vi "Periodic Tasks.vi"(8 "error in":errorcluster) -> ()   [LabVIEW 2023]
doc: "This VI runs in parallel to other tasks. It can contain as many user-defined periodic loops as you need. These can carry out PID or other sorts of timed response."
uses:
  <vilib>/Rock Robotics/WPI/DriverStation/WPI_DriverStationAllianceInfo.ctl
  <vilib>/Rock Robotics/WPI/DriverStation/WPI_DriverStationRobotMode2.ctl
  <vilib>/Rock Robotics/WPI/ThirdParty/JAS_Junk/TrajLib/TypeDef/TRANSLATION3D.ctl
  <vilib>/Rock Robotics/WPI/ThirdParty/JAS_Junk/TrajLib/TypeDef/POSE2D.ctl
  <vilib>/Rock Robotics/WPI/ThirdParty/JAS_Junk/TrajLib/TypeDef/TRANSLATION2D.ctl
  <vilib>/Rock Robotics/WPI/ThirdParty/JAS_Junk/TrajLib/TypeDef/ROTATION2D.ctl
  <vilib>/Rock Robotics/WPI/ThirdParty/JAS_Junk/TrajLib/TypeDef/X_Y_PAIR.ctl
  e9f6a02a-451a-49ef-b810-556ee57ecbaa.vi
  d07e73b9-761c-4664-be59-ebf116924375.vi
  <vilib>/Rock Robotics/WPI/ThirdParty/JAS_Junk/TrajLib/VI/BoolCmd_Recv_Internal.vi
  <vilib>/Rock Robotics/WPI/ThirdParty/JAS_Junk/TrajLib/VI/BoolCmd_Send_Internal.vi
  <vilib>/Rock Robotics/WPI/ThirdParty/JAS_Junk/TrajLib/VI/Util_GetTime_U32.vi
  <vilib>/Rock Robotics/WPI/ThirdParty/JAS_Junk/TrajLib/Translation2d_UnaryMinus.vi
  <vilib>/Rock Robotics/WPI/ThirdParty/JAS_Junk/TrajLib/Rotation2d_UnaryMinus.vi
  <vilib>/Rock Robotics/WPI/ThirdParty/JAS_Junk/TrajLib/Translation2d_RotateBy.vi
  <vilib>/Rock Robotics/WPI/ThirdParty/JAS_Junk/TrajLib/MathUtil_InputModulus.vi
  <vilib>/Rock Robotics/WPI/ThirdParty/JAS_Junk/TrajLib/Rotation2d_GetRadians.vi
  <vilib>/Rock Robotics/WPI/ThirdParty/JAS_Junk/TrajLib/MathUtil_Clamp.vi
  <vilib>/Rock Robotics/WPI/ThirdParty/JAS_Junk/TrajLib/VI/BoolCmd_ObtainQueue.vi
  <vilib>/Rock Robotics/WPI/ThirdParty/JAS_Junk/TrajLib/Rotation2d_CreateXY.vi
  <vilib>/Rock Robotics/WPI/Utilities/WPI_GetSetVariantRefNum.vi
  <vilib>/Rock Robotics/WPI/ThirdParty/JAS_Junk/TrajLib/VI/Util_GetTime_U64.vi
  <vilib>/Rock Robotics/Network Tables/NT Write Number.vi
  Swerve_Drive_System/SWERVE_DRIVE_GLOBALS.vi
  <vilib>/Rock Robotics/Network Tables/NT Read Numeric Array.vi
  <vilib>/Rock Robotics/Network Tables/NT Read String.vi
  Robot Global Data.vi
  <vilib>/Rock Robotics/Network Tables/NT Write String.vi
  <vilib>/Rock Robotics/Network Tables/NT Write Boolean.vi
  <vilib>/Rock Robotics/Network Tables/NT Write String Array.vi
  <vilib>/Rock Robotics/Network Tables/NT Write Numeric Array.vi
  <vilib>/addons/control/pid/pid.llb/PID Control Input Filter (DBL).vi
  <vilib>/Rock Robotics/Network Tables/NT Read String Array.vi
  <vilib>/Rock Robotics/Network Tables/NT Read Boolean.vi
  <vilib>/Rock Robotics/Network Tables/NT Read Number.vi
  <vilib>/gmath/interp.llb/Search Ordered Table.vi
  <vilib>/Rock Robotics/WPI/ThirdParty/Phoenix-LabVIEW/Motor Controller/Get/CTRE_Phoenix_MotorController_GetSelectedSensorData.vi
  <vilib>/Rock Robotics/WPI/ThirdParty/JAS_Junk/TrajLib/Trajectory_Library.lvlib
  <vilib>/Rock Robotics/WPI/ThirdParty/Phoenix-LabVIEW/Motor Controller/Controls/CTRE_Phoenix_MotorControl_ControlMode.ctl
  <vilib>/Rock Robotics/WPI/ThirdParty/JAS_Junk/TrajLib/Enum/DCMOTOR_TYPES_ENUM.ctl
  <vilib>/Rock Robotics/WPI/ThirdParty/REV Robotics/REVLib/Typedef/Spark MAX Control Type.ctl
  <vilib>/Rock Robotics/WPI/ThirdParty/Phoenix-LabVIEW/Motor Controller/Get/CTRE_Phoenix_MotorController_GetTemperature.vi
  <vilib>/Rock Robotics/WPI/ThirdParty/Phoenix-LabVIEW/CANdle/Controls/CTRE_Phoenix_CANdle_LEDColor.ctl
  <vilib>/addons/control/pid/NI_PID_pid.lvlib
  a548ba9f-81d9-431c-be79-d7e9cbcd1e66.vi
  <vilib>/Rock Robotics/WPI/ThirdParty/Phoenix-LabVIEW/Motor Controller/Controls/CTRE_Phoenix_MotorControl_NeutralMode.ctl
  <vilib>/Rock Robotics/Network Tables/NT Write Boolean Array.vi
  <vilib>/Rock Robotics/WPI/ThirdParty/Phoenix-LabVIEW/CANCoder/Get/CTRE_Phoenix_CANcoder_GetSensorData.vi
  <vilib>/Rock Robotics/Network Tables/NT Write Variant.vi
  <vilib>/Rock Robotics/Network Tables/NT Read Variant.vi
  <vilib>/Rock Robotics/WPI/ThirdParty/REV Robotics/REVLib/SubVI/Public/SPARK Get Device Status Applied Output.vi
  <vilib>/Rock Robotics/WPI/ThirdParty/REV Robotics/REVLib/SubVI/Public/SPARK Get Encoder Status Position.vi
  <vilib>/Rock Robotics/WPI/ThirdParty/REV Robotics/REVLib/SubVI/Public/SPARK Get Encoder Status Velocity.vi
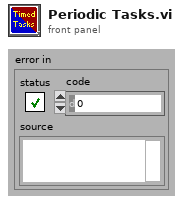
[diagram p1: front panel]
types:
  T1 = typedef "CTRE_Phoenix_CANdle_LEDColor.ctl" = cluster{"Red":u8, "Green":u8, "Blue":u8, "White":u8}
  T2 = typedef "WPI_DriverStationRobotMode2.ctl" = enum16{"Autonomous Disabled", "Autonomous Enabled", "Teleop Disabled", "Teleop Enabled", "Disconnected", "Finish", "Test Disabled", "Test Enabled", "Emergency Stopped"}
  T3 = typedef "CTRE_Phoenix_CANdle_DeviceRef.ctl" = cluster{"DeviceStatus":errorcluster, "Device Number":u8, "Handle":u64, "UsageFrame":u32, "Library Path":path}
  T4 = typedef "Trajectory_Library.lvlib/X_Y_PAIR.ctl" = cluster{"X":dbl, "Y":dbl}
  T5 = typedef "Trajectory_Library.lvlib/FUNCTION_GENERATOR.ctl" = cluster{"Table Xs":dbl[], "Table Ys":dbl[], "MinX":dbl, "MaxX":dbl, "ItemCount":i32}
  T6 = typedef "PathPlanner24.lvlib/PathPlannerEventMarker.ctl" = cluster{"WaypointRelativePos":dbl, "minimumTriggerDistance":dbl, "markerPos":T7, "lastRobotPos":T7, "Command":T8, "markerPos Exists":bool, "LastRobotPoseExists":bool, "Triggered":bool}
  T7 = typedef "Trajectory_Library.lvlib/TRANSLATION2D.ctl" = cluster{"X":dbl, "Y":dbl}
  T8 = typedef "PathPlanner24.lvlib/PathPlannerCommandUtil.ctl" = cluster{"waitTime":dbl, "name":string, "pathName":string, "commands":cluster{"type":T9, "waitTime":dbl, "name":string, "pathName":string}[], "type":T9}
  T9 = typedef "PathPlanner24.lvlib/PathPlanner_CommandUtilType_ENUM.ctl" = enum16{"Unknown", "Wait", "Named", "Path", "Sequential", "Parallel", "Race", "Deadline"}
  T10 = typedef "WPI_JoystickDevRef.ctl" = cluster{"Device":T11}
  T11 = typedef "WPI_JoystickDeviceEnum.ctl" = enum16{"USB 0", "USB 1", "USB 2", "USB 3", "USB 4", "USB 5"}
  T12 = typedef "Trajectory_Library.lvlib/SWERVE_DRIVE_KINEMATICS.ctl" = cluster{"NumModules":i32, "InverseKinematics":T13, "ForwardKinematics":T13, "Modules":T7[], "PrevCoR":T7, "SavedModuleStates":T14[]}
  T13 = typedef "NI_Matrix.lvlib/RealMatrix.ctl" = dbl[][]
  T14 = typedef "Trajectory_Library.lvlib/SWERVE_DRIVE_MODULE_STATE.ctl" = cluster{"Speed":dbl, "Angle":T15}
  T15 = typedef "Trajectory_Library.lvlib/ROTATION2D.ctl" = cluster{"VALUE":dbl, "COS":dbl, "SIN":dbl}
  T16 = typedef "Trajectory_Library.lvlib/SWERVE_DRIVE_ODOMETRY.ctl" = cluster{"POSE":T17, "GyroOffset":T15, "PreviousAngle":T15, "PrevModulePositions":T18[], "NumModules":i32}
  T17 = typedef "Trajectory_Library.lvlib/POSE2D.ctl" = cluster{"TRANSLATION":T7, "ROTATION":T15}
  T18 = typedef "Trajectory_Library.lvlib/SWERVE_DRIVE_MODULE_POSITION.ctl" = cluster{"Distance":dbl, "Angle":T15, "P":bool}
  T19 = typedef "Trajectory_Library.lvlib/SWERVE_DRIVE_POSE_EST2.ctl" = cluster{"M_Vision_K":T13, "m_nominal_dT":dbl, "m_PrevTime_Sec":dbl, "Pose_Buffer":T20, "Swerve_Drive_Kinematics":T12, "Swerve_Drive_Odom":T16, "M_Q":T13, "NumModules":i32}
  T20 = typedef "Trajectory_Library.lvlib/TIME_INTERPOLATABLE_VARIANT.ctl" = cluster{"TimeStamps":dbl[], "DataArray":variant[], "Min_TimeStamp":dbl, "Max_TimeStamp":dbl, "ItemCount":i32, "MaxBufferTime":dbl}
  T21 = typedef "Spark MAX Control Type.ctl" = enum16{"Percent VBus", "Voltage", "Velocity", "Position", "Smart Motion", "Current", "Smart Velocity", "MAXMotion Position", "MAXMotion Velocity"}
  T22 = typedef "Trajectory_Library.lvlib/DCMOTOR_TYPES_ENUM.ctl" = enum16{"CIM", "AndyMark 9015", "Andy Mark RS 775 125", "Bag", "BaneBots RS 550", "BaneBots RS 775", "Falcon 500", "Mini CIM", "NEO", "NEO 550", "Romi BuiltIn", "Vex 775 Pro", "Snow Blower AM 2235A", "Bosch Seat AM 3493", "Falcon 500 FOC", "Kraken X60", "Kraken X60 FOC", "NEO Vortex"}
  T23 = enum16{"DemandType_Neutral", "DemandType_AuxPID", "DemandType_ArbitraryFeedForward"}
  T24 = typedef "WPI_DriverStationAllianceInfo.ctl" = enum16{"Red", "Blue", "Invalid"}
  T25 = typedef "CTRE_Phoenix_MotorControl_NeutralMode.ctl" = enum8{"EEPROMSetting", "Override to Coast", "Override to Brake"}
  T26 = cluster{"proportional gain (Kp)":dbl, "integral time (Ki)":dbl, "derivative time (Kd)":dbl}
  T27 = typedef "WPI_MotorControlDeviceRef.ctl" = cluster{"DeviceStatus":errorcluster, "Type":T28, "PWM":cluster{"PWM Channel":T29, "DeadBand":T30}, "CAN":cluster{"Device Number":u8, "SetOutput VI Ref":variant, "GetOutput VI Ref":variant, "Enable VI Ref":variant, "Disable VI Ref":variant, "Data":variant}, "Invert":bool, "DIO PWM":cluster{"PWM \"Enable\" Channel":T29, "DIOChannel":T31, "PWM Rate":dbl}}
  T28 = typedef "WPI_MotorControlType.ctl" = enum16{"PWM", "CAN", "DIO PWM"}
  T29 = typedef "FPGA_DIOPWMChannel.ctl" = enum8{"PWM 0", "PWM 1", "PWM 2", "PWM 3", "PWM 4", "PWM 5", "PWM 6", "PWM 7", "PWM 8", "PWM 9", "PWM MXP 0", "PWM MXP 1", "PWM MXP 2", "PWM MXP 3", "PWM MXP 4", "PWM MXP 5", "PWM MXP 6", "PWM MXP 7", "PWM MXP 8", "PWM MXP 9", "Invalid"}
  T30 = typedef "WPI_PWMDeadband.ctl" = cluster{"Name":string, "maxPositivePwm":i32, "minPositivePwm":i32, "centerPwm":i32, "maxNegativePwm":i32, "minNegativePwm":i32, "angularRange":u16}
  T31 = typedef "FPGA_DIOChannel.ctl" = enum8{"DIO 0", "DIO 1", "DIO 2", "DIO 3", "DIO 4", "DIO 5", "DIO 6", "DIO 7", "DIO 8", "DIO 9", "DIO MXP 0", "DIO MXP 1", "DIO MXP 2", "DIO MXP 3", "DIO MXP 4", "DIO MXP 5", "DIO MXP 6", "DIO MXP 7", "DIO MXP 8", "DIO MXP 9", "DIO MXP 10", "DIO MXP 11", "DIO MXP 12", "DIO MXP 13", "DIO MXP 14", "DIO MXP 15", "SPI Port CS1", "SPI Port CS2", "SPI Port CS3", "SPI Port MISO", "SPI Port MOSI", "Invalid"}
  T32 = typedef "Trajectory_Library.lvlib/DCMOTOR.CTL" = cluster{"nominalVoltage_Volts":dbl, "StallTorque_NM":dbl, "StallCurrent_Amps":dbl, "FreeCurrent_Amps":dbl, "FreeSpeed_RadPerSec":dbl, "R_Ohms":dbl, "KvINV_RadPerSecPerVolt":dbl, "Kt_NMPerAmp":dbl, "L_H":dbl, "Jr_KgM2":dbl}
  T33 = typedef "Trajectory_Library.lvlib/SIMPLE_MOTOR_FF.ctl" = cluster{"Ks":dbl, "Kv":dbl, "Ka":dbl, "KnInv":dbl}
  T34 = typedef "CTRE_Phoenix_MotorControl_ControlMode.ctl" = u16
  T35 = typedef "CTRE_Phoenix_CANcoder_DeviceRef.ctl" = cluster{"DeviceStatus":errorcluster, "Device Number":u8, "Handle":u64, "UsageFrame":u32, "Library Path":path}
  T36 = typedef "WPI_SwitchDevRef.ctl" = cluster{"DevStatus":errorcluster, "DIO Channel":T31, "CntIndex":T37, "Normally Closed":bool}
  T37 = typedef "FPGA_CounterCtrSystemIndex.ctl" = enum8{"Ctr 0", "Ctr 1", "Ctr 2", "Ctr 3", "Ctr 4", "Ctr 5", "Ctr 6", "Ctr 7", "Invalid"}
  T38 = typedef "Trajectory_Library.lvlib/TRANSLATION3D.ctl" = cluster{"X":dbl, "Y":dbl, "Z":dbl}
  T39 = cluster{"CameraName":string, "TRANSLATION3D":T38, "Roll, Pitch, Yaw":cluster{"Roll  Degrees":dbl, "Pitch  Degrees":dbl, "Yaw  Degrees":dbl}}[]
  T40 = cluster{"Roll  Degrees":dbl, "Pitch  Degrees":dbl, "Yaw  Degrees":dbl}
  T41 = typedef "Trajectory_Library.lvlib/POSE3D.ctl" = cluster{"Translation3d":T38, "Rotation3d":T42}
  T42 = typedef "Trajectory_Library.lvlib/ROTATION3D.ctl" = cluster{"Q_quaternion":T43}
  T43 = typedef "Trajectory_Library.lvlib/QUATERNION.ctl" = cluster{"R":dbl, "V":dbl[]}
  T44 = cluster{"Future Proof Configs":bool, "MotorOutputInverted":u16, "MotorOutputNeutralMode":u16, "MotorOutputDutyCycleNeutralDeadband":dbl, "MotorOutputPeakForwardDutyCycle":dbl, "MotorOutputPeakReverseDutyCycle":dbl, "MotorOutputControlTimesyncFreqHz":dbl, "CurrentLimitsStatorCurrentLimit":dbl, "CurrentLimitsStatorCurrentLimitEnable":bool, "CurrentLimitsSupplyCurrentLimit":dbl, "CurrentLimitsSupplyCurrentLimitEnable":bool, "CurrentLimitsSupplyCurrentLowerLimit":dbl, "CurrentLimitsSupplyCurrentLowerTime":dbl, "VoltageSupplyVoltageTimeConstant":dbl, "VoltagePeakForwardVoltage":dbl, "VoltagePeakReverseVoltage":dbl, "TorqueCurrentPeakForwardTorqueCurrent":dbl, "TorqueCurrentPeakReverseTorqueCurrent":dbl, "TorqueCurrentTorqueNeutralDeadband":dbl, "FeedbackFeedbackRotorOffset":dbl, "FeedbackSensorToMechanismRatio":dbl, "FeedbackRotorToSensorRatio":dbl, "FeedbackFeedbackSensorSource":u16, "FeedbackFeedbackRemoteSensorID":i16, "FeedbackVelocityFilterTimeConstant":dbl, "DifferentialSensorsDifferentialSensorSource":u16, "DifferentialSensorsDifferentialTalonFXSensorID":i16, "DifferentialSensorsDifferentialRemoteSensorID":i16, "DifferentialConstantsPeakDifferentialDutyCycle":dbl, "DifferentialConstantsPeakDifferentialVoltage":dbl, "DifferentialConstantsPeakDifferentialTorqueCurrent":dbl, "OpenLoopRampsDutyCycleOpenLoopRampPeriod":dbl, "OpenLoopRampsVoltageOpenLoopRampPeriod":dbl, "OpenLoopRampsTorqueOpenLoopRampPeriod":dbl, "ClosedLoopRampsDutyCycleClosedLoopRampPeriod":dbl, "ClosedLoopRampsVoltageClosedLoopRampPeriod":dbl, "ClosedLoopRampsTorqueClosedLoopRampPeriod":dbl, "HardwareLimitSwitchForwardLimitType":u16, "HardwareLimitSwitchForwardLimitAutosetPositionEnable":bool, "HardwareLimitSwitchForwardLimitAutosetPositionValue":dbl, "HardwareLimitSwitchForwardLimitEnable":bool, "HardwareLimitSwitchForwardLimitSource":u16, "HardwareLimitSwitchForwardLimitRemoteSensorID":i16, "HardwareLimitSwitchReverseLimitType":u16, "HardwareLimitSwitchReverseLimitAutosetPositionEnable":bool, "HardwareLimitSwitchReverseLimitAutosetPositionValue":dbl, "HardwareLimitSwitchReverseLimitEnable":bool, "HardwareLimitSwitchReverseLimitSource":u16, "HardwareLimitSwitchReverseLimitRemoteSensorID":i16, "AudioBeepOnBoot":bool, "AudioBeepOnConfig":bool, "AudioAllowMusicDurDisable":bool, "SoftwareLimitSwitchForwardSoftLimitEnable":bool, "SoftwareLimitSwitchReverseSoftLimitEnable":bool, "SoftwareLimitSwitchForwardSoftLimitThreshold":dbl, "SoftwareLimitSwitchReverseSoftLimitThreshold":dbl, "MotionMagicMotionMagicCruiseVelocity":dbl, "MotionMagicMotionMagicAcceleration":dbl, "MotionMagicMotionMagicJerk":dbl, "MotionMagicMotionMagicExpo_kV":dbl, "MotionMagicMotionMagicExpo_kA":dbl, "CustomParamsCustomParam0":i16, "CustomParamsCustomParam1":i16, "ClosedLoopGeneralContinuousWrap":bool, "Slot0kP":dbl, "Slot0kI":dbl, "Slot0kD":dbl, "Slot0kS":dbl, "Slot0kV":dbl, "Slot0kA":dbl, "Slot0kG":dbl, "Slot0GravityType":u16, "Slot0StaticFeedforwardSign":u16, "Slot1kP":dbl, "Slot1kI":dbl, "Slot1kD":dbl, "Slot1kS":dbl, "Slot1kV":dbl, "Slot1kA":dbl, "Slot1kG":dbl, "Slot1GravityType":u16, "Slot1StaticFeedforwardSign":u16, "Slot2kP":dbl, "Slot2kI":dbl, "Slot2kD":dbl, "Slot2kS":dbl, "Slot2kV":dbl, "Slot2kA":dbl, "Slot2kG":dbl, "Slot2GravityType":u16, "Slot2StaticFeedforwardSign":u16}[]
  T45 = typedef "Trajectory_Library.lvlib/CHASSIS_SPEEDS.ctl" = cluster{"vX":dbl, "vY":dbl, "vOmega":dbl}
  T46 = typedef "Trajectory_Library.lvlib/TWIST2D.ctl" = cluster{"dX":dbl, "dY":dbl, "dTHETA":dbl}
  T47 = typedef "Trajectory_Library.lvlib/TRANSFORM2D.ctl" = cluster{"TRANSLATION":T7, "ROTATION":T15, "xF":bool}
  T48 = cluster{"Future Proof Configs":bool, "MotorOutputInverted":u16, "MotorOutputNeutralMode":u16, "MotorOutputDutyCycleNeutralDeadband":dbl, "MotorOutputPeakForwardDutyCycle":dbl, "MotorOutputPeakReverseDutyCycle":dbl, "MotorOutputControlTimesyncFreqHz":dbl, "CurrentLimitsStatorCurrentLimit":dbl, "CurrentLimitsStatorCurrentLimitEnable":bool, "CurrentLimitsSupplyCurrentLimit":dbl, "CurrentLimitsSupplyCurrentLimitEnable":bool, "CurrentLimitsSupplyCurrentLowerLimit":dbl, "CurrentLimitsSupplyCurrentLowerTime":dbl, "VoltageSupplyVoltageTimeConstant":dbl, "VoltagePeakForwardVoltage":dbl, "VoltagePeakReverseVoltage":dbl, "TorqueCurrentPeakForwardTorqueCurrent":dbl, "TorqueCurrentPeakReverseTorqueCurrent":dbl, "TorqueCurrentTorqueNeutralDeadband":dbl, "FeedbackFeedbackRotorOffset":dbl, "FeedbackSensorToMechanismRatio":dbl, "FeedbackRotorToSensorRatio":dbl, "FeedbackFeedbackSensorSource":u16, "FeedbackFeedbackRemoteSensorID":i16, "FeedbackVelocityFilterTimeConstant":dbl, "DifferentialSensorsDifferentialSensorSource":u16, "DifferentialSensorsDifferentialTalonFXSensorID":i16, "DifferentialSensorsDifferentialRemoteSensorID":i16, "DifferentialConstantsPeakDifferentialDutyCycle":dbl, "DifferentialConstantsPeakDifferentialVoltage":dbl, "DifferentialConstantsPeakDifferentialTorqueCurrent":dbl, "OpenLoopRampsDutyCycleOpenLoopRampPeriod":dbl, "OpenLoopRampsVoltageOpenLoopRampPeriod":dbl, "OpenLoopRampsTorqueOpenLoopRampPeriod":dbl, "ClosedLoopRampsDutyCycleClosedLoopRampPeriod":dbl, "ClosedLoopRampsVoltageClosedLoopRampPeriod":dbl, "ClosedLoopRampsTorqueClosedLoopRampPeriod":dbl, "HardwareLimitSwitchForwardLimitType":u16, "HardwareLimitSwitchForwardLimitAutosetPositionEnable":bool, "HardwareLimitSwitchForwardLimitAutosetPositionValue":dbl, "HardwareLimitSwitchForwardLimitEnable":bool, "HardwareLimitSwitchForwardLimitSource":u16, "HardwareLimitSwitchForwardLimitRemoteSensorID":i16, "HardwareLimitSwitchReverseLimitType":u16, "HardwareLimitSwitchReverseLimitAutosetPositionEnable":bool, "HardwareLimitSwitchReverseLimitAutosetPositionValue":dbl, "HardwareLimitSwitchReverseLimitEnable":bool, "HardwareLimitSwitchReverseLimitSource":u16, "HardwareLimitSwitchReverseLimitRemoteSensorID":i16, "AudioBeepOnBoot":bool, "AudioBeepOnConfig":bool, "AudioAllowMusicDurDisable":bool, "SoftwareLimitSwitchForwardSoftLimitEnable":bool, "SoftwareLimitSwitchReverseSoftLimitEnable":bool, "SoftwareLimitSwitchForwardSoftLimitThreshold":dbl, "SoftwareLimitSwitchReverseSoftLimitThreshold":dbl, "MotionMagicMotionMagicCruiseVelocity":dbl, "MotionMagicMotionMagicAcceleration":dbl, "MotionMagicMotionMagicJerk":dbl, "MotionMagicMotionMagicExpo_kV":dbl, "MotionMagicMotionMagicExpo_kA":dbl, "CustomParamsCustomParam0":i16, "CustomParamsCustomParam1":i16, "ClosedLoopGeneralContinuousWrap":bool, "Slot0kP":dbl, "Slot0kI":dbl, "Slot0kD":dbl, "Slot0kS":dbl, "Slot0kV":dbl, "Slot0kA":dbl, "Slot0kG":dbl, "Slot0GravityType":u16, "Slot0StaticFeedforwardSign":u16, "Slot1kP":dbl, "Slot1kI":dbl, "Slot1kD":dbl, "Slot1kS":dbl, "Slot1kV":dbl, "Slot1kA":dbl, "Slot1kG":dbl, "Slot1GravityType":u16, "Slot1StaticFeedforwardSign":u16, "Slot2kP":dbl, "Slot2kI":dbl, "Slot2kD":dbl, "Slot2kS":dbl, "Slot2kV":dbl, "Slot2kA":dbl, "Slot2kG":dbl, "Slot2GravityType":u16, "Slot2StaticFeedforwardSign":u16}
  T49 = typedef "DeviceReference.ctl" = cluster{"CANbus Name":string, "Device Encoding":u32, "Device Name":string}
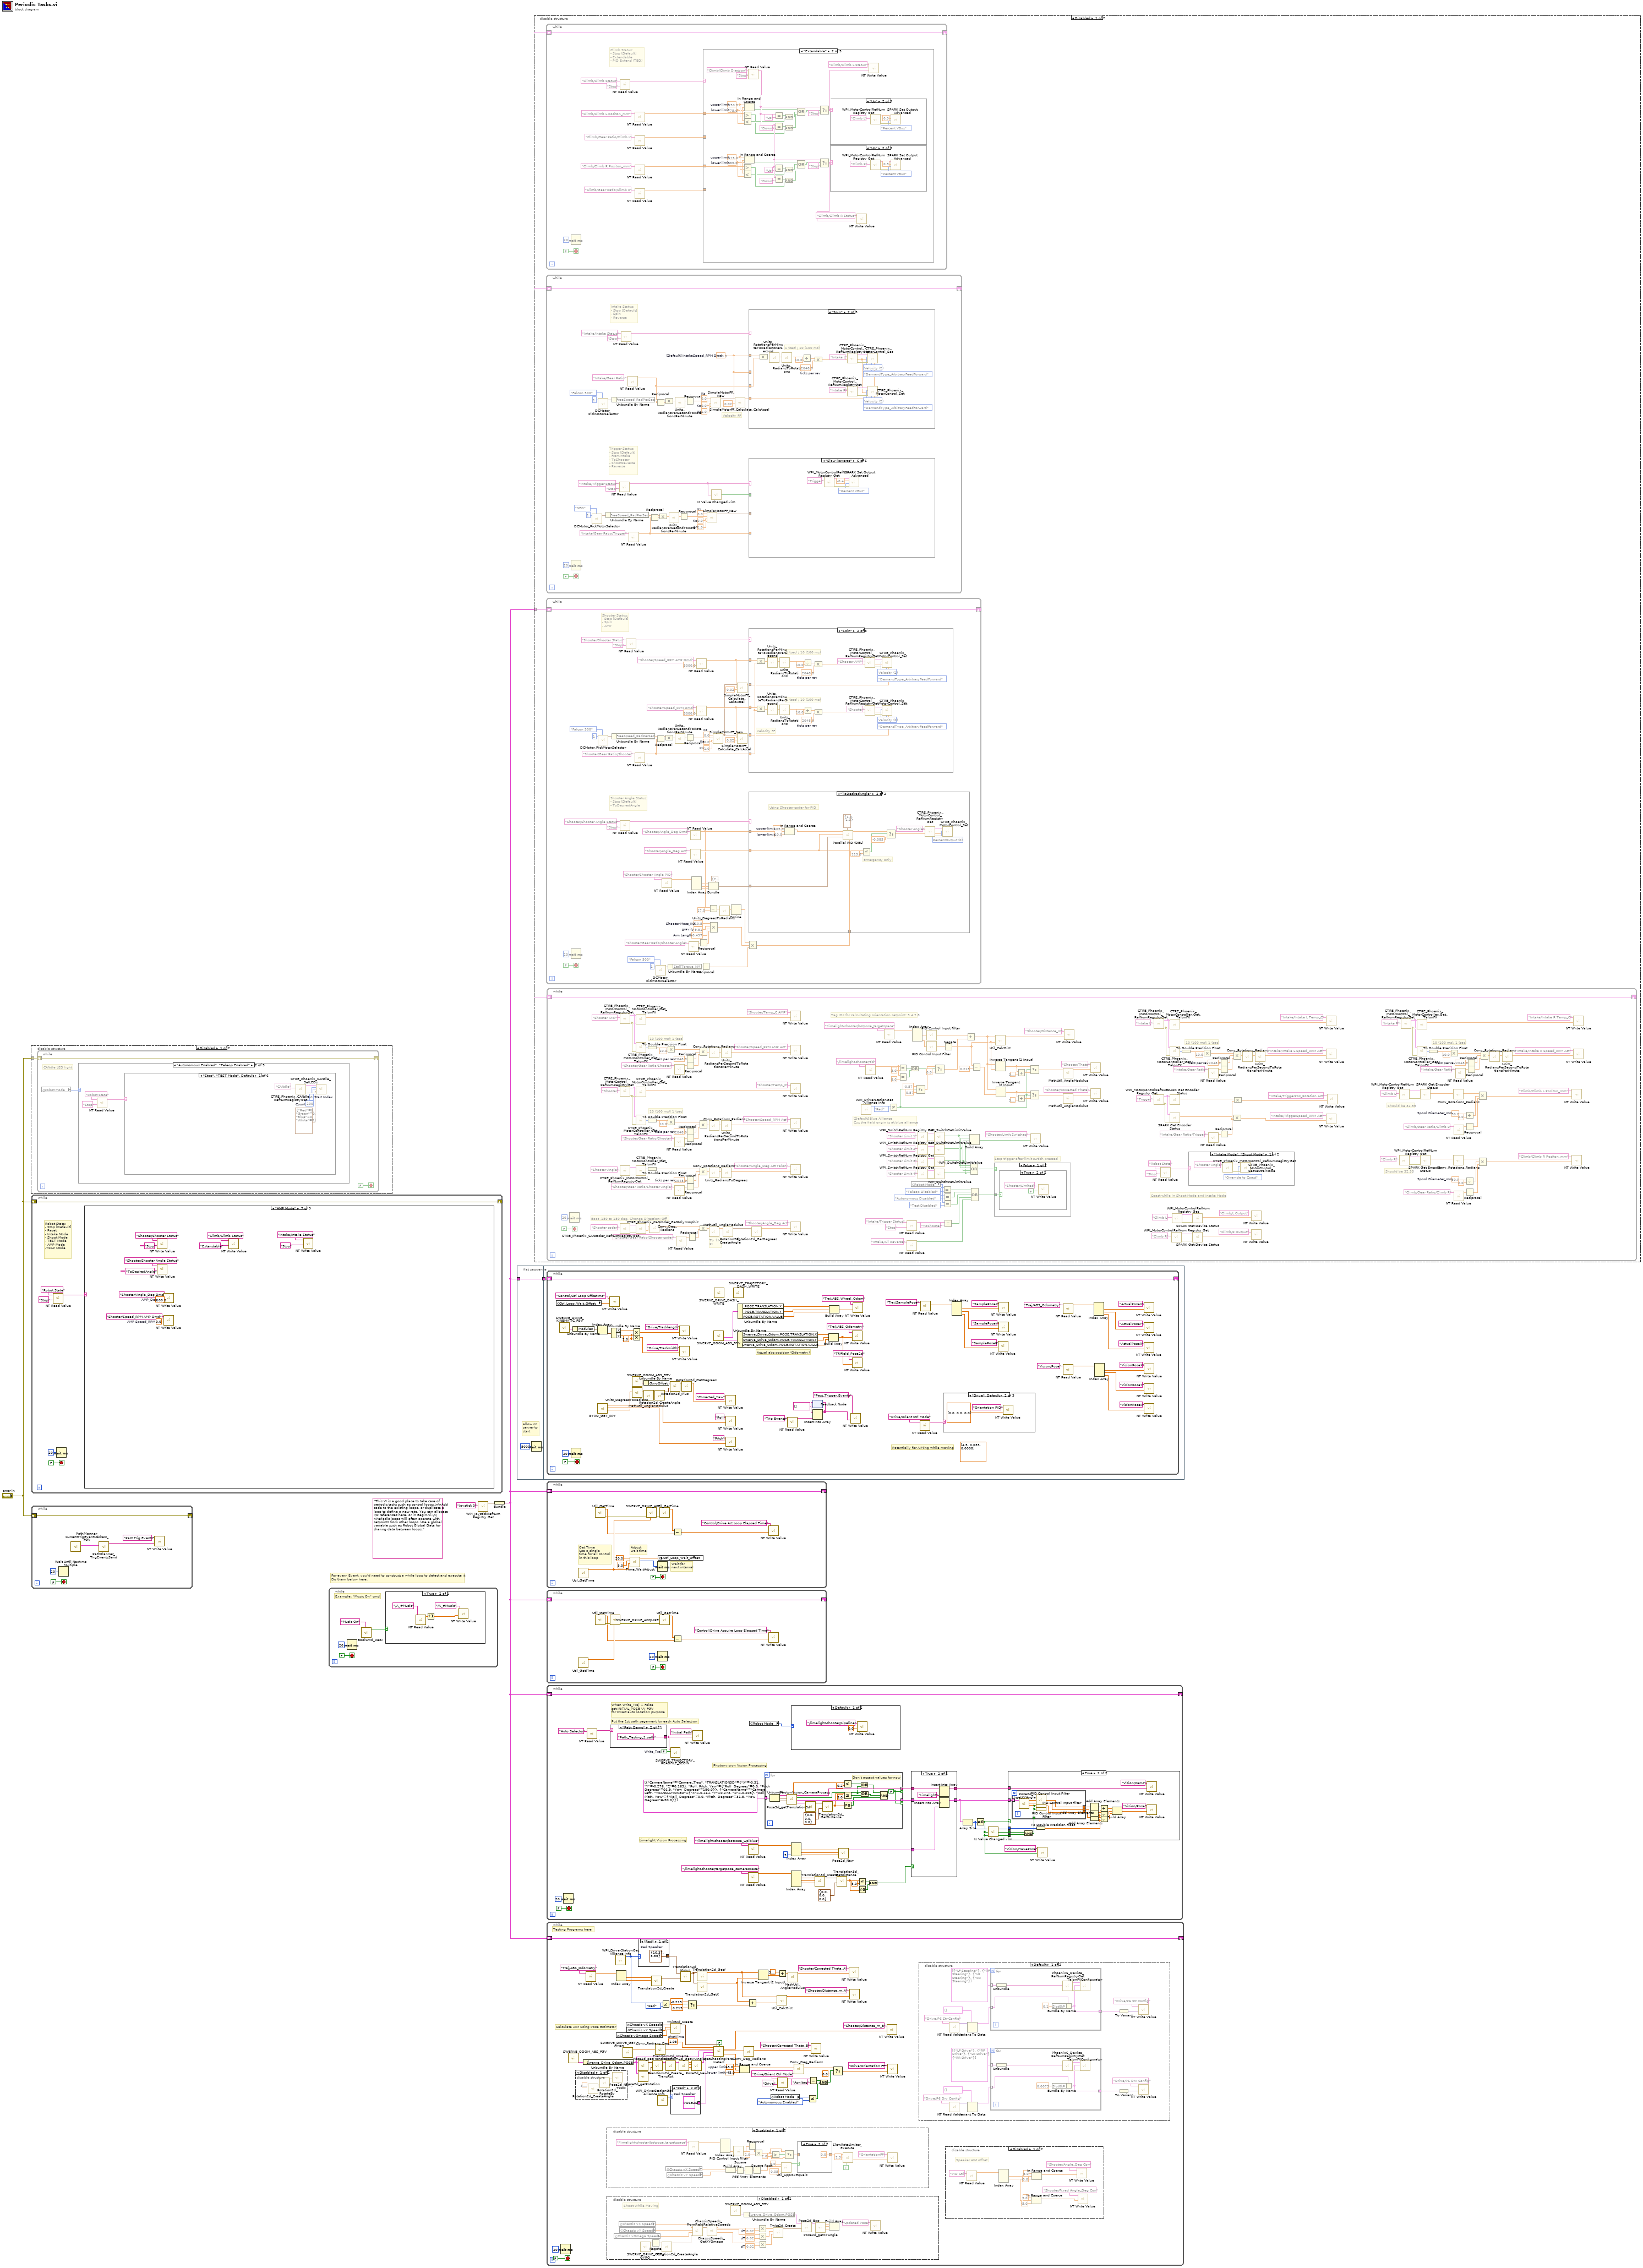
[diagram p0: block diagram]
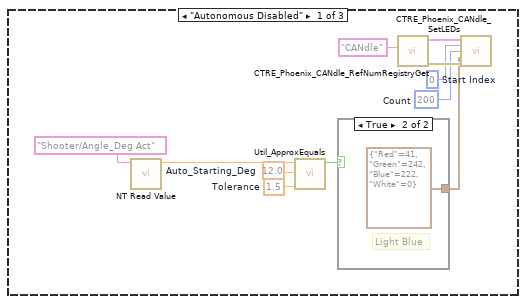
[diagram p2: hidden frame]
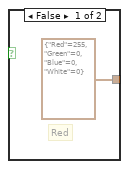
[diagram p3: hidden frame]
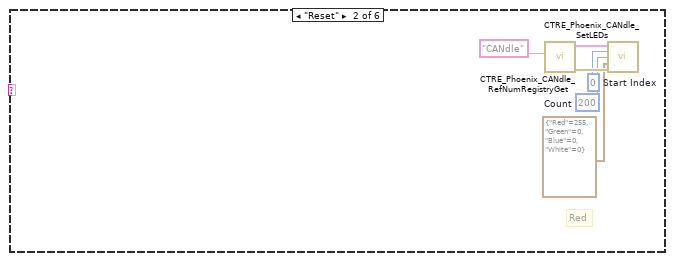
[diagram p4: hidden frame]
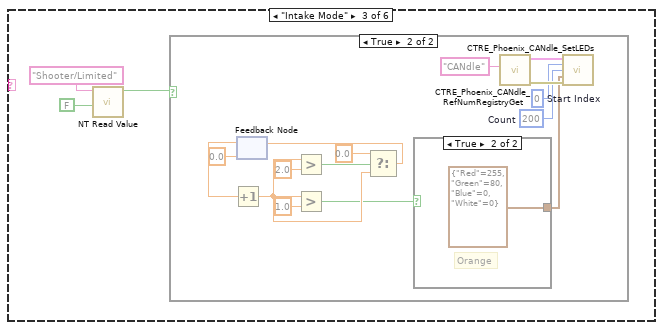
[diagram p5: hidden frame]
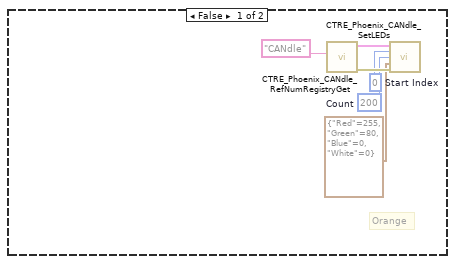
[diagram p6: hidden frame]
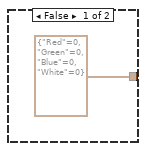
[diagram p7: hidden frame]
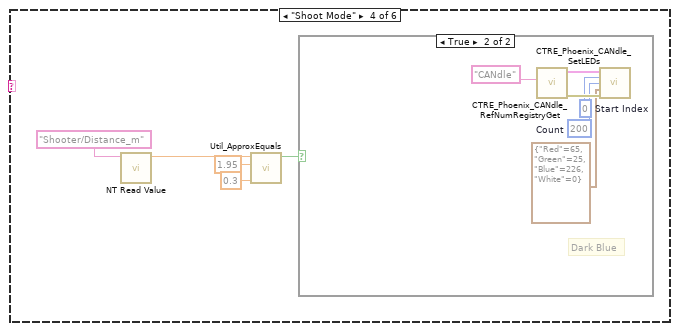
[diagram p8: hidden frame]
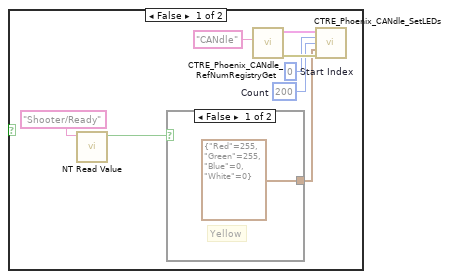
[diagram p9: hidden frame]
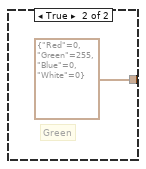
[diagram p10: hidden frame]
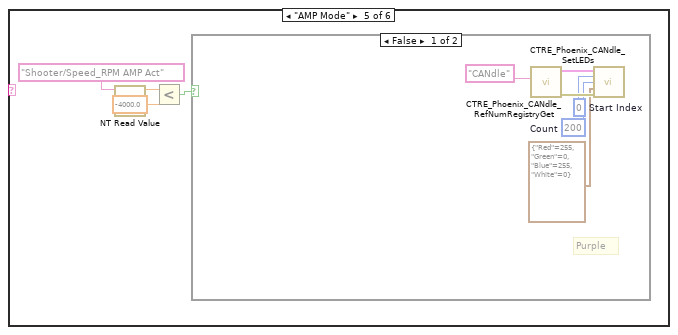
[diagram p11: hidden frame]
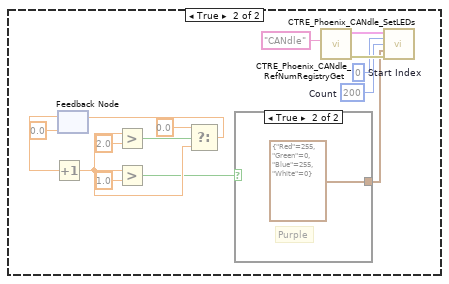
[diagram p12: hidden frame]
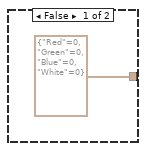
[diagram p13: hidden frame]
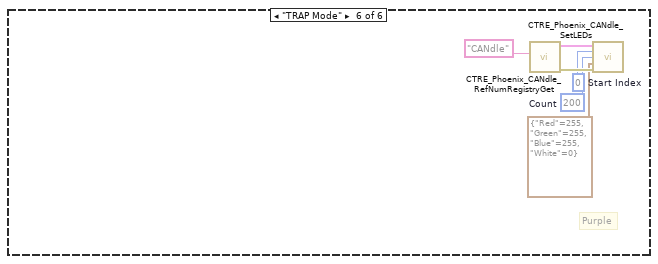
[diagram p14: hidden frame]
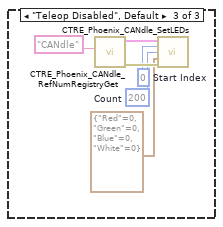
[diagram p15: hidden frame]
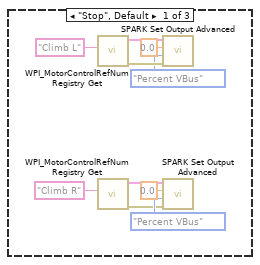
[diagram p18: hidden frame]
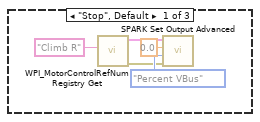
[diagram p19: hidden frame]
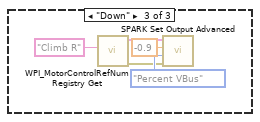
[diagram p20: hidden frame]
diagram:
  (unwired) "This VI is a good place to take care of periodic tasks such as control loops.\n\nAdd code to the existing loops, or duplicate a loop to define a new rate. You can allocate I/O references here, or in Begin.vi.\n\nPeriodic loops will often operate with setpoints from other loops. Use a global variable such as Robot Global Data for sharing data between loops."
  # "For every Event, you'd need to construct a while loop to detect and execute it\nDo them below here:"
  n1 = disable-structure shown="Disabled" {
    disable-tunnel: "error in" -> [w6 _]
    frame Disabled {
      n2 = while {
        shift-right: [w9] -> _
        shift-left: w6 -> [w9]
        stop <- FALSE stop-if-true
        # "CANdle LED light"
        n3 = global read "Robot Global Data.vi" "Robot Mode"() -> (w8:T2)
        n4 = case shown="\"Autonomous Enabled\", \"Teleop Enabled\"" w8 {
          frame "Autonomous Disabled" {
            w11 = 12.0  # Auto_Starting_Deg
            w13 = 1.5  # Tolerance
            w15 = 200  # Count
            w16 = 0  # Start Index
            n5 = call-poly <vilib>:"NT Read Value.vi"("name"="Shooter/Angle_Deg Act") -> ("value"=w12:dbl)  [unwired: 8 in, 2 out]
            n6 = call <vilib>:"Util_ApproxEquals.vi"("Tolerance"=w13, "Value 2"=w11, "Value 1"=w12) -> ("ApproxEquals"=w10:bool)  [unwired: 8 in]
            n7 = case shown="True" w10 {
              tunnel: [T1 {"Red"=255, "Green"=0, "Blue"=0, "White"=0} ("LED Color") T1 {"Red"=41, "Green"=242, "Blue"=222, "White"=0} ("LED Color")] -> w14
              frame False {
                # "Red"
              }
              frame True {
                # "Light Blue"
              }
            }
            n8 = call <vilib>:"CTRE_Phoenix_CANdle_RefNumRegistryGet.vi"("refnum name"="CANdle") -> ("error out"=w17:errorcluster, "CTRE_CANdle_DeviceRef"=w18:T3)  [unwired: 9 in]
            n9 = call <vilib>:"CTRE_Phoenix_CANdle_SetLEDs.vi"("CTRE_CANdle_DeviceRef"=w18, "Start Index"=w16, "Count"=w15, "LED Color"=w14, "error in"=w17) -> ()  [unwired: 9 in, 2 out]
          }
          frame "Autonomous Enabled", "Teleop Enabled" {
            n10 = call-poly <vilib>:"NT Read Value.vi"("default value"="Stop", "name"="Robot State") -> ("value"=w23:string)  [unwired: 7 in, 2 out]
            n11 = case shown="\"Stop\", \"TEST Mode\", Default" w23 {
              frame "Stop", "TEST Mode", Default {
                w27 = 200  # Count
                w28 = 0  # Start Index
                n12 = call <vilib>:"CTRE_Phoenix_CANdle_RefNumRegistryGet.vi"("refnum name"="CANdle") -> ("error out"=w29:errorcluster, "CTRE_CANdle_DeviceRef"=w30:T3)  [unwired: 9 in]
                n13 = call <vilib>:"CTRE_Phoenix_CANdle_SetLEDs.vi"("CTRE_CANdle_DeviceRef"=w30, "Start Index"=w28, "Count"=w27, "LED Color"=T1 {"Red"=0, "Green"=0, "Blue"=0, "White"=0}, "error in"=w29) -> ()  [unwired: 9 in, 2 out]
              }
              frame "Reset" {
                w33 = 200  # Count
                w34 = 0  # Start Index
                # "Red"
                n14 = call <vilib>:"CTRE_Phoenix_CANdle_RefNumRegistryGet.vi"("refnum name"="CANdle") -> ("error out"=w35:errorcluster, "CTRE_CANdle_DeviceRef"=w36:T3)  [unwired: 9 in]
                n15 = call <vilib>:"CTRE_Phoenix_CANdle_SetLEDs.vi"("CTRE_CANdle_DeviceRef"=w36, "Start Index"=w34, "Count"=w33, "LED Color"=T1 {"Red"=255, "Green"=0, "Blue"=0, "White"=0}, "error in"=w35) -> ()  [unwired: 9 in, 2 out]
              }
              frame "Intake Mode" {
                n16 = call-poly <vilib>:"NT Read Value.vi"("default value"=FALSE ("value"), "name"="Shooter/Limited") -> ("value"=w38:bool)  [unwired: 7 in, 2 out]
                n17 = case shown="True" w38 {
                  frame False {
                    w42 = 200  # Count
                    w43 = 0  # Start Index
                    # "Orange"
                    n18 = call <vilib>:"CTRE_Phoenix_CANdle_RefNumRegistryGet.vi"("refnum name"="CANdle") -> ("error out"=w44:errorcluster, "CTRE_CANdle_DeviceRef"=w45:T3)  [unwired: 9 in]
                    n19 = call <vilib>:"CTRE_Phoenix_CANdle_SetLEDs.vi"("CTRE_CANdle_DeviceRef"=w45, "Start Index"=w43, "Count"=w42, "LED Color"=T1 {"Red"=255, "Green"=80, "Blue"=0, "White"=0}, "error in"=w44) -> ()  [unwired: 9 in, 2 out]
                  }
                  frame True {
                    w57 = 200  # Count
                    w58 = 0  # Start Index
                    n20 = feedback #1(0.0) -> (w55:dbl)
                    n21 = Increment(x=w55) -> (x+1=w50:dbl)
                    n22 = Greater?(x=w50, y=2.0) -> (0:w48:bool)
                    n23 = Greater?(x=w50, y=1.0) -> (0:w47:bool)
                    n24 = Select(t=0.0, s=w48, f=w50) -> (s? t:f=w49:dbl)
                    n25 = feedback-in #1(w49) -> ()
                    n26 = case shown="True" w47 {
                      tunnel: [T1 {"Red"=0, "Green"=0, "Blue"=0, "White"=0} ("LED Color") T1 {"Red"=255, "Green"=80, "Blue"=0, "White"=0} ("LED Color")] -> w56
                      frame False {
                      }
                      frame True {
                        # "Orange"
                      }
                    }
                    n27 = call <vilib>:"CTRE_Phoenix_CANdle_RefNumRegistryGet.vi"("refnum name"="CANdle") -> ("error out"=w59:errorcluster, "CTRE_CANdle_DeviceRef"=w60:T3)  [unwired: 9 in]
                    n28 = call <vilib>:"CTRE_Phoenix_CANdle_SetLEDs.vi"("CTRE_CANdle_DeviceRef"=w60, "Start Index"=w58, "Count"=w57, "LED Color"=w56, "error in"=w59) -> ()  [unwired: 9 in, 2 out]
                  }
                }
              }
              frame "Shoot Mode" {
                n29 = call-poly <vilib>:"NT Read Value.vi"("name"="Shooter/Distance_m") -> ("value"=w67:dbl)  [unwired: 8 in, 2 out]
                n30 = call <vilib>:"Util_ApproxEquals.vi"("Tolerance"=0.3, "Value 2"=1.95, "Value 1"=w67) -> ("ApproxEquals"=w64:bool)  [unwired: 8 in]
                n31 = case shown="True" w64 {
                  frame False {
                    w72 = 200  # Count
                    w73 = 0  # Start Index
                    n32 = call-poly <vilib>:"NT Read Value.vi"("name"="Shooter/Ready") -> ("value"=w69:bool)  [unwired: 8 in, 2 out]
                    n33 = case shown="False" w69 {
                      tunnel: [T1 {"Red"=255, "Green"=255, "Blue"=0, "White"=0} ("LED Color") T1 {"Red"=0, "Green"=255, "Blue"=0, "White"=0} ("LED Color")] -> w71
                      frame False {
                        # "Yellow"
                      }
                      frame True {
                        # "Green"
                      }
                    }
                    n34 = call <vilib>:"CTRE_Phoenix_CANdle_RefNumRegistryGet.vi"("refnum name"="CANdle") -> ("error out"=w74:errorcluster, "CTRE_CANdle_DeviceRef"=w75:T3)  [unwired: 9 in]
                    n35 = call <vilib>:"CTRE_Phoenix_CANdle_SetLEDs.vi"("CTRE_CANdle_DeviceRef"=w75, "Start Index"=w73, "Count"=w72, "LED Color"=w71, "error in"=w74) -> ()  [unwired: 9 in, 2 out]
                  }
                  frame True {
                    w80 = 200  # Count
                    w81 = 0  # Start Index
                    # "Dark Blue"
                    n36 = call <vilib>:"CTRE_Phoenix_CANdle_RefNumRegistryGet.vi"("refnum name"="CANdle") -> ("error out"=w82:errorcluster, "CTRE_CANdle_DeviceRef"=w83:T3)  [unwired: 9 in]
                    n37 = call <vilib>:"CTRE_Phoenix_CANdle_SetLEDs.vi"("CTRE_CANdle_DeviceRef"=w83, "Start Index"=w81, "Count"=w80, "LED Color"=T1 {"Red"=65, "Green"=25, "Blue"=226, "White"=0}, "error in"=w82) -> ()  [unwired: 9 in, 2 out]
                  }
                }
              }
              frame "AMP Mode" {
                n38 = call-poly <vilib>:"NT Read Value.vi"("name"="Shooter/Speed_RPM AMP Act") -> ("value"=w86:dbl)  [unwired: 8 in, 2 out]
                n39 = Less?(x=w86, y=-4000.0) -> (x < y?=w87:bool)
                n40 = case shown="False" w87 {
                  frame False {
                    w90 = 200  # Count
                    w91 = 0  # Start Index
                    # "Purple"
                    n41 = call <vilib>:"CTRE_Phoenix_CANdle_RefNumRegistryGet.vi"("refnum name"="CANdle") -> ("error out"=w92:errorcluster, "CTRE_CANdle_DeviceRef"=w93:T3)  [unwired: 9 in]
                    n42 = call <vilib>:"CTRE_Phoenix_CANdle_SetLEDs.vi"("CTRE_CANdle_DeviceRef"=w93, "Start Index"=w91, "Count"=w90, "LED Color"=T1 {"Red"=255, "Green"=0, "Blue"=255, "White"=0}, "error in"=w92) -> ()  [unwired: 9 in, 2 out]
                  }
                  frame True {
                    w105 = 200  # Count
                    w106 = 0  # Start Index
                    n43 = feedback #2(0.0) -> (w103:dbl)
                    n44 = Increment(x=w103) -> (x+1=w98:dbl)
                    n45 = Greater?(x=w98, y=2.0) -> (0:w96:bool)
                    n46 = Greater?(x=w98, y=1.0) -> (0:w95:bool)
                    n47 = Select(t=0.0, s=w96, f=w98) -> (s? t:f=w97:dbl)
                    n48 = feedback-in #2(w97) -> ()
                    n49 = case shown="True" w95 {
                      tunnel: [T1 {"Red"=0, "Green"=0, "Blue"=0, "White"=0} ("LED Color") T1 {"Red"=255, "Green"=0, "Blue"=255, "White"=0} ("LED Color")] -> w104
                      frame False {
                      }
                      frame True {
                        # "Purple"
                      }
                    }
                    n50 = call <vilib>:"CTRE_Phoenix_CANdle_RefNumRegistryGet.vi"("refnum name"="CANdle") -> ("error out"=w107:errorcluster, "CTRE_CANdle_DeviceRef"=w108:T3)  [unwired: 9 in]
                    n51 = call <vilib>:"CTRE_Phoenix_CANdle_SetLEDs.vi"("CTRE_CANdle_DeviceRef"=w108, "Start Index"=w106, "Count"=w105, "LED Color"=w104, "error in"=w107) -> ()  [unwired: 9 in, 2 out]
                  }
                }
              }
              frame "TRAP Mode" {
                w113 = 200  # Count
                w114 = 0  # Start Index
                # "Purple"
                n52 = call <vilib>:"CTRE_Phoenix_CANdle_RefNumRegistryGet.vi"("refnum name"="CANdle") -> ("error out"=w115:errorcluster, "CTRE_CANdle_DeviceRef"=w116:T3)  [unwired: 9 in]
                n53 = call <vilib>:"CTRE_Phoenix_CANdle_SetLEDs.vi"("CTRE_CANdle_DeviceRef"=w116, "Start Index"=w114, "Count"=w113, "LED Color"=T1 {"Red"=255, "Green"=255, "Blue"=255, "White"=0}, "error in"=w115) -> ()  [unwired: 9 in, 2 out]
              }
            }
          }
          frame "Teleop Disabled", Default {
            w119 = 200  # Count
            w120 = 0  # Start Index
            n54 = call <vilib>:"CTRE_Phoenix_CANdle_RefNumRegistryGet.vi"("refnum name"="CANdle") -> ("error out"=w121:errorcluster, "CTRE_CANdle_DeviceRef"=w122:T3)  [unwired: 9 in]
            n55 = call <vilib>:"CTRE_Phoenix_CANdle_SetLEDs.vi"("CTRE_CANdle_DeviceRef"=w122, "Start Index"=w120, "Count"=w119, "LED Color"=T1 {"Red"=0, "Green"=0, "Blue"=0, "White"=0}, "error in"=w121) -> ()  [unwired: 9 in, 2 out]
          }
        }
      }
    }
    frame Enabled {
    }
  }
  n56 = while {
    shift-right: [w128] -> _
    shift-left: "error in" -> [w128]
    stop <- FALSE stop-if-true
    # "Robot State:\n- Stop [Default]\n- Reset\n- Intake Mode\n- Shoot Mode\n- TEST Mode\n- AMP Mode\n-TRAP Mode"
    n57 = call-poly <vilib>:"NT Read Value.vi"("default value"="Stop", "name"="Robot State") -> ("value"=w124:string)  [unwired: 7 in, 2 out]
    n58 = Wait (ms)(milliseconds to wait=u32 20) -> ()  [unwired: 1 out]
    n59 = case shown="\"AMP Mode\"" w124 {
      frame "Stop", Default {
        n60 = call-poly <vilib>:"NT Write Value.vi"("value"="Stop" ("default value"), "name"="Shooter/Shooter Status") -> ()  [unwired: 9 in, 1 out]
        n61 = call-poly <vilib>:"NT Write Value.vi"("value"="Stop" ("default value"), "name"="Shooter/Shooter Angle Status") -> ()  [unwired: 9 in, 1 out]
        n62 = call-poly <vilib>:"NT Write Value.vi"("value"="Stop" ("default value"), "name"="Climb/Climb Status") -> ()  [unwired: 9 in, 1 out]
        n63 = call-poly <vilib>:"NT Write Value.vi"("value"="Stop" ("default value"), "name"="Intake/Intake Status") -> ()  [unwired: 9 in, 1 out]
        n64 = call-poly <vilib>:"NT Write Value.vi"("value"="Stop" ("default value"), "name"="Intake/Trigger Status") -> ()  [unwired: 9 in, 1 out]
      }
      frame "Reset" {
        w142 = 12.0  # Reset_Deg
        n65 = global read "Robot Global Data.vi" "Robot Mode"() -> (w140:T2)
        n66 = case shown="\"Autonomous Disabled\", Default" w140 {
          frame "Autonomous Disabled", Default {
            n67 = call-poly <vilib>:"NT Write Value.vi"("value"="Stop" ("default value"), "name"="Shooter/Shooter Status") -> ()  [unwired: 9 in, 1 out]
          }
          frame "Autonomous Enabled" {
            n68 = call-poly <vilib>:"NT Write Value.vi"("value"="Spin" ("default value"), "name"="Shooter/Shooter Status") -> ()  [unwired: 9 in, 1 out]
          }
        }
        n69 = call-poly <vilib>:"NT Write Value.vi"("value"="ToDesiredAngle" ("default value"), "name"="Shooter/Shooter Angle Status") -> ()  [unwired: 9 in, 1 out]
        n70 = call-poly <vilib>:"NT Write Value.vi"("value"=w142, "name"="Shooter/Angle_Deg Dmd") -> ()  [unwired: 9 in, 1 out]
        n71 = call-poly <vilib>:"NT Write Value.vi"("value"="Extendable" ("default value"), "name"="Climb/Climb Status") -> ()  [unwired: 9 in, 1 out]
        n72 = call-poly <vilib>:"NT Write Value.vi"("value"="Stop" ("default value"), "name"="Intake/Intake Status") -> ()  [unwired: 9 in, 1 out]
        n73 = call-poly <vilib>:"NT Write Value.vi"("value"="Stop" ("default value"), "name"="Intake/Trigger Status") -> ()  [unwired: 9 in, 1 out]
      }
      frame "Intake Mode" {
        w155 = 17.0  # Intake_Deg
        n74 = call-poly <vilib>:"NT Write Value.vi"("value"="Extendable" ("default value"), "name"="Climb/Climb Status") -> ()  [unwired: 9 in, 1 out]
        n75 = call-poly <vilib>:"NT Write Value.vi"("value"="ToDesiredAngle" ("default value"), "name"="Shooter/Shooter Angle Status") -> ()  [unwired: 9 in, 1 out]
        n76 = call-poly <vilib>:"NT Read Value.vi"("name"="Intake/All Reverse") -> ("value"=w158:bool)  [unwired: 8 in, 2 out]
        n77 = global read "Robot Global Data.vi" "Robot Mode"() -> (w156:T2)
        n78 = case shown="False" w158 {
          frame False {
            n79 = call-poly <vilib>:"NT Read Value.vi"("default value"=FALSE ("value"), "name"="Shooter/Limited") -> ("value"=w176:bool)  [unwired: 7 in, 2 out]
            n80 = Select(t="Stop" ("default value"), s=w176, f="FromIntake" ("default value")) -> (s? t:f=w179:string)
            n81 = call-poly <vilib>:"NT Write Value.vi"("value"="Spin" ("default value"), "name"="Intake/Intake Status") -> ()  [unwired: 9 in, 1 out]
            n82 = call-poly <vilib>:"NT Write Value.vi"("value"=w179, "name"="Intake/Trigger Status") -> ()  [unwired: 9 in, 1 out]
          }
          frame True {
            n83 = call-poly <vilib>:"NT Write Value.vi"("value"="Reverse" ("default value"), "name"="Intake/Intake Status") -> ()  [unwired: 9 in, 1 out]
            n84 = call-poly <vilib>:"NT Write Value.vi"("value"="Reverse" ("default value"), "name"="Intake/Trigger Status") -> ()  [unwired: 9 in, 1 out]
          }
        }
        n85 = case shown="\"Autonomous Disabled\", Default" w156 {
          frame "Autonomous Disabled", Default {
            w164 = 3500.0  # Pre-accelerate RPM
            n86 = call-poly <vilib>:"NT Write Value.vi"("value"="Spin" ("default value"), "name"="Shooter/Shooter Status") -> ()  [unwired: 9 in, 1 out]
            n87 = call-poly <vilib>:"NT Write Value.vi"("value"=w164, "name"="Shooter/Speed_RPM AMP Dmd") -> ()  [unwired: 9 in, 1 out]
            n88 = call-poly <vilib>:"NT Write Value.vi"("value"=w164, "name"="Shooter/Speed_RPM Dmd") -> ()  [unwired: 9 in, 1 out]
          }
          frame "Autonomous Enabled" {
            w169 = 3500.0  # Pre-accelerate RPM
            n89 = call-poly <vilib>:"NT Write Value.vi"("value"="Spin" ("default value"), "name"="Shooter/Shooter Status") -> ()  [unwired: 9 in, 1 out]
            n90 = call-poly <vilib>:"NT Write Value.vi"("value"=w169, "name"="Shooter/Speed_RPM AMP Dmd") -> ()  [unwired: 9 in, 1 out]
            n91 = call-poly <vilib>:"NT Write Value.vi"("value"=w169, "name"="Shooter/Speed_RPM Dmd") -> ()  [unwired: 9 in, 1 out]
          }
        }
        n92 = call-poly <vilib>:"NT Write Value.vi"("value"=w155, "name"="Shooter/Angle_Deg Dmd") -> ()  [unwired: 9 in, 1 out]
      }
      frame "Shoot Mode" {
        w198 = 300.0  # Tolerance
        w223 = 2.75  # Tolerance
        w226 = 2.0  # Tolerance
        # "Overwrite Shooter Angle in Auto B2"
        # "stop shooter angle when firing note"
        n93 = global read "Robot Global Data.vi" "Robot Mode"() -> (w213:T2)
        n94 = call-poly <vilib>:"NT Read Value.vi"("name"="Drive/Orient Ctrl Mode") -> ("value"=w206:string)  [unwired: 8 in, 2 out]
        n95 = call-poly <vilib>:"NT Read Value.vi"("default value"=FALSE, "name"="Shooter/Fixed Angle") -> ("value"=w196:bool)  [unwired: 7 in, 2 out]
        n96 = call-poly <vilib>:"NT Read Value.vi"("default value"=FALSE ("value"), "name"="Shooter/Overwrite Angle") -> ("value"=w191:bool)  [unwired: 7 in, 2 out]
        n97 = global read "Robot Global Data.vi" "Robot Mode"() -> (w188:T2)
        n98 = Equal?(x=w213, y=WPI_DriverStationRobotMode2."Autonomous Enabled") -> (x = y?=w204:bool)
        n99 = Not Equal?(x=w206, y="Apriltag" ("default value")) -> (x != y?=w202:bool)
        n100 = call-poly <vilib>:"NT Write Value.vi"("value"="Spin" ("default value"), "name"="Shooter/Shooter Status") -> ()  [unwired: 9 in, 1 out]
        n101 = call-poly <vilib>:"NT Write Value.vi"("value"="ToDesiredAngle" ("default value"), "name"="Shooter/Shooter Angle Status") -> ()  [unwired: 9 in, 1 out]
        n102 = Not(x=w204) -> (.not. x?=w193:bool)
        n103 = Or(x=w202, y=w196) -> (x .or. y?=w203:bool)
        n104 = Or(x=w193, y=w191) -> (x .or. y?=w192:bool)
        n105 = Compound Arithmetic op=AND(w203, w192) -> (w190:bool)
        n106 = call-poly <vilib>:"NT Write Value.vi"("value"="Extendable" ("default value"), "name"="Climb/Climb Status") -> ()  [unwired: 9 in, 1 out]
        n107 = global read "Robot Global Data.vi" "Robot Mode"() -> (w215:T2)
        n108 = Not(x=w190) -> (.not. x?=w189:bool)
        n109 = call-poly <vilib>:"NT Read Value.vi"("default value"="Stop", "name"="Intake/Trigger Status") -> ("value"=w231:string)  [unwired: 7 in, 2 out]
        n110 = call-poly <vilib>:"NT Read Value.vi"("name"="Shooter/Angle_Deg Act") -> ("value"=w210:dbl)  [unwired: 8 in, 2 out]
        n111 = call-poly <vilib>:"NT Read Value.vi"("name"="Shooter/Angle_Deg Dmd") -> ("value"=w227:dbl)  [unwired: 8 in, 2 out]
        n112 = call-poly <vilib>:"NT Read Value.vi"("name"="Shooter/Speed_RPM AMP Dmd") -> ("value"=w199:dbl)  [unwired: 8 in, 2 out]
        n113 = call-poly <vilib>:"NT Read Value.vi"("name"="Shooter/Speed_RPM AMP Act") -> ("value"=w201:dbl)  [unwired: 8 in, 2 out]
        n114 = call-poly <vilib>:"NT Read Value.vi"("name"="Shooter/Corrected Theta_A") -> ("value"=w221:dbl)  [unwired: 8 in, 2 out]
        n115 = case shown="\"Autonomous Enabled\"" w215 {
          frame Default {
            n116 = call-poly <vilib>:"NT Write Value.vi"("value"="Stop" ("default value"), "name"="Intake/Intake Status") -> ()  [unwired: 9 in, 1 out]
          }
          frame "Autonomous Enabled" {
            # "For Autonomous, spin intake until note is into trigger"
            n117 = call-poly <vilib>:"NT Read Value.vi"("name"="Shooter/Limited") -> ("value"=w287:bool)  [unwired: 8 in, 2 out]
            n118 = Select(t="Stop" ("default value"), s=w287, f="Spin" ("default value")) -> (s? t:f=w290:string)
            n119 = call-poly <vilib>:"NT Write Value.vi"("value"=w290, "name"="Intake/Intake Status") -> ()  [unwired: 9 in, 1 out]
          }
        }
        n120 = Not Equal?(x=w231, y="ToShooter") -> (x != y?=w214:bool)
        n121 = Or(x=w204, y=w214) -> (x .or. y?=w187:bool)
        n122 = case shown="True" w190 {
          tunnel: [w253 w269] -> w211
          tunnel: w210 -> [w252 _]
          tunnel: w187 -> [w251 _]
          tunnel: w196 -> [_ w268]
          tunnel: w191 -> [_ w276]
          tunnel: w188 -> [w241 _]
          frame False {
            w258 = 5000.0  # Long Dist RPM
            w249 = 3500.0  # Short Dist RPM
            # "1.735"
            # "When in different distance, pick between two RPMs and regression equations"
            # "Shooter Angle AIM enabled"
            n123 = case shown="Default" w241 {
              tunnel: [w262 w265] -> w247
              frame "Autonomous Disabled", "Autonomous Enabled" {
                n124 = call-poly <vilib>:"NT Read Value.vi"("name"="Shooter/Distance_m") -> ("value"=w262:dbl)  [unwired: 8 in, 2 out]
              }
              frame Default {
                n125 = call-poly <vilib>:"NT Read Value.vi"("name"="Shooter/Distance_m_A") -> ("value"=w265:dbl)  [unwired: 8 in, 2 out]
              }
            }
            n126 = Greater?(x=w247, y=1.95) -> (0:w243:bool)
            n127 = Select(t=w258, s=w243, f=w249) -> (s? t:f=w250:dbl)
            n128 = Select(t=T4[] [{"X"=3.032472, "Y"=32.6}, {"X"=3.48178, "Y"=29.78}, {"X"=4.03953, "Y"=25.46}, {"X"=4.51023, "Y"=24.546}, {"X"=4.964, "Y"=22.922}, {"X"=5.5, "Y"=22.75}, {"X"=6.0, "Y"=20.5}, {"X"=2.730961, "Y"=33.428516}, {"X"=2.527363, "Y"=35.068359}, {"X"=2.30303, "Y"=36.386719}, {"X"=2.038037, "Y"=40.78125}, {"X"=3.132137, "Y"=31.025391}] ("X, Y Pairs"), s=w243, f=T4[] [{"X"=1.323346, "Y"=51.397656}, {"X"=1.517911, "Y"=48.867188}, {"X"=2.019133, "Y"=42.714844}] ("X, Y Pairs")) -> (s? t:f=w242:T4[])
            n129 = call <vilib>:"FunctionGenerator_New.vi"("X Y Pairs"=w242) -> ("FUNCTION_GENERATOR"=w248:T5)  [unwired: 10 in]
            n130 = call <vilib>:"FunctionGenerator_Calculate.vi"("Input Value"=w247, "FUNCTION_GENERATOR"=w248) -> ("Output Value"=w246:dbl)  [unwired: 9 in]
            n131 = call-poly <vilib>:"NT Read Value.vi"("default value"=0.0, "name"="Shooter/Angle_Deg Corr") -> ("value"=w256:dbl)  [unwired: 7 in, 2 out]
            n132 = call-poly <vilib>:"NT Write Value.vi"("value"=w250, "name"="Shooter/Speed_RPM AMP Dmd") -> ()  [unwired: 9 in, 1 out]
            n133 = call-poly <vilib>:"NT Write Value.vi"("value"=w250, "name"="Shooter/Speed_RPM Dmd") -> ()  [unwired: 9 in, 1 out]
            n134 = Add(x=w256, y=w246) -> (x+y=w254:dbl)
            n135 = Select(t=w254, s=w251, f=w252) -> (s? t:f=w253:dbl)
          }
          frame True {
            w280 = 12.5  # Reset_Deg
            w281 = 51.5  # Subwoofer_Deg
            # "Disable shooter angle AIM while in teleop if robot not auto-aiming or in fixed angle mode"
            n136 = call-poly <vilib>:"NT Read Value.vi"("name"="Shooter/Overwrite RPM") -> ("value"=w266:bool)  [unwired: 8 in, 2 out]
            n137 = case shown="False" w266 {
              tunnel: [w282 w283] -> w277
              frame False {
                w282 = 3250.0  # Fixed Deg RPM
              }
              frame True {
                n138 = call-poly <vilib>:"NT Read Value.vi"("name"="Shooter/RPM Dmd") -> ("value"=w283:dbl)  [unwired: 8 in, 2 out]
              }
            }
            n139 = Select(t=w281, s=w268, f=w280) -> (s? t:f=w275:dbl)
            n140 = call-poly <vilib>:"NT Read Value.vi"("name"="Shooter/Fixed Angle_Deg Corr") -> ("value"=w270:dbl)  [unwired: 8 in, 2 out]
            n141 = call-poly <vilib>:"NT Read Value.vi"("name"="Shooter/Angle_Deg Dmd") -> ("value"=w273:dbl)  [unwired: 8 in, 2 out]
            n142 = Select(t=w273, s=w276, f=w275) -> (s? t:f=w272:dbl)
            n143 = Add(x=w270, y=w272) -> (x+y=w269:dbl)
            n144 = call-poly <vilib>:"NT Write Value.vi"("value"=w277, "name"="Shooter/Speed_RPM AMP Dmd") -> ()  [unwired: 9 in, 1 out]
            n145 = call-poly <vilib>:"NT Write Value.vi"("value"=w277, "name"="Shooter/Speed_RPM Dmd") -> ()  [unwired: 9 in, 1 out]
          }
        }
        n146 = call "SWERVE_DRIVE_GET_GYRO.vi"() -> ("Gyro Heading Radians"=w220:dbl)  [unwired: 11 in]
        n147 = call <vilib>:"Units_DegreesToRadians.vi"("Degrees"=w223) -> ("Radians"=w224:dbl)  [unwired: 10 in]
        n148 = call <vilib>:"Util_ApproxEquals.vi"("Tolerance"=w226, "Value 2"=w227, "Value 1"=w210) -> ("ApproxEquals"=w219:bool)  [unwired: 8 in]
        n149 = call <vilib>:"Util_ApproxEquals.vi"("Tolerance"=w224, "Value 2"=w221, "Value 1"=w220) -> ("ApproxEquals"=w218:bool)  [unwired: 8 in]
        n150 = call <vilib>:"Util_ApproxEquals.vi"("Tolerance"=w198, "Value 2"=w201, "Value 1"=w199) -> ("ApproxEquals"=w197:bool)  [unwired: 8 in]
        n151 = Compound Arithmetic op=AND(w219, w197, w218, w189) -> (w216:bool)
        n152 = call-poly <vilib>:"NT Write Value.vi"("value"=w216, "name"="Shooter/Ready") -> ()  [unwired: 9 in, 1 out]
        n153 = call-poly <vilib>:"NT Write Value.vi"("value"=w211, "name"="Shooter/Angle_Deg Dmd") -> ()  [unwired: 9 in, 1 out]
      }
      frame "Reverse Mode" {
        w298 = -1900.0  # Trap RPM
        (unwired) "Shooter/Speed_RPM Dmd" ("name")
        (unwired) "Shooter/Speed_RPM AMP Dmd" ("name")
        n154 = call-poly <vilib>:"NT Read Value.vi"("name"="PID Ctrl") -> ("value"=w294:dbl[])  [unwired: 8 in, 2 out]
        n155 = Index Array(array=w294) -> (element=w293:dbl)  [unwired: 1 in]
        n156 = call-poly <vilib>:"NT Write Value.vi"("value"="Spin" ("default value"), "name"="Shooter/Shooter Status") -> ()  [unwired: 9 in, 1 out]
        n157 = call-poly <vilib>:"NT Write Value.vi"("value"="ToDesiredAngle" ("default value"), "name"="Shooter/Shooter Angle Status") -> ()  [unwired: 9 in, 1 out]
        n158 = call-poly <vilib>:"NT Write Value.vi"("value"=w298) -> ()  [unwired: 10 in, 1 out]
        n159 = call-poly <vilib>:"NT Write Value.vi"("value"=w298) -> ()  [unwired: 10 in, 1 out]
        n160 = call-poly <vilib>:"NT Write Value.vi"("value"=w293, "name"="Shooter/Angle_Deg Dmd") -> ()  [unwired: 9 in, 1 out]
        n161 = call-poly <vilib>:"NT Write Value.vi"("value"="Stop" ("default value"), "name"="Climb/Climb Status") -> ()  [unwired: 9 in, 1 out]
        n162 = call-poly <vilib>:"NT Write Value.vi"("value"="Slow Reverse", "name"="Intake/Trigger Status") -> ()  [unwired: 9 in, 1 out]
        n163 = call-poly <vilib>:"NT Write Value.vi"("value"="Stop" ("default value"), "name"="Intake/Intake Status") -> ()  [unwired: 9 in, 1 out]
      }
      frame "TEST Mode" {
        w308 = 5000.0  # Test Mode RPM
        w313 = TRUE  # AIM Calibration
        n164 = call-poly <vilib>:"NT Write Value.vi"("value"="Spin" ("default value"), "name"="Shooter/Shooter Status") -> ()  [unwired: 9 in, 1 out]
        n165 = call-poly <vilib>:"NT Write Value.vi"("value"="ToDesiredAngle" ("default value"), "name"="Shooter/Shooter Angle Status") -> ()  [unwired: 9 in, 1 out]
        n166 = case shown="True" w313 {
          frame False {
          }
          frame True {
            # "Angle to Shoot"
            # "Distance to Target"
            n167 = call-poly <vilib>:"NT Read Value.vi"("name"="Shooter/Data Reset") -> ("value"=w337:bool)  [unwired: 8 in, 2 out]
            n168 = call-poly <vilib>:"NT Read Value.vi"("name"="Shooter/Data Accept") -> ("value"=w326:bool)  [unwired: 8 in, 2 out]
            n169 = call-poly <vilib>:"NT Read Value.vi"("name"="Shooter/Distance_m") -> ("value"=w322:dbl)  [unwired: 8 in, 2 out]
            n170 = call-poly <vilib>:"NT Read Value.vi"("name"="Shooter/Angle_Deg Dmd") -> ("value"=w330:dbl)  [unwired: 8 in, 2 out]
            n171 = call "Is Value Changed.vim"("value"=w326) -> ("changed or first call?"=w336:bool)
            n172 = And(x=w326, y=w336) -> (x .and. y?=w335:bool)
            n173 = feedback #3(0.0) -> (w329:dbl)
            n174 = Select(t=w330, s=w335, f=w329) -> (s? t:f=w333:dbl)
            n175 = feedback-in #3(w333) -> ()
            n176 = call <vilib>:"Util_ApproxEquals.vi"("Tolerance"=1.0, "Value 2"=w329, "Value 1"=w330) -> ("ApproxEquals"=w324:bool)  [unwired: 8 in]
            n177 = Not(x=w324) -> (.not. x?=w327:bool)
            n178 = And(x=w326, y=w327) -> (x .and. y?=w325:bool)
            n179 = Build Array(w322, w330) -> (w332:dbl[])
            n180 = Build Array(w332) -> (w331:dbl[][])
            n181 = call "AIM_DataCollectAsCSV.vi"("Data Reset?"=w337, "WRITE"=w325, "in X, Y Data"=w331, "Data File Name"="AIM_Data_far.csv") -> ()  [unwired: 4 in, 4 out]
          }
        }
        n182 = call-poly <vilib>:"NT Write Value.vi"("value"="Extendable" ("default value"), "name"="Climb/Climb Status") -> ()  [unwired: 9 in, 1 out]
        n183 = call-poly <vilib>:"NT Read Value.vi"("name"="PID Ctrl") -> ("value"=w309:dbl[])  [unwired: 8 in, 2 out]
        n184 = Index Array(array=w309) -> ()  [unwired: 3 in, 3 out]
        n185 = call-poly <vilib>:"NT Write Value.vi"("value"="Spin" ("default value"), "name"="Intake/Intake Status") -> ()  [unwired: 9 in, 1 out]
        n186 = call-poly <vilib>:"NT Write Value.vi"("value"=w308, "name"="Shooter/Speed_RPM AMP Dmd") -> ()  [unwired: 9 in, 1 out]
        n187 = call-poly <vilib>:"NT Write Value.vi"("value"=w308, "name"="Shooter/Speed_RPM Dmd") -> ()  [unwired: 9 in, 1 out]
      }
      frame "AMP Mode" {
        w342 = 100.0  # AMP_Deg
        w344 = 0.0  # AMP Speed_RPM
        n188 = call-poly <vilib>:"NT Write Value.vi"("value"="Stop" ("default value"), "name"="Shooter/Shooter Status") -> ()  [unwired: 9 in, 1 out]
        n189 = call-poly <vilib>:"NT Write Value.vi"("value"="ToDesiredAngle" ("default value"), "name"="Shooter/Shooter Angle Status") -> ()  [unwired: 9 in, 1 out]
        n190 = call-poly <vilib>:"NT Write Value.vi"("value"=w342, "name"="Shooter/Angle_Deg Dmd") -> ()  [unwired: 9 in, 1 out]
        n191 = call-poly <vilib>:"NT Write Value.vi"("value"=w344, "name"="Shooter/Speed_RPM AMP Dmd") -> ()  [unwired: 9 in, 1 out]
        n192 = call-poly <vilib>:"NT Write Value.vi"("value"="Extendable" ("default value"), "name"="Climb/Climb Status") -> ()  [unwired: 9 in, 1 out]
        n193 = call-poly <vilib>:"NT Write Value.vi"("value"="Stop" ("default value"), "name"="Intake/Intake Status") -> ()  [unwired: 9 in, 1 out]
      }
      frame "TRAP Mode" {
        w354 = 1900.0  # Trap RPM
        w355 = 59.0  # AMP_Deg
        n194 = call-poly <vilib>:"NT Write Value.vi"("value"="Spin" ("default value"), "name"="Shooter/Shooter Status") -> ()  [unwired: 9 in, 1 out]
        n195 = call-poly <vilib>:"NT Write Value.vi"("value"="ToDesiredAngle" ("default value"), "name"="Shooter/Shooter Angle Status") -> ()  [unwired: 9 in, 1 out]
        n196 = call-poly <vilib>:"NT Write Value.vi"("value"=w354, "name"="Shooter/Speed_RPM AMP Dmd") -> ()  [unwired: 9 in, 1 out]
        n197 = call-poly <vilib>:"NT Write Value.vi"("value"=w354, "name"="Shooter/Speed_RPM Dmd") -> ()  [unwired: 9 in, 1 out]
        n198 = call-poly <vilib>:"NT Write Value.vi"("value"=w355, "name"="Shooter/Angle_Deg Dmd") -> ()  [unwired: 9 in, 1 out]
        n199 = call-poly <vilib>:"NT Write Value.vi"("value"="Extendable" ("default value"), "name"="Climb/Climb Status") -> ()  [unwired: 9 in, 1 out]
        n200 = call-poly <vilib>:"NT Write Value.vi"("value"="Stop" ("default value"), "name"="Intake/Intake Status") -> ()  [unwired: 9 in, 1 out]
      }
      frame "Calibrate Mode" {
        n201 = call-poly <vilib>:"NT Write Value.vi"("value"="Stop" ("default value"), "name"="Shooter/Shooter Status") -> ()  [unwired: 9 in, 1 out]
        n202 = call-poly <vilib>:"NT Write Value.vi"("value"="Calibrate" ("default value"), "name"="Shooter/Shooter Angle Status") -> ()  [unwired: 9 in, 1 out]
        n203 = call-poly <vilib>:"NT Write Value.vi"("value"="Stop" ("default value"), "name"="Climb/Climb Status") -> ()  [unwired: 9 in, 1 out]
        n204 = call-poly <vilib>:"NT Write Value.vi"("value"="Stop" ("default value"), "name"="Intake/Intake Status") -> ()  [unwired: 9 in, 1 out]
        n205 = call-poly <vilib>:"NT Write Value.vi"("value"="Stop" ("default value"), "name"="Intake/Trigger Status") -> ()  [unwired: 9 in, 1 out]
      }
    }
  }
  n206 = while {
    shift-right: [w381] -> _
    shift-left: "error in" -> [w381]
    stop <- FALSE stop-if-true
    n207 = Wait Until Next ms Multiple(millisecond multiple=u32 20) -> ()  [unwired: 1 out]
    n208 = call "PathPlanner_CurrentTrigEventMarkers_FGV.vi"() -> ("out EventMarkers"=w378:T6[])  [unwired: 11 in]
    n209 = call "PathPlanner_TrigEventsSend.vi"("Current Trig Events"=w378) -> ("Past Trig Events"=w379:string[])  [unwired: 9 in, 1 out]
    n210 = call-poly <vilib>:"NT Write Value.vi"("value"=w379, "name"="Past Trig Events") -> ()  [unwired: 9 in, 1 out]
  }
  n211 = while {
    stop <- FALSE stop-if-true
    # "Example: \"Music On\" cmd"
    n212 = Wait (ms)(milliseconds to wait=u32 20 ("millisecond multiple")) -> ()  [unwired: 1 out]
    n213 = call <vilib>:"BoolCmd_Recv.vi"("Command Name"="Music On") -> ("New Request"=w383:bool)  [unwired: 9 in, 1 out]
    n214 = case shown="True" w383 {
      frame False {
      }
      frame True {
        n215 = call-poly <vilib>:"NT Read Value.vi"("name"="/A_#Music") -> ("value"=w388:dbl)  [unwired: 8 in, 2 out]
        n216 = Increment(x=w388) -> (x+1=w387:dbl)
        n217 = call-poly <vilib>:"NT Write Value.vi"("value"=w387, "name"="/A_#Music") -> ()  [unwired: 9 in, 1 out]
      }
    }
  }
  n218 = call <vilib>:"WPI_JoystickRefNum Registry Get.vi"("refnum name"="Joystick 0") -> ("JoystickDevRef"=w4:T10)  [unwired: 1 in, 9 out]
  n219 = Bundle("JoystickDevRef"=w4) -> (w1:cluster{"JoystickDevRef":T10})  [unwired: 1 out]
  n220 = flat-sequence {
    tunnel: w1 -> [w392]
    tunnel: [w392] -> w3
    tunnel: w3 -> [w393]
    frame #0 {
      # "allow nt\nserver to \nstart"
      n221 = Wait (ms)(milliseconds to wait=u32 5000) -> ()  [unwired: 1 out]
    }
    frame #1 {
      n222 = while {
        shift-right: [w465] -> _
        shift-left: w393 -> [w465]
        stop <- FALSE stop-if-true
        (unwired) dbl[] [4.5, 0.035, 0.0008] ("value")
        w451 = 2.0 ("y")
        # "Potentially for AIMing while moving"
        # "Actual abs position (Odometry)"
        n223 = global read "Robot Global Data.vi" "Ctrl_Loop_Wait_Offset"() -> (w462:dbl)
        n224 = call "SWERVE_DRIVE_KINEMATIC_FGV.vi"() -> ("out SWERVE_DRIVE_KINEMATICS"=w448:T12)  [unwired: 11 in]
        n225 = Wait (ms)(milliseconds to wait=u32 20) -> ()  [unwired: 1 out]
        n226 = Unbundle By Name(w448) -> ("Modules"=w447:T7[])
        n227 = Index Array(array=w447) -> (element=w446:T7)  [unwired: 1 in]
        n228 = call "GYRO_GET_RPY.vi"() -> ("Yaw_Deg"=w394:dbl, "Pitch_Deg"=w395:dbl, "Roll_Deg"=w396:dbl)  [unwired: 9 in]
        n229 = call-poly <vilib>:"NT Write Value.vi"("value"=w462, "name"="Control/Ctrl Loop Offset ms" ("Name")) -> ()  [unwired: 9 in, 1 out]
        n230 = Unbundle By Name(w446) -> ("X"=w453:dbl, "Y"=w452:dbl)
        n231 = Multiply(x=w453, y=w451) -> (x*y=w449:dbl)
        n232 = Multiply(x=w452, y=w451) -> (x*y=w450:dbl)
        n233 = call "SWERVE_ODOM_ABS_FGV.vi"() -> ("out SWERVE_DRIVE_ODOMETRY"=w417:T16)  [unwired: 10 in, 1 out]
        n234 = call <vilib>:"Units_DegreesToRadians.vi"("Degrees"=w394) -> ("Radians"=w421:dbl)  [unwired: 10 in]
        n235 = Unbundle By Name(w417) -> ("GyroOffset"=w422:T15)
        n236 = call <vilib>:"MathUtil_AngleModulus.vi"("InputAngle"=w421) -> ("ModulsAngle"=w420:dbl)  [unwired: 10 in]
        n237 = call <vilib>:"Rotation2d_CreateAngle.vi"("Angle"=w420) -> ("ROTATION"=w419:T15)  [unwired: 10 in]
        n238 = call <vilib>:"Rotation2d_Plus.vi"("other ROTATION"=w419, "in ROTATION"=w422) -> ("out ROTATION"=w418:T15)  [unwired: 9 in]
        n239 = call-poly <vilib>:"NT Write Value.vi"("value"=w449, "name"="Drive/Tracklength" ("Name")) -> ()  [unwired: 9 in, 1 out]
        n240 = call-poly <vilib>:"NT Write Value.vi"("value"=w450, "name"="Drive/Trackwidth" ("Name")) -> ()  [unwired: 9 in, 1 out]
        n241 = call <vilib>:"Rotation2d_GetDegrees.vi"("in ROTATION"=w418) -> ("AngleDegrees"=w416:dbl)  [unwired: 10 in]
        n242 = call "SWERVE_ODOM_ABS_FGV.vi"() -> ("out SWERVE_DRIVE_POSE_EST2"=w429:T19, "out SWERVE_DRIVE_ODOMETRY"=w414:T16)  [unwired: 10 in]
        n243 = call "SWERVE_DRIVE_DASH_WRITE.vi"() -> ()  [unwired: 12 in]
        n244 = call-poly <vilib>:"NT Write Value.vi"("value"=w416, "name"="Corrected_Yaw" ("Name")) -> ()  [unwired: 9 in, 1 out]
        n245 = call-poly <vilib>:"NT Write Value.vi"("value"=w396, "name"="Roll" ("Name")) -> ()  [unwired: 9 in, 1 out]
        n246 = call-poly <vilib>:"NT Write Value.vi"("value"=w395, "name"="Pitch" ("Name")) -> ()  [unwired: 9 in, 1 out]
        n247 = call "SWERVE_TRAJECTORY_DASH_WRITE.vi"() -> ()  [unwired: 12 in]
        n248 = Unbundle By Name(w429) -> ("Swerve_Drive_Odom.POSE.TRANSLATION.X"=w459:dbl, "Swerve_Drive_Odom.POSE.TRANSLATION.Y"=w460:dbl, "Swerve_Drive_Odom.POSE.ROTATION.VALUE"=w461:dbl)
        n249 = Unbundle By Name(w414) -> ("POSE.TRANSLATION.X"=w411:dbl, "POSE.TRANSLATION.Y"=w410:dbl, "POSE.ROTATION.VALUE"=w409:dbl)
        n250 = call-poly <vilib>:"NT Read Value.vi"("name"="Trig Events") -> ("value"=w427:string[])  [unwired: 8 in, 2 out]
        n251 = feedback #4(string[] []) -> (w426:string[])
        n252 = Insert Into Array(array=w426, new element=w427) -> (w424:string[])  [unwired: 1 in]
        n253 = feedback-in #4(w424) -> ()
        n254 = Build Array(w459, w460, w461) -> (w397:dbl[])
        n255 = Build Array(w411, w410, w409) -> (w412:dbl[])
        n256 = call-poly <vilib>:"NT Write Value.vi"("value"=w424, "name"="Past_Trigger_Events") -> ()  [unwired: 9 in, 1 out]
        n257 = call-poly <vilib>:"NT Write Value.vi"("value"=w397, "name"="Traj/ABS_Odometry" ("Name")) -> ()  [unwired: 9 in, 1 out]
        n258 = call-poly <vilib>:"NT Write Value.vi"("value"=w397, "name"="TF/Field_Pose2d" ("Name")) -> ()  [unwired: 9 in, 1 out]
        n259 = call-poly <vilib>:"NT Write Value.vi"("value"=w412, "name"="Traj/ABS_Wheel_Odom" ("Name")) -> ()  [unwired: 9 in, 1 out]
        n260 = call-poly <vilib>:"NT Read Value.vi"("name"="Drive/Orient Ctrl Mode") -> ("value"=w407:string)  [unwired: 8 in, 2 out]
        n261 = call-poly <vilib>:"NT Read Value.vi"("name"="Traj/SamplePose" ("Name")) -> ("value"=w443:dbl[])  [unwired: 8 in, 2 out]
        n262 = case shown="\"Drive\", Default" w407 {
          frame "Note" {
            n263 = call-poly <vilib>:"NT Write Value.vi"("value"=dbl[] [2.5, 0.003, 0.06], "name"="Orientation PID") -> ()  [unwired: 9 in, 1 out]
          }
          frame "Drive", Default {
            n264 = call-poly <vilib>:"NT Write Value.vi"("value"=dbl[] [0.0, 0.0, 0.0], "name"="Orientation PID") -> ()  [unwired: 9 in, 1 out]
          }
          frame "Apriltag" {
            n265 = call-poly <vilib>:"NT Write Value.vi"("value"=dbl[] [2.5, 0.0075, 0.0], "name"="Orientation PID") -> ()  [unwired: 9 in, 1 out]
          }
        }
        n266 = Index Array(array=w443) -> (element #1=w439:dbl, element #2=w436:dbl, element #3=w432:dbl)  [unwired: 3 in]
        n267 = call-poly <vilib>:"NT Write Value.vi"("value"=w432, "name"="SamplePoseR" ("Name")) -> ()  [unwired: 9 in, 1 out]
        n268 = call-poly <vilib>:"NT Write Value.vi"("value"=w439, "name"="SamplePoseX" ("Name")) -> ()  [unwired: 9 in, 1 out]
        n269 = call-poly <vilib>:"NT Write Value.vi"("value"=w436, "name"="SamplePoseY" ("Name")) -> ()  [unwired: 9 in, 1 out]
        n270 = call-poly <vilib>:"NT Read Value.vi"("name"="Traj/ABS_Odometry" ("Name")) -> ("value"=w442:dbl[])  [unwired: 8 in, 2 out]
        n271 = call-poly <vilib>:"NT Read Value.vi"("name"="Vision/Pose" ("Name")) -> ("value"=w400:dbl[])  [unwired: 8 in, 2 out]
        n272 = Index Array(array=w442) -> (element #1=w438:dbl, element #2=w434:dbl, element #3=w430:dbl)  [unwired: 3 in]
        n273 = Index Array(array=w400) -> (element #1=w402:dbl, element #2=w404:dbl, element #3=w406:dbl)  [unwired: 3 in]
        n274 = call-poly <vilib>:"NT Write Value.vi"("value"=w438, "name"="ActualPoseX" ("Name")) -> ()  [unwired: 9 in, 1 out]
        n275 = call-poly <vilib>:"NT Write Value.vi"("value"=w434, "name"="ActualPoseY" ("Name")) -> ()  [unwired: 9 in, 1 out]
        n276 = call-poly <vilib>:"NT Write Value.vi"("value"=w430, "name"="ActualPoseR" ("Name")) -> ()  [unwired: 9 in, 1 out]
        n277 = call-poly <vilib>:"NT Write Value.vi"("value"=w402, "name"="VisionPoseX" ("Name")) -> ()  [unwired: 9 in, 1 out]
        n278 = call-poly <vilib>:"NT Write Value.vi"("value"=w404, "name"="VisionPoseY" ("Name")) -> ()  [unwired: 9 in, 1 out]
        n279 = call-poly <vilib>:"NT Write Value.vi"("value"=w406, "name"="VisionPoseR" ("Name")) -> ()  [unwired: 9 in, 1 out]
      }
    }
  }
  n280 = disable-structure shown="Disabled" {
    disable-tunnel: w1 -> [w473 _]
    frame Disabled {
      n281 = while {
        shift-right: [w485] -> _
        shift-left: w473 -> [w485]
        stop <- FALSE stop-if-true
        # "Climb Status:\n- Stop [Default]\n- Extendable\n- PID Extend (TBD)"
        n282 = Wait (ms)(milliseconds to wait=u32 20) -> ()  [unwired: 1 out]
        n283 = call-poly <vilib>:"NT Read Value.vi"("default value"="Stop", "name"="Climb/Climb Status") -> ("value"=w483:string)  [unwired: 7 in, 2 out]
        n284 = call-poly <vilib>:"NT Read Value.vi"("name"="Climb/Climb L Positon_mm") -> ("value"=w475:dbl)  [unwired: 8 in, 2 out]
        n285 = call-poly <vilib>:"NT Read Value.vi"("name"="Climb/Gear Ratio/Climb L") -> ("value"=w481:dbl)  [unwired: 8 in, 2 out]
        n286 = call-poly <vilib>:"NT Read Value.vi"("name"="Climb/Climb R Positon_mm") -> ("value"=w476:dbl)  [unwired: 8 in, 2 out]
        n287 = call-poly <vilib>:"NT Read Value.vi"("name"="Climb/Gear Ratio/Climb R") -> ("value"=w479:dbl)  [unwired: 8 in, 2 out]
        n288 = case shown="\"Extendable\"" w483 {
          tunnel: w481 -> [_ _ _]
          tunnel: w479 -> [_ _ _]
          tunnel: w475 -> [_ w530 w580]
          tunnel: w476 -> [_ w529 w564]
          frame "Stop", Default {
            n289 = call <vilib>:"WPI_MotorControlRefNum Registry Get.vi"("refnum name"="Climb L") -> ("error out"=w497:errorcluster, "MotorControlDevRef"=w496:T27)  [unwired: 9 in]
            n290 = call <vilib>:"WPI_MotorControlRefNum Registry Get.vi"("refnum name"="Climb R") -> ("error out"=w488:errorcluster, "MotorControlDevRef"=w489:T27)  [unwired: 9 in]
            n291 = call <vilib>:"SPARK Set Output Advanced.vi"("error in (no error)"=w497, "Control Mode"=Spark_MAX_Control_Type."Percent VBus", "Setpoint"=0.0 ("t"), "MotorControlDevRef"=w496) -> ()  [unwired: 6 in, 2 out]
            n292 = call <vilib>:"SPARK Set Output Advanced.vi"("error in (no error)"=w488, "Control Mode"=Spark_MAX_Control_Type."Percent VBus", "Setpoint"=0.0 ("t"), "MotorControlDevRef"=w489) -> ()  [unwired: 6 in, 2 out]
          }
          frame "Extendable" {
            w512 = 175.0  # upper limit
            w513 = -85.0  # lower limit
            w517 = 150.0  # upper limit
            w516 = -75.0  # lower limit
            n293 = Greater?(x=w530, y=w517) -> (0:w521:bool)
            n294 = Less?(x=w530, y=w516) -> (x < y?=w524:bool)
            n295 = Greater?(x=w529, y=w512) -> (0:w508:bool)
            n296 = Less?(x=w529, y=w513) -> (x < y?=w505:bool)
            n297 = In Range and Coerce(upper limit=w517, x=w530, lower limit=w516) -> (In Range?=w515:bool)  [unwired: 1 out]
            n298 = In Range and Coerce(upper limit=w512, x=w529, lower limit=w513) -> (In Range?=w514:bool)  [unwired: 1 out]
            n299 = call-poly <vilib>:"NT Read Value.vi"("default value"="Stop", "name"="Climb/Climb Diection") -> ("value"=w528:string)  [unwired: 7 in, 2 out]
            n300 = Equal?(x=w528, y="Up") -> (x = y?=w523:bool)
            n301 = Equal?(x=w528, y="Down") -> (x = y?=w520:bool)
            n302 = Equal?(x=w528, y="Up") -> (x = y?=w506:bool)
            n303 = Equal?(x=w528, y="Down") -> (x = y?=w509:bool)
            n304 = And(x=w523, y=w524) -> (x .and. y?=w525:bool)
            n305 = And(x=w520, y=w521) -> (x .and. y?=w526:bool)
            n306 = And(x=w506, y=w505) -> (x .and. y?=w504:bool)
            n307 = And(x=w509, y=w508) -> (x .and. y?=w503:bool)
            n308 = Compound Arithmetic op=OR(w515, w525, w526) -> (w527:bool)
            n309 = Compound Arithmetic op=OR(w514, w504, w503) -> (w502:bool)
            n310 = Select(t=w528, s=w527, f="Stop" ("t")) -> (s? t:f=w500:string)
            n311 = Select(t=w528, s=w502, f="Stop" ("t")) -> (s? t:f=w498:string)
            n312 = case shown="\"Up\"" w500 {
              frame "Stop", Default {
                n313 = call <vilib>:"WPI_MotorControlRefNum Registry Get.vi"("refnum name"="Climb L") -> ("error out"=w552:errorcluster, "MotorControlDevRef"=w551:T27)  [unwired: 9 in]
                n314 = call <vilib>:"SPARK Set Output Advanced.vi"("error in (no error)"=w552, "Control Mode"=Spark_MAX_Control_Type."Percent VBus", "Setpoint"=0.0 ("t"), "MotorControlDevRef"=w551) -> ()  [unwired: 6 in, 2 out]
              }
              frame "Up" {
                n315 = call <vilib>:"WPI_MotorControlRefNum Registry Get.vi"("refnum name"="Climb L") -> ("error out"=w557:errorcluster, "MotorControlDevRef"=w556:T27)  [unwired: 9 in]
                n316 = call <vilib>:"SPARK Set Output Advanced.vi"("error in (no error)"=w557, "Control Mode"=Spark_MAX_Control_Type."Percent VBus", "Setpoint"=0.9 ("t"), "MotorControlDevRef"=w556) -> ()  [unwired: 6 in, 2 out]
              }
              frame "Down" {
                n317 = call <vilib>:"WPI_MotorControlRefNum Registry Get.vi"("refnum name"="Climb L") -> ("error out"=w562:errorcluster, "MotorControlDevRef"=w561:T27)  [unwired: 9 in]
                n318 = call <vilib>:"SPARK Set Output Advanced.vi"("error in (no error)"=w562, "Control Mode"=Spark_MAX_Control_Type."Percent VBus", "Setpoint"=-0.9 ("t"), "MotorControlDevRef"=w561) -> ()  [unwired: 6 in, 2 out]
              }
            }
            n319 = case shown="\"Up\"" w498 {
              frame "Stop", Default {
                n320 = call <vilib>:"WPI_MotorControlRefNum Registry Get.vi"("refnum name"="Climb R") -> ("error out"=w533:errorcluster, "MotorControlDevRef"=w534:T27)  [unwired: 9 in]
                n321 = call <vilib>:"SPARK Set Output Advanced.vi"("error in (no error)"=w533, "Control Mode"=Spark_MAX_Control_Type."Percent VBus", "Setpoint"=0.0 ("t"), "MotorControlDevRef"=w534) -> ()  [unwired: 6 in, 2 out]
              }
              frame "Up" {
                n322 = call <vilib>:"WPI_MotorControlRefNum Registry Get.vi"("refnum name"="Climb R") -> ("error out"=w538:errorcluster, "MotorControlDevRef"=w539:T27)  [unwired: 9 in]
                n323 = call <vilib>:"SPARK Set Output Advanced.vi"("error in (no error)"=w538, "Control Mode"=Spark_MAX_Control_Type."Percent VBus", "Setpoint"=0.9 ("t"), "MotorControlDevRef"=w539) -> ()  [unwired: 6 in, 2 out]
              }
              frame "Down" {
                n324 = call <vilib>:"WPI_MotorControlRefNum Registry Get.vi"("refnum name"="Climb R") -> ("error out"=w543:errorcluster, "MotorControlDevRef"=w544:T27)  [unwired: 9 in]
                n325 = call <vilib>:"SPARK Set Output Advanced.vi"("error in (no error)"=w543, "Control Mode"=Spark_MAX_Control_Type."Percent VBus", "Setpoint"=-0.9 ("t"), "MotorControlDevRef"=w544) -> ()  [unwired: 6 in, 2 out]
              }
            }
            n326 = call-poly <vilib>:"NT Write Value.vi"("value"=w498, "name"="Climb/Climb R Status") -> ()  [unwired: 9 in, 1 out]
            n327 = call-poly <vilib>:"NT Write Value.vi"("value"=w500, "name"="Climb/Climb L Status") -> ()  [unwired: 9 in, 1 out]
          }
          frame "PID Extend" {
            w576 = 450.0  # upper limit
            w577 = 0.0  # lower limit
            w582 = 450.0  # upper limit
            w581 = 0.0  # lower limit
            n328 = Greater?(x=w580, y=w582) -> (0:w587:bool)
            n329 = Less?(x=w580, y=w581) -> (x < y?=w590:bool)
            n330 = Greater?(x=w564, y=w576) -> (0:w572:bool)
            n331 = Less?(x=w564, y=w577) -> (x < y?=w569:bool)
            n332 = In Range and Coerce(upper limit=w582, x=w580, lower limit=w581) -> (In Range?=w579:bool)  [unwired: 1 out]
            n333 = In Range and Coerce(upper limit=w576, x=w564, lower limit=w577) -> (In Range?=w578:bool)  [unwired: 1 out]
            n334 = call-poly <vilib>:"NT Read Value.vi"("default value"="Stop", "name"="Climb/Climb Diection") -> ("value"=w563:string)  [unwired: 7 in, 2 out]
            n335 = Equal?(x=w563, y="Up") -> (x = y?=w589:bool)
            n336 = Equal?(x=w563, y="Down") -> (x = y?=w586:bool)
            n337 = Equal?(x=w563, y="Up") -> (x = y?=w570:bool)
            n338 = Equal?(x=w563, y="Down") -> (x = y?=w573:bool)
            n339 = And(x=w589, y=w590) -> (x .and. y?=w591:bool)
            n340 = And(x=w586, y=w587) -> (x .and. y?=w592:bool)
            n341 = And(x=w570, y=w569) -> (x .and. y?=w568:bool)
            n342 = And(x=w573, y=w572) -> (x .and. y?=w567:bool)
            n343 = Compound Arithmetic op=OR(w579, w591, w592) -> (w593:bool)
            n344 = Compound Arithmetic op=OR(w578, w568, w567) -> (w566:bool)
            n345 = Select(t=w563, s=w593, f="Stop" ("t")) -> (s? t:f=w583:string)
            n346 = Select(t=w563, s=w566, f="Stop" ("t")) -> (s? t:f=w565:string)
            n347 = case shown="\"Stop\", Default" w583 {
              frame "Stop", Default {
                n348 = call <vilib>:"WPI_MotorControlRefNum Registry Get.vi"("refnum name"="Climb L") -> ("error out"=w615:errorcluster, "MotorControlDevRef"=w614:T27)  [unwired: 9 in]
                n349 = call <vilib>:"SPARK Set Output Advanced.vi"("error in (no error)"=w615, "Control Mode"=Spark_MAX_Control_Type."Percent VBus", "Setpoint"=0.0 ("t"), "MotorControlDevRef"=w614) -> ()  [unwired: 6 in, 2 out]
              }
              frame "Up" {
                n350 = call <vilib>:"WPI_MotorControlRefNum Registry Get.vi"("refnum name"="Climb L") -> ("error out"=w620:errorcluster, "MotorControlDevRef"=w619:T27)  [unwired: 9 in]
                n351 = call <vilib>:"SPARK Set Output Advanced.vi"("error in (no error)"=w620, "Control Mode"=Spark_MAX_Control_Type."Percent VBus", "Setpoint"=0.6 ("t"), "MotorControlDevRef"=w619) -> ()  [unwired: 6 in, 2 out]
              }
              frame "Down" {
                n352 = call <vilib>:"WPI_MotorControlRefNum Registry Get.vi"("refnum name"="Climb L") -> ("error out"=w625:errorcluster, "MotorControlDevRef"=w624:T27)  [unwired: 9 in]
                n353 = call <vilib>:"SPARK Set Output Advanced.vi"("error in (no error)"=w625, "Control Mode"=Spark_MAX_Control_Type."Percent VBus", "Setpoint"=-0.6 ("t"), "MotorControlDevRef"=w624) -> ()  [unwired: 6 in, 2 out]
              }
            }
            n354 = case shown="\"Stop\", Default" w565 {
              frame "Stop", Default {
                n355 = call <vilib>:"WPI_MotorControlRefNum Registry Get.vi"("refnum name"="Climb R") -> ("error out"=w596:errorcluster, "MotorControlDevRef"=w597:T27)  [unwired: 9 in]
                n356 = call <vilib>:"SPARK Set Output Advanced.vi"("error in (no error)"=w596, "Control Mode"=Spark_MAX_Control_Type."Percent VBus", "Setpoint"=0.0 ("t"), "MotorControlDevRef"=w597) -> ()  [unwired: 6 in, 2 out]
              }
              frame "Up" {
                n357 = call <vilib>:"WPI_MotorControlRefNum Registry Get.vi"("refnum name"="Climb R") -> ("error out"=w601:errorcluster, "MotorControlDevRef"=w602:T27)  [unwired: 9 in]
                n358 = call <vilib>:"SPARK Set Output Advanced.vi"("error in (no error)"=w601, "Control Mode"=Spark_MAX_Control_Type."Percent VBus", "Setpoint"=0.6 ("t"), "MotorControlDevRef"=w602) -> ()  [unwired: 6 in, 2 out]
              }
              frame "Down" {
                n359 = call <vilib>:"WPI_MotorControlRefNum Registry Get.vi"("refnum name"="Climb R") -> ("error out"=w606:errorcluster, "MotorControlDevRef"=w607:T27)  [unwired: 9 in]
                n360 = call <vilib>:"SPARK Set Output Advanced.vi"("error in (no error)"=w606, "Control Mode"=Spark_MAX_Control_Type."Percent VBus", "Setpoint"=-0.6 ("t"), "MotorControlDevRef"=w607) -> ()  [unwired: 6 in, 2 out]
              }
            }
          }
        }
      }
      n361 = while {
        shift-right: [w664] -> _
        shift-left: w473 -> [w664]
        stop <- FALSE stop-if-true
        w640 = 1.0  # Kn
        w642 = 0.0  # Ks
        w641 = 0.0  # Ka
        w632 = 650.0  # [Default] IntakeSpeed_RPM Dmd
        w659 = 1.0  # Kn
        w657 = 0.0  # Ks
        w658 = 0.0  # Ka
        # "Velocity FF"
        # "Trigger Status:\n- Stop [Default]\n- FromIntake\n- ToShooter\n- ShootReverse\n- Reverse"
        # "Intake Status:\n- Stop [Default]\n- Spin\n- Reverse"
        n362 = Wait (ms)(milliseconds to wait=u32 20) -> ()  [unwired: 1 out]
        n363 = call <vilib>:"DCMotor_PickMotorSelector.vi"("DCMOTOR_TYPES"=DCMOTOR_TYPES_ENUM."NEO" ("Motor Type"), "Num Motors"=1) -> ("DCMOTOR"=w631:T32)  [unwired: 9 in]
        n364 = call <vilib>:"DCMotor_PickMotorSelector.vi"("DCMOTOR_TYPES"=DCMOTOR_TYPES_ENUM."Falcon 500" ("Motor Type"), "Num Motors"=1) -> ("DCMOTOR"=w628:T32)  [unwired: 9 in]
        n365 = Unbundle By Name(w631) -> ("FreeSpeed_RadPerSec"=w645:dbl)
        n366 = Unbundle By Name(w628) -> ("FreeSpeed_RadPerSec"=w652:dbl)
        n367 = call-poly <vilib>:"NT Read Value.vi"("default value"="Stop", "name"="Intake/Trigger Status") -> ("value"=w635:string)  [unwired: 7 in, 2 out]
        n368 = call-poly <vilib>:"NT Read Value.vi"("default value"="Stop", "name"="Intake/Intake Status") -> ("value"=w662:string)  [unwired: 7 in, 2 out]
        n369 = call-poly <vilib>:"NT Read Value.vi"("name"="Intake/Gear Ratio") -> ("value"=w650:dbl)  [unwired: 8 in, 2 out]
        n370 = call-poly <vilib>:"NT Read Value.vi"("name"="Intake/Gear Ratio/Trigger") -> ("value"=w636:dbl)  [unwired: 8 in, 2 out]
        n371 = Reciprocal(x=w636) -> (1/x=w643:dbl)
        n372 = Reciprocal(x=w650) -> (1/x=w654:dbl)
        n373 = Compound Arithmetic op=MULTIPLY(w645, w643) -> (w646:dbl)
        n374 = Compound Arithmetic op=MULTIPLY(w652, w654) -> (w651:dbl)
        n375 = call <vilib>:"Units_RadiansPerSecondToRotationsPerMinute.vi"("RadiansPerSecond"=w646) -> ("RotationsPerMinute"=w639:dbl)  [unwired: 10 in]
        n376 = call <vilib>:"Units_RadiansPerSecondToRotationsPerMinute.vi"("RadiansPerSecond"=w651) -> ("RotationsPerMinute"=w660:dbl)  [unwired: 10 in]
        n377 = Reciprocal(x=w639) -> (1/x=w638:dbl)
        n378 = Reciprocal(x=w660) -> (1/x=w661:dbl)
        n379 = call <vilib>:"SimpleMotorFF_New.vi"("Kn"=w640, "Ka"=w641, "Kv"=w638, "Ks"=w642) -> ("SIMPLE_MOTOR_FF"=w637:T33)  [unwired: 7 in]
        n380 = call <vilib>:"SimpleMotorFF_New.vi"("Kn"=w659, "Ka"=w658, "Kv"=w661, "Ks"=w657) -> ("SIMPLE_MOTOR_FF"=w655:T33)  [unwired: 7 in]
        n381 = call "Is Value Changed.vim"("value"=w635) -> ("changed or first call?"=w634:bool)
        n382 = call <vilib>:"SimpleMotorFF_Calculate_CalcAccel.vi"("dT_Sec"=0.02, "VelSp"=w632, "SIMPLE_MOTOR_FF"=w655) -> ("FeedForward"=w633:dbl)  [unwired: 8 in]
        n383 = case shown="\"Spin\"" w662 {
          tunnel: w632 -> [_ w768 _]
          tunnel: w650 -> [_ w750 _]
          tunnel: w633 -> [_ w751 _]
          tunnel: w632 -> [_ _ _]
          frame "Stop", Default {
            w741 = T34 0 items=["PercentOutput"=0, "Position"=1, "Velocity"=2, "Current"=3, "Follower"=5, "MotionProfile"=6, "MotionMagic"=7, "MotionProfileArc"=10, "Disabled"=15] ("Control Mode")
            w746 = T34 0 items=["PercentOutput"=0, "Position"=1, "Velocity"=2, "Current"=3, "Follower"=5, "MotionProfile"=6, "MotionMagic"=7, "MotionProfileArc"=10, "Disabled"=15] ("Control Mode")
            n384 = call <vilib>:"CTRE_Phoenix_MotorControl_RefNumRegistryGet.vi"("refnum name"="Intake L") -> ("error out"=w748:errorcluster, "PhoenixMotorControlDevRef"=w747:T27)  [unwired: 9 in]
            n385 = call <vilib>:"CTRE_Phoenix_MotorControl_RefNumRegistryGet.vi"("refnum name"="Intake R") -> ("error out"=w743:errorcluster, "PhoenixMotorControlDevRef"=w742:T27)  [unwired: 9 in]
            n386 = call <vilib>:"CTRE_Phoenix_MotorControl_Set.vi"("error in (no error)"=w748, "Output"=0.0, "Control Mode"=w746, "PhoenixMotorControlDevRef"=w747) -> ()  [unwired: 6 in, 2 out]
            n387 = call <vilib>:"CTRE_Phoenix_MotorControl_Set.vi"("error in (no error)"=w743, "Output"=0.0, "Control Mode"=w741, "PhoenixMotorControlDevRef"=w742) -> ()  [unwired: 6 in, 2 out]
          }
          frame "Spin" {
            w754 = T34 2 items=["PercentOutput"=0, "Position"=1, "Velocity"=2, "Current"=3, "Follower"=5, "MotionProfile"=6, "MotionMagic"=7, "MotionProfileArc"=10, "Disabled"=15] ("Control Mode")
            w759 = 2048.0  # ticks per rev
            w765 = T34 2 items=["PercentOutput"=0, "Position"=1, "Velocity"=2, "Current"=3, "Follower"=5, "MotionProfile"=6, "MotionMagic"=7, "MotionProfileArc"=10, "Disabled"=15] ("Control Mode")
            # "1 (sec) / 10 (100 ms)"
            n388 = Compound Arithmetic op=MULTIPLY(w768, w750) -> (w758:dbl)
            n389 = call <vilib>:"Units_RotationsPerMinuteToRadiansPerSecond.vi"("RotationsPerMinute"=w758) -> ("RadiansPerSecond"=w760:dbl)  [unwired: 10 in]
            n390 = call <vilib>:"Units_RadiansToRotations.vi"("Radians"=w760) -> ("Rotations"=w757:dbl)  [unwired: 10 in]
            n391 = Divide(x=w757, y=10.0) -> (x/y=w761:dbl)
            n392 = Compound Arithmetic op=MULTIPLY(w761, w759) -> (w749:dbl)
            n393 = call <vilib>:"CTRE_Phoenix_MotorControl_RefNumRegistryGet.vi"("refnum name"="Intake L") -> ("error out"=w767:errorcluster, "PhoenixMotorControlDevRef"=w766:T27)  [unwired: 9 in]
            n394 = call <vilib>:"CTRE_Phoenix_MotorControl_RefNumRegistryGet.vi"("refnum name"="Intake R") -> ("error out"=w756:errorcluster, "PhoenixMotorControlDevRef"=w755:T27)  [unwired: 9 in]
            n395 = call <vilib>:"CTRE_Phoenix_MotorControl_Set.vi"("Demand1"=w751, "DemandType"=T23."DemandType_ArbitraryFeedForward", "error in (no error)"=w767, "Output"=w749, "Control Mode"=w765, "PhoenixMotorControlDevRef"=w766) -> ()  [unwired: 4 in, 2 out]
            n396 = call <vilib>:"CTRE_Phoenix_MotorControl_Set.vi"("Demand1"=w751, "DemandType"=T23."DemandType_ArbitraryFeedForward", "error in (no error)"=w756, "Output"=w749, "Control Mode"=w754, "PhoenixMotorControlDevRef"=w755) -> ()  [unwired: 4 in, 2 out]
          }
          frame "Reverse" {
            w771 = T34 0 items=["PercentOutput"=0, "Position"=1, "Velocity"=2, "Current"=3, "Follower"=5, "MotionProfile"=6, "MotionMagic"=7, "MotionProfileArc"=10, "Disabled"=15] ("Control Mode")
            w776 = T34 0 items=["PercentOutput"=0, "Position"=1, "Velocity"=2, "Current"=3, "Follower"=5, "MotionProfile"=6, "MotionMagic"=7, "MotionProfileArc"=10, "Disabled"=15] ("Control Mode")
            n397 = call <vilib>:"CTRE_Phoenix_MotorControl_RefNumRegistryGet.vi"("refnum name"="Intake L") -> ("error out"=w778:errorcluster, "PhoenixMotorControlDevRef"=w777:T27)  [unwired: 9 in]
            n398 = call <vilib>:"CTRE_Phoenix_MotorControl_RefNumRegistryGet.vi"("refnum name"="Intake R") -> ("error out"=w773:errorcluster, "PhoenixMotorControlDevRef"=w772:T27)  [unwired: 9 in]
            n399 = call <vilib>:"CTRE_Phoenix_MotorControl_Set.vi"("error in (no error)"=w778, "Output"=-1.0, "Control Mode"=w776, "PhoenixMotorControlDevRef"=w777) -> ()  [unwired: 6 in, 2 out]
            n400 = call <vilib>:"CTRE_Phoenix_MotorControl_Set.vi"("error in (no error)"=w773, "Output"=-1.0, "Control Mode"=w771, "PhoenixMotorControlDevRef"=w772) -> ()  [unwired: 6 in, 2 out]
          }
        }
        n401 = case shown="\"Slow Reverse\"" w635 {
          tunnel: w637 -> [_ w673 w692 _ _ _]
          tunnel: w636 -> [_ w672 w691 _ _ _]
          tunnel: w634 -> [_ _ _ w719 _ _]
          frame "Stop", Default {
            n402 = call <vilib>:"WPI_MotorControlRefNum Registry Get.vi"("refnum name"="Trigger") -> ("error out"=w671:errorcluster, "MotorControlDevRef"=w670:T27)  [unwired: 9 in]
            n403 = call <vilib>:"SPARK Set Output Advanced.vi"("error in (no error)"=w671, "Control Mode"=Spark_MAX_Control_Type."Percent VBus", "Setpoint"=0.0 ("t"), "MotorControlDevRef"=w670) -> ()  [unwired: 6 in, 2 out]
          }
          frame "FromIntake" {
            n404 = disable-structure shown="Enabled" {
              disable-tunnel: w673 -> [w680 _]
              disable-tunnel: w672 -> [w676 _]
              frame Disabled {
                w679 = 12.0  # Nominal Voltage
                w674 = 80.0  # TriggerSpeed_RPM Dmd
                n405 = call <vilib>:"SimpleMotorFF_Calculate_CalcAccel.vi"("dT_Sec"=0.02, "VelSp"=w674, "SIMPLE_MOTOR_FF"=w680) -> ("FeedForward"=w678:dbl)  [unwired: 8 in]
                n406 = Compound Arithmetic op=MULTIPLY(w674, w676) -> (w675:dbl)
                n407 = call <vilib>:"WPI_MotorControlRefNum Registry Get.vi"("refnum name"="Trigger") -> ("error out"=w685:errorcluster, "MotorControlDevRef"=w684:T27)  [unwired: 9 in]
                n408 = Multiply(x=w678, y=w679) -> (x*y=w677:dbl)
                n409 = call <vilib>:"SPARK Set Output Advanced.vi"("Arbitrary Feed Forward (0)"=w677, "error in (no error)"=w685, "Control Mode"=Spark_MAX_Control_Type."Velocity", "Setpoint"=w675, "MotorControlDevRef"=w684) -> ()  [unwired: 5 in, 2 out]
              }
              frame Enabled {
                n410 = call <vilib>:"WPI_MotorControlRefNum Registry Get.vi"("refnum name"="Trigger") -> ("error out"=w690:errorcluster, "MotorControlDevRef"=w689:T27)  [unwired: 9 in]
                n411 = call <vilib>:"SPARK Set Output Advanced.vi"("error in (no error)"=w690, "Control Mode"=Spark_MAX_Control_Type."Percent VBus", "Setpoint"=0.4, "MotorControlDevRef"=w689) -> ()  [unwired: 6 in, 2 out]
              }
            }
          }
          frame "ToShooter" {
            n412 = disable-structure shown="Enabled" {
              disable-tunnel: w692 -> [w699 _]
              disable-tunnel: w691 -> [w695 _]
              frame Disabled {
                w698 = 12.0  # Nominal Voltage
                w693 = 400.0  # TriggerSpeed_RPM Dmd
                n413 = call <vilib>:"SimpleMotorFF_Calculate_CalcAccel.vi"("dT_Sec"=0.02, "VelSp"=w693, "SIMPLE_MOTOR_FF"=w699) -> ("FeedForward"=w697:dbl)  [unwired: 8 in]
                n414 = Compound Arithmetic op=MULTIPLY(w693, w695) -> (w694:dbl)
                n415 = call <vilib>:"WPI_MotorControlRefNum Registry Get.vi"("refnum name"="Trigger") -> ("error out"=w704:errorcluster, "MotorControlDevRef"=w703:T27)  [unwired: 9 in]
                n416 = Multiply(x=w697, y=w698) -> (x*y=w696:dbl)
                n417 = call <vilib>:"SPARK Set Output Advanced.vi"("Arbitrary Feed Forward (0)"=w696, "error in (no error)"=w704, "Control Mode"=Spark_MAX_Control_Type."Velocity", "Setpoint"=w694, "MotorControlDevRef"=w703) -> ()  [unwired: 5 in, 2 out]
              }
              frame Enabled {
                n418 = call <vilib>:"WPI_MotorControlRefNum Registry Get.vi"("refnum name"="Trigger") -> ("error out"=w709:errorcluster, "MotorControlDevRef"=w708:T27)  [unwired: 9 in]
                n419 = call <vilib>:"SPARK Set Output Advanced.vi"("error in (no error)"=w709, "Control Mode"=Spark_MAX_Control_Type."Percent VBus", "Setpoint"=0.7 ("t"), "MotorControlDevRef"=w708) -> ()  [unwired: 6 in, 2 out]
              }
            }
          }
          frame "ShootReverse" {
            # "Backup plan, if limit switch stopper malfunction"
            # "End this when trigger turns approx 120 deg"
            n420 = feedback #5(0.0 ("Sensor Position")) -> (w718:dbl)
            n421 = call-poly <vilib>:"NT Read Value.vi"("name"="Intake/TriggerPos_Rotation Act") -> ("value"=w710:dbl)  [unwired: 8 in, 2 out]
            n422 = case shown="False" w719 {
              tunnel: [w727 w728] -> w716
              tunnel: w718 -> [w727 _]
              tunnel: w710 -> [_ w728]
              frame False {
              }
              frame True {
              }
            }
            n423 = feedback-in #5(w716) -> ()
            n424 = Subtract(x=w716, y=w710) -> (x-y=w715:dbl)
            n425 = Absolute Value(x=w715) -> (abs(x)=w714:dbl)
            n426 = Greater?(x=w714, y=0.3) -> (0:w712:bool)
            n427 = call <vilib>:"WPI_MotorControlRefNum Registry Get.vi"("refnum name"="Trigger") -> ("error out"=w724:errorcluster, "MotorControlDevRef"=w723:T27)  [unwired: 9 in]
            n428 = case shown="True" w712 {
              frame False {
              }
              frame True {
                n429 = call-poly <vilib>:"NT Write Value.vi"("value"="Stop", "name"="Intake/Trigger Status") -> ()  [unwired: 9 in, 1 out]
              }
            }
            n430 = call <vilib>:"SPARK Set Output Advanced.vi"("error in (no error)"=w724, "Control Mode"=Spark_MAX_Control_Type."Percent VBus", "Setpoint"=-0.4 ("t"), "MotorControlDevRef"=w723) -> ()  [unwired: 6 in, 2 out]
          }
          frame "Reverse" {
            n431 = call <vilib>:"WPI_MotorControlRefNum Registry Get.vi"("refnum name"="Trigger") -> ("error out"=w733:errorcluster, "MotorControlDevRef"=w732:T27)  [unwired: 9 in]
            n432 = call <vilib>:"SPARK Set Output Advanced.vi"("error in (no error)"=w733, "Control Mode"=Spark_MAX_Control_Type."Percent VBus", "Setpoint"=-1.0 ("t"), "MotorControlDevRef"=w732) -> ()  [unwired: 6 in, 2 out]
          }
          frame "Slow Reverse" {
            n433 = call <vilib>:"WPI_MotorControlRefNum Registry Get.vi"("refnum name"="Trigger") -> ("error out"=w738:errorcluster, "MotorControlDevRef"=w737:T27)  [unwired: 9 in]
            n434 = call <vilib>:"SPARK Set Output Advanced.vi"("error in (no error)"=w738, "Control Mode"=Spark_MAX_Control_Type."Percent VBus", "Setpoint"=-0.4 ("t"), "MotorControlDevRef"=w737) -> ()  [unwired: 6 in, 2 out]
          }
        }
      }
      n435 = while {
        shift-right: [w1076] -> _
        shift-left: w473 -> [w1076]
        stop <- FALSE stop-if-true
        w1028 = 0.497  # Arm Length
        w1046 = 9.81  # gravity
        w1042 = 10.5  # Shooter Mass_KG
        w1071 = 1.0  # Kn
        w1069 = 0.0  # Ks
        w1070 = 0.0  # Ka
        # "Shooter Angle Status:\n- Stop [Default]\n- ToDesiredAngle"
        # "Shooter Status:\n- Stop [Default]\n- Spin\n- AMP"
        n436 = Wait (ms)(milliseconds to wait=u32 20) -> ()  [unwired: 1 out]
        n437 = call <vilib>:"DCMotor_PickMotorSelector.vi"("DCMOTOR_TYPES"=DCMOTOR_TYPES_ENUM."Falcon 500" ("Motor Type"), "Num Motors"=1) -> ("DCMOTOR"=w1020:T32)  [unwired: 9 in]
        n438 = Unbundle By Name(w1020) -> ("FreeSpeed_RadPerSec"=w1062:dbl)
        n439 = call-poly <vilib>:"NT Read Value.vi"("default value"="Stop", "name"="Shooter/Shooter Angle Status") -> ("value"=w1058:string)  [unwired: 7 in, 2 out]
        n440 = call-poly <vilib>:"NT Read Value.vi"("default value"="Stop", "name"="Shooter/Shooter Status") -> ("value"=w1074:string)  [unwired: 7 in, 2 out]
        n441 = call-poly <vilib>:"NT Read Value.vi"("name"="Shooter/Gear Ratio/Shooter") -> ("value"=w1060:dbl)  [unwired: 8 in, 2 out]
        n442 = Reciprocal(x=w1060) -> (1/x=w1064:dbl)
        n443 = call <vilib>:"DCMotor_PickMotorSelector.vi"("DCMOTOR_TYPES"=DCMOTOR_TYPES_ENUM."Falcon 500" ("Motor Type"), "Num Motors"=1) -> ("DCMOTOR"=w1022:T32)  [unwired: 9 in]
        n444 = call-poly <vilib>:"NT Read Value.vi"("name"="Shooter/Shooter Angle PID") -> ("value"=w1049:dbl[])  [unwired: 8 in, 2 out]
        n445 = Compound Arithmetic op=MULTIPLY(w1062, w1064) -> (w1061:dbl)
        n446 = Unbundle By Name(w1022) -> ("StallTorque_NM"=w1045:dbl)
        n447 = call <vilib>:"Units_RadiansPerSecondToRotationsPerMinute.vi"("RadiansPerSecond"=w1061) -> ("RotationsPerMinute"=w1072:dbl)  [unwired: 10 in]
        n448 = Reciprocal(x=w1072) -> (1/x=w1073:dbl)
        n449 = call-poly <vilib>:"NT Read Value.vi"("name"="Shooter/Gear Ratio/Shooter Angle") -> ("value"=w1044:dbl)  [unwired: 8 in, 2 out]
        n450 = call-poly <vilib>:"NT Read Value.vi"("name"="Shooter/Angle_Deg Dmd") -> ("value"=w1036:dbl)  [unwired: 8 in, 2 out]
        n451 = call-poly <vilib>:"NT Read Value.vi"("name"="Shooter/Angle_Deg Act") -> ("value"=w1048:dbl)  [unwired: 8 in, 2 out]
        n452 = Index Array(array=w1049) -> (element #1=w1029:dbl, element #2=w1033:dbl, element #3=w1030:dbl)  [unwired: 3 in]
        n453 = call-poly <vilib>:"NT Read Value.vi"("default value"=5000.0, "name"="Shooter/Speed_RPM AMP Dmd") -> ("value"=w1025:dbl)  [unwired: 7 in, 2 out]
        n454 = call-poly <vilib>:"NT Read Value.vi"("default value"=5000.0, "name"="Shooter/Speed_RPM Dmd") -> ("value"=w1066:dbl)  [unwired: 7 in, 2 out]
        n455 = Reciprocal(x=w1044) -> (1/x=w1043:dbl)
        n456 = Reciprocal(x=w1045) -> (1/x=w1039:dbl)
        n457 = Bundle(cluster=T26 {"proportional gain (Kp)"=2.25, "integral time (Ki)"=0.0, "derivative time (Kd)"=0.0} ("PID gains"), "proportional gain (Kp)"=w1029, "integral time (Ki)"=w1033, "derivative time (Kd)"=w1030) -> (w1050:T26)
        n458 = Subtract(x=w1036, y=17.0) -> (x-y=w1034:dbl)
        n459 = Compound Arithmetic op=MULTIPLY(w1042, w1046, w1028, w1043) -> (w1038:dbl)
        n460 = call <vilib>:"SimpleMotorFF_New.vi"("Kn"=w1071, "Ka"=w1070, "Kv"=w1073, "Ks"=w1069) -> ("SIMPLE_MOTOR_FF"=w1026:T33)  [unwired: 7 in]
        n461 = call <vilib>:"Units_DegreesToRadians.vi"("Degrees"=w1034) -> ("Radians"=w1041:dbl)  [unwired: 10 in]
        n462 = Cosine(x=w1041) -> (cos(x)=w1040:dbl)
        n463 = call <vilib>:"SimpleMotorFF_Calculate_CalcAccel.vi"("dT_Sec"=0.02, "VelSp"=w1025, "SIMPLE_MOTOR_FF"=w1026) -> ("FeedForward"=w1024:dbl)  [unwired: 8 in]
        n464 = call <vilib>:"SimpleMotorFF_Calculate_CalcAccel.vi"("dT_Sec"=0.02, "VelSp"=w1066, "SIMPLE_MOTOR_FF"=w1026) -> ("FeedForward"=w1065:dbl)  [unwired: 8 in]
        n465 = case shown="\"Spin\"" w1074 {
          tunnel: w1066 -> [_ w1139 _]
          tunnel: w1065 -> [_ w1111 _]
          tunnel: w1060 -> [_ w1137 w1158]
          tunnel: w1025 -> [_ w1138 w1159]
          tunnel: w1024 -> [_ w1112 w1141]
          frame "Stop", Default {
            w1103 = T34 0 items=["PercentOutput"=0, "Position"=1, "Velocity"=2, "Current"=3, "Follower"=5, "MotionProfile"=6, "MotionMagic"=7, "MotionProfileArc"=10, "Disabled"=15] ("Control Mode")
            w1108 = T34 0 items=["PercentOutput"=0, "Position"=1, "Velocity"=2, "Current"=3, "Follower"=5, "MotionProfile"=6, "MotionMagic"=7, "MotionProfileArc"=10, "Disabled"=15] ("Control Mode")
            n466 = call <vilib>:"CTRE_Phoenix_MotorControl_RefNumRegistryGet.vi"("refnum name"="Shooter") -> ("error out"=w1105:errorcluster, "PhoenixMotorControlDevRef"=w1104:T27)  [unwired: 9 in]
            n467 = call <vilib>:"CTRE_Phoenix_MotorControl_RefNumRegistryGet.vi"("refnum name"="Shooter AMP") -> ("error out"=w1110:errorcluster, "PhoenixMotorControlDevRef"=w1109:T27)  [unwired: 9 in]
            n468 = call <vilib>:"CTRE_Phoenix_MotorControl_Set.vi"("error in (no error)"=w1105, "Output"=0.0, "Control Mode"=w1103, "PhoenixMotorControlDevRef"=w1104) -> ()  [unwired: 6 in, 2 out]
            n469 = call <vilib>:"CTRE_Phoenix_MotorControl_Set.vi"("error in (no error)"=w1110, "Output"=0.0, "Control Mode"=w1108, "PhoenixMotorControlDevRef"=w1109) -> ()  [unwired: 6 in, 2 out]
          }
          frame "Spin" {
            w1121 = 2048.0  # ticks per rev
            w1115 = T34 2 items=["PercentOutput"=0, "Position"=1, "Velocity"=2, "Current"=3, "Follower"=5, "MotionProfile"=6, "MotionMagic"=7, "MotionProfileArc"=10, "Disabled"=15] ("Control Mode")
            w1128 = 2048.0  # ticks per rev
            w1134 = T34 2 items=["PercentOutput"=0, "Position"=1, "Velocity"=2, "Current"=3, "Follower"=5, "MotionProfile"=6, "MotionMagic"=7, "MotionProfileArc"=10, "Disabled"=15] ("Control Mode")
            # "1 (sec) / 10 (100 ms)"
            # "Velocity FF"
            # "1 (sec) / 10 (100 ms)"
            n470 = Compound Arithmetic op=MULTIPLY(w1138, w1137) -> (w1122:dbl)
            n471 = Compound Arithmetic op=MULTIPLY(w1139, w1137) -> (w1127:dbl)
            n472 = call <vilib>:"Units_RotationsPerMinuteToRadiansPerSecond.vi"("RotationsPerMinute"=w1122) -> ("RadiansPerSecond"=w1120:dbl)  [unwired: 10 in]
            n473 = call <vilib>:"Units_RotationsPerMinuteToRadiansPerSecond.vi"("RotationsPerMinute"=w1127) -> ("RadiansPerSecond"=w1129:dbl)  [unwired: 10 in]
            n474 = call <vilib>:"Units_RadiansToRotations.vi"("Radians"=w1120) -> ("Rotations"=w1123:dbl)  [unwired: 10 in]
            n475 = call <vilib>:"Units_RadiansToRotations.vi"("Radians"=w1129) -> ("Rotations"=w1126:dbl)  [unwired: 10 in]
            n476 = Divide(x=w1123, y=10.0) -> (x/y=w1119:dbl)
            n477 = Divide(x=w1126, y=10.0) -> (x/y=w1130:dbl)
            n478 = Compound Arithmetic op=MULTIPLY(w1119, w1121) -> (w1124:dbl)
            n479 = Compound Arithmetic op=MULTIPLY(w1130, w1128) -> (w1125:dbl)
            n480 = call <vilib>:"CTRE_Phoenix_MotorControl_RefNumRegistryGet.vi"("refnum name"="Shooter AMP") -> ("error out"=w1113:errorcluster, "PhoenixMotorControlDevRef"=w1114:T27)  [unwired: 9 in]
            n481 = call <vilib>:"CTRE_Phoenix_MotorControl_RefNumRegistryGet.vi"("refnum name"="Shooter") -> ("error out"=w1136:errorcluster, "PhoenixMotorControlDevRef"=w1135:T27)  [unwired: 9 in]
            n482 = call <vilib>:"CTRE_Phoenix_MotorControl_Set.vi"("Demand1"=w1112, "DemandType"=T23."DemandType_ArbitraryFeedForward", "error in (no error)"=w1113, "Output"=w1124, "Control Mode"=w1115, "PhoenixMotorControlDevRef"=w1114) -> ()  [unwired: 4 in, 2 out]
            n483 = call <vilib>:"CTRE_Phoenix_MotorControl_Set.vi"("Demand1"=w1111, "DemandType"=T23."DemandType_ArbitraryFeedForward", "error in (no error)"=w1136, "Output"=w1125, "Control Mode"=w1134, "PhoenixMotorControlDevRef"=w1135) -> ()  [unwired: 4 in, 2 out]
          }
          frame "AMP" {
            w1150 = 2048.0  # ticks per rev
            w1144 = T34 2 items=["PercentOutput"=0, "Position"=1, "Velocity"=2, "Current"=3, "Follower"=5, "MotionProfile"=6, "MotionMagic"=7, "MotionProfileArc"=10, "Disabled"=15] ("Control Mode")
            w1155 = T34 0 items=["PercentOutput"=0, "Position"=1, "Velocity"=2, "Current"=3, "Follower"=5, "MotionProfile"=6, "MotionMagic"=7, "MotionProfileArc"=10, "Disabled"=15] ("Control Mode")
            # "1 (sec) / 10 (100 ms)"
            n484 = Compound Arithmetic op=MULTIPLY(w1159, w1158) -> (w1151:dbl)
            n485 = call <vilib>:"Units_RotationsPerMinuteToRadiansPerSecond.vi"("RotationsPerMinute"=w1151) -> ("RadiansPerSecond"=w1149:dbl)  [unwired: 10 in]
            n486 = call <vilib>:"Units_RadiansToRotations.vi"("Radians"=w1149) -> ("Rotations"=w1152:dbl)  [unwired: 10 in]
            n487 = Divide(x=w1152, y=10.0) -> (x/y=w1148:dbl)
            n488 = Compound Arithmetic op=MULTIPLY(w1148, w1150) -> (w1153:dbl)
            n489 = call <vilib>:"CTRE_Phoenix_MotorControl_RefNumRegistryGet.vi"("refnum name"="Shooter AMP") -> ("error out"=w1142:errorcluster, "PhoenixMotorControlDevRef"=w1143:T27)  [unwired: 9 in]
            n490 = call <vilib>:"CTRE_Phoenix_MotorControl_RefNumRegistryGet.vi"("refnum name"="Shooter") -> ("error out"=w1157:errorcluster, "PhoenixMotorControlDevRef"=w1156:T27)  [unwired: 9 in]
            n491 = call <vilib>:"CTRE_Phoenix_MotorControl_Set.vi"("Demand1"=w1141, "DemandType"=T23."DemandType_ArbitraryFeedForward", "error in (no error)"=w1142, "Output"=w1153, "Control Mode"=w1144, "PhoenixMotorControlDevRef"=w1143) -> ()  [unwired: 4 in, 2 out]
            n492 = call <vilib>:"CTRE_Phoenix_MotorControl_Set.vi"("error in (no error)"=w1157, "Output"=0.0, "Control Mode"=w1155, "PhoenixMotorControlDevRef"=w1156) -> ()  [unwired: 6 in, 2 out]
          }
        }
        n493 = Compound Arithmetic op=MULTIPLY(w1040, w1038, w1039) -> (w1037:dbl)
        n494 = case shown="\"ToDesiredAngle\"" w1058 {
          tunnel: w1036 -> [_ w1100]
          tunnel: w1048 -> [_ w1090]
          tunnel: w1050 -> [_ w1099]
          tunnel: w1037 -> [_ w1098]
          frame "Stop", Default {
            w1081 = T34 0 items=["PercentOutput"=0, "Position"=1, "Velocity"=2, "Current"=3, "Follower"=5, "MotionProfile"=6, "MotionMagic"=7, "MotionProfileArc"=10, "Disabled"=15] ("Control Mode")
            n495 = call <vilib>:"CTRE_Phoenix_MotorControl_RefNumRegistryGet.vi"("refnum name"="Shooter Angle") -> ("error out"=w1083:errorcluster, "PhoenixMotorControlDevRef"=w1082:T27)  [unwired: 9 in]
            n496 = call <vilib>:"CTRE_Phoenix_MotorControl_Set.vi"("error in (no error)"=w1083, "Output"=0.0, "Control Mode"=w1081, "PhoenixMotorControlDevRef"=w1082) -> ()  [unwired: 6 in, 2 out]
          }
          frame "ToDesiredAngle" {
            w1092 = 10.0  # lower limit
            w1093 = 105.0  # upper limit
            w1095 = T34 0 items=["PercentOutput"=0, "Position"=1, "Velocity"=2, "Current"=3, "Follower"=5, "MotionProfile"=6, "MotionMagic"=7, "MotionProfileArc"=10, "Disabled"=15] ("Control Mode")
            # "Emergency only"
            # "Using Shooter coder for PID"
            n497 = In Range and Coerce(upper limit=w1093, x=w1100, lower limit=w1092) -> (coerced(x)=w1091:dbl)  [unwired: 1 out]
            n498 = call <vilib>:"Parallel PID (DBL).vi"("FeedFwd Value"=w1098, "output range"=cluster{"high":dbl, "low":dbl} {"high"=1.0, "low"=-1.0}, "PID gains"=w1099, "process variable"=w1090, "setpoint"=w1091) -> ("output"=w1087:dbl)  [unwired: 3 in, 3 out]
            n499 = Less Or Equal?(x=w1090, y=115.0) -> (x <= y?=w1088:bool)
            n500 = Select(t=w1087, s=w1088, f=-0.085) -> (s? t:f=w1085:dbl)
            n501 = call <vilib>:"CTRE_Phoenix_MotorControl_RefNumRegistryGet.vi"("refnum name"="Shooter Angle") -> ("error out"=w1097:errorcluster, "PhoenixMotorControlDevRef"=w1096:T27)  [unwired: 9 in]
            n502 = call <vilib>:"CTRE_Phoenix_MotorControl_Set.vi"("error in (no error)"=w1097, "Output"=w1085, "Control Mode"=w1095, "PhoenixMotorControlDevRef"=w1096) -> ()  [unwired: 6 in, 2 out]
          }
        }
      }
      n503 = while {
        shift-right: [w1002] -> _
        shift-left: w473 -> [w1002]
        stop <- FALSE stop-if-true
        w845 = 2048.0  # ticks per rev
        w907 = 2048.0  # ticks per rev
        w921 = 30.0  # Spool Diameter_mm
        w925 = 30.0  # Spool Diameter_mm
        w972 = 2048.0  # ticks per rev
        w987 = 2048.0  # ticks per rev
        w979 = 2048.0  # ticks per rev
        # "Tag IDs for calcultating orientation setpoint: 3,4,7,8"
        # "[Default] Blue Alliance\nCuz the field origin is at blue alliance"
        # "Should be 32.55"
        # "Should be 32.55"
        # "Coast while in Shoot Mode and Intake Mode"
        # "Stop trigger after limit swtich pressed"
        # "10 (100 ms)/ 1 (sec)"
        # "10 (100 ms)/ 1 (sec)"
        # "Boot -180 to 180 deg, Change Direction: Off"
        # "To +/-\nPI"
        # "10 (100 ms)/ 1 (sec)"
        # "10 (100 ms)/ 1 (sec)"
        n504 = Wait (ms)(milliseconds to wait=u32 20) -> ()  [unwired: 1 out]
        n505 = call <vilib>:"CTRE_Phoenix_MotorControl_RefNumRegistryGet.vi"("refnum name"="Shooter AMP") -> ("error out"=w975:errorcluster, "PhoenixMotorControlDevRef"=w976:T27)  [unwired: 9 in]
        n506 = call <vilib>:"CTRE_Phoenix_MotorControl_RefNumRegistryGet.vi"("refnum name"="Shooter") -> ("error out"=w910:errorcluster, "PhoenixMotorControlDevRef"=w909:T27)  [unwired: 9 in]
        n507 = call <vilib>:"CTRE_Phoenix_MotorControl_RefNumRegistryGet.vi"("refnum name"="Shooter Angle") -> ("error out"=w985:errorcluster, "PhoenixMotorControlDevRef"=w984:T27)  [unwired: 9 in]
        n508 = call <vilib>:"CTRE_Phoenix_CANcoder_RefNumRegistryGet.vi"("refnum name"="Shooter coder") -> ("error out"=w962:errorcluster, "CTRE_CANcoder_DeviceRef"=w961:T35)  [unwired: 9 in]
        n509 = call-poly <vilib>:"CTRE_Phoenix_MotorController_Get_TalonFX.vi"("PhoenixMotorControlDevRef"=w976, "error in"=w975) -> ("Temperature (C)"=w980:dbl)  [unwired: 11 in, 2 out]
        n510 = call-poly <vilib>:"CTRE_Phoenix_MotorController_Get_TalonFX.vi"("PhoenixMotorControlDevRef"=w976, "error in"=w975) -> ("Velocity (Raw Sensor Units per 100 ms)"=w998:i32)  [unwired: 10 in, 3 out]
        n511 = call-poly <vilib>:"CTRE_Phoenix_MotorController_Get_TalonFX.vi"("PhoenixMotorControlDevRef"=w909, "error in"=w910) -> ("Temperature (C)"=w906:dbl)  [unwired: 11 in, 2 out]
        n512 = call-poly <vilib>:"CTRE_Phoenix_MotorController_Get_TalonFX.vi"("PhoenixMotorControlDevRef"=w909, "error in"=w910) -> ("Velocity (Raw Sensor Units per 100 ms)"=w898:i32)  [unwired: 10 in, 3 out]
        n513 = call-poly <vilib>:"CTRE_Phoenix_MotorController_Get_TalonFX.vi"("PhoenixMotorControlDevRef"=w984, "error in"=w985) -> ("Position (Raw Sensor Units)"=w990:i32)  [unwired: 10 in, 3 out]
        n514 = call-poly <vilib>:"CTRE_Phoenix_CANcoder_GetPolymorphic.vi"("CTRE_CANcoder_DeviceRef"=w961, "error in"=w962) -> ("Absolute Position"=w866:dbl)  [unwired: 9 in, 4 out]
        n515 = To Double Precision Float(number=w998) -> (double precision float=w997:dbl)
        n516 = To Double Precision Float(number=w898) -> (double precision float=w899:dbl)
        n517 = To Double Precision Float(number=w990) -> (double precision float=w983:dbl)
        n518 = call <vilib>:"Conv_Deg_Radians.vi"("Degress"=w866) -> ("Radians"=w943:dbl)  [unwired: 10 in]
        n519 = Multiply(x=w997, y=10.0) -> (x*y=w995:dbl)
        n520 = Multiply(x=w899, y=10.0) -> (x*y=w901:dbl)
        n521 = call-poly <vilib>:"NT Read Value.vi"("name"="Shooter/Gear Ratio/Shooter") -> ("value"=w950:dbl)  [unwired: 8 in, 2 out]
        n522 = call-poly <vilib>:"NT Read Value.vi"("name"="Shooter/Gear Ratio/Shooter") -> ("value"=w912:dbl)  [unwired: 8 in, 2 out]
        n523 = call-poly <vilib>:"NT Read Value.vi"("name"="Shooter/Gear Ratio/Shooter Angle") -> ("value"=w952:dbl)  [unwired: 8 in, 2 out]
        n524 = call-poly <vilib>:"NT Read Value.vi"("name"="Shooter/Gear Ratio/Shooter coder") -> ("value"=w954:dbl)  [unwired: 8 in, 2 out]
        n525 = Reciprocal(x=w979) -> (1/x=w1000:dbl)
        n526 = Reciprocal(x=w950) -> (1/x=w978:dbl)
        n527 = Reciprocal(x=w907) -> (1/x=w896:dbl)
        n528 = Reciprocal(x=w912) -> (1/x=w908:dbl)
        n529 = Reciprocal(x=w987) -> (1/x=w988:dbl)
        n530 = Reciprocal(x=w952) -> (1/x=w977:dbl)
        n531 = Reciprocal(x=w954) -> (1/x=w959:dbl)
        n532 = Compound Arithmetic op=MULTIPLY(w995, w1000, w978) -> (w994:dbl)
        n533 = Compound Arithmetic op=MULTIPLY(w901, w896, w908) -> (w902:dbl)
        n534 = Compound Arithmetic op=MULTIPLY(w983, w988, w977) -> (w991:dbl)
        n535 = Compound Arithmetic op=MULTIPLY(w943, w959) -> (w958:dbl)
        n536 = call <vilib>:"Conv_Rotations_Radians.vi"("Rotations"=w994) -> ("Radians"=w993:dbl)  [unwired: 10 in]
        n537 = call <vilib>:"Conv_Rotations_Radians.vi"("Rotations"=w902) -> ("Radians"=w903:dbl)  [unwired: 10 in]
        n538 = call <vilib>:"Conv_Rotations_Radians.vi"("Rotations"=w991) -> ("Radians"=w982:dbl)  [unwired: 10 in]
        n539 = call <vilib>:"MathUtil_AngleModulus.vi"("InputAngle"=w958) -> ("ModulsAngle"=w957:dbl)  [unwired: 10 in]
        n540 = call <vilib>:"Units_RadiansPerSecondToRotationsPerMinute.vi"("RadiansPerSecond"=w993) -> ("RotationsPerMinute"=w992:dbl)  [unwired: 10 in]
        n541 = call <vilib>:"Units_RadiansPerSecondToRotationsPerMinute.vi"("RadiansPerSecond"=w903) -> ("RotationsPerMinute"=w904:dbl)  [unwired: 10 in]
        n542 = call <vilib>:"Units_RadiansToDegrees.vi"("Radians"=w982) -> ("Degrees"=w916:dbl)  [unwired: 10 in]
        n543 = call <vilib>:"Rotation2d_CreateAngle.vi"("Angle"=w957) -> ("ROTATION"=w894:T15)  [unwired: 10 in]
        n544 = call <vilib>:"Rotation2d_GetDegrees.vi"("in ROTATION"=w894) -> ("AngleDegrees"=w956:dbl)  [unwired: 10 in]
        n545 = call-poly <vilib>:"NT Write Value.vi"("value"=w980, "name"="Shooter/Temp_C AMP") -> ()  [unwired: 9 in, 1 out]
        n546 = call-poly <vilib>:"NT Write Value.vi"("value"=w992, "name"="Shooter/Speed_RPM AMP Act") -> ()  [unwired: 9 in, 1 out]
        n547 = call-poly <vilib>:"NT Write Value.vi"("value"=w906, "name"="Shooter/Temp_C") -> ()  [unwired: 9 in, 1 out]
        n548 = call-poly <vilib>:"NT Write Value.vi"("value"=w904, "name"="Shooter/Speed_RPM Act") -> ()  [unwired: 9 in, 1 out]
        n549 = call-poly <vilib>:"NT Write Value.vi"("value"=w916, "name"="Shooter/Angle_Deg Act Talon") -> ()  [unwired: 9 in, 1 out]
        n550 = call-poly <vilib>:"NT Write Value.vi"("value"=w956, "name"="Shooter/Angle_Deg Act") -> ()  [unwired: 9 in, 1 out]
        n551 = call <vilib>:"WPI_DriverStationGet Alliance Info.vi"() -> ("Alliance"=w827:T24)  [unwired: 6 in, 5 out]
        n552 = call-poly <vilib>:"NT Read Value.vi"("name"="/limelight-shooter/tid") -> ("value"=w809:dbl)  [unwired: 8 in, 2 out]
        n553 = call-poly <vilib>:"NT Read Value.vi"("name"="/limelight-shooter/botpose_targetspace") -> ("value"=w836:dbl[])  [unwired: 8 in, 2 out]
        n554 = Not Equal?(x=w827, y=WPI_DriverStationAllianceInfo."Red") -> (x != y?=w805:bool)
        n555 = Equal?(x=w809, y=3.0) -> (x = y?=w811:bool)
        n556 = Equal?(x=w809, y=8.0) -> (x = y?=w808:bool)
        n557 = call-poly <vilib>:"NT Read Value.vi"("default value"="Stop", "name"="Intake/Trigger Status") -> ("value"=w863:string)  [unwired: 7 in, 2 out]
        n558 = call-poly <vilib>:"NT Read Value.vi"("name"="Intake/All Reverse") -> ("value"=w841:bool)  [unwired: 8 in, 2 out]
        n559 = Or(x=w811, y=w808) -> (x .or. y?=w807:bool)
        n560 = global read "Robot Global Data.vi" "Robot Mode"() -> (w882:T2)
        n561 = Index Array(array=w836) -> (element #1=w830:dbl, element #3=w829:dbl)  [unwired: 3 in, 1 out]
        n562 = Select(t=-0.57, s=w805, f=0.57) -> (s? t:f=w802:dbl)
        n563 = call <vilib>:"WPI_SwitchRefNum Registry Get.vi"("refnum name"="Shooter Limit 1") -> ("error out"=w914:errorcluster, "SwitchDevRef"=w915:T36)  [unwired: 9 in]
        n564 = call <vilib>:"WPI_SwitchRefNum Registry Get.vi"("refnum name"="Shooter Limit 2") -> ("error out"=w892:errorcluster, "SwitchDevRef"=w891:T36)  [unwired: 9 in]
        n565 = call <vilib>:"WPI_SwitchRefNum Registry Get.vi"("refnum name"="Shooter Limit 3") -> ("error out"=w889:errorcluster, "SwitchDevRef"=w890:T36)  [unwired: 9 in]
        n566 = call <vilib>:"WPI_SwitchRefNum Registry Get.vi"("refnum name"="Shooter Limit 4") -> ("error out"=w886:errorcluster, "SwitchDevRef"=w885:T36)  [unwired: 9 in]
        n567 = call-poly <vilib>:"PID Control Input Filter.vi"("input"=w830) -> ("output"=w818:dbl)  [unwired: 4 in]
        n568 = call-poly <vilib>:"PID Control Input Filter.vi"("input"=w829) -> ("output"=w814:dbl)  [unwired: 4 in]
        n569 = call <vilib>:"WPI_SwitchGetLimitValue.vi"("error in (no error)"=w914, "SwitchDevRef"=w915) -> ("Switch Pressed"=w871:bool)  [unwired: 7 in, 2 out]
        n570 = call <vilib>:"WPI_SwitchGetLimitValue.vi"("error in (no error)"=w892, "SwitchDevRef"=w891) -> ("Switch Pressed"=w870:bool)  [unwired: 7 in, 2 out]
        n571 = call <vilib>:"WPI_SwitchGetLimitValue.vi"("error in (no error)"=w889, "SwitchDevRef"=w890) -> ("Switch Pressed"=w869:bool)  [unwired: 7 in, 2 out]
        n572 = call <vilib>:"WPI_SwitchGetLimitValue.vi"("error in (no error)"=w886, "SwitchDevRef"=w885) -> ("Switch Pressed"=w868:bool)  [unwired: 7 in, 2 out]
        n573 = Select(t=w802, s=w807, f=0.0) -> (s? t:f=w817:dbl)
        n574 = Equal?(x=w882, y=WPI_DriverStationRobotMode2."Teleop Disabled") -> (x = y?=w878:bool)
        n575 = Equal?(x=w882, y=WPI_DriverStationRobotMode2."Autonomous Disabled") -> (x = y?=w877:bool)
        n576 = Equal?(x=w882, y=WPI_DriverStationRobotMode2."Test Disabled") -> (x = y?=w876:bool)
        n577 = Equal?(x=w863, y="ToShooter") -> (x = y?=w861:bool)
        n578 = Negate(x=w814) -> (-x=w799:dbl)
        n579 = Add(x=w818, y=w817) -> (x+y=w815:dbl)
        n580 = Build Array(w871, w870, w869, w868) -> (w867:bool[])
        n581 = Compound Arithmetic op=OR(w871, w870, w869, w868) -> (w883:bool)
        n582 = Compound Arithmetic op=OR(w878, w877, w876, w861, w841) -> (w875:bool)
        n583 = Subtract(x=w799, y=0.215) -> (x-y=w801:dbl)
        n584 = case shown="False" w883 {
          tunnel: w875 -> [w1013 _]
          frame False {
            n585 = case shown="True" w1013 {
              frame False {
              }
              frame True {
                n586 = call-poly <vilib>:"NT Write Value.vi"("value"=FALSE, "name"="Shooter/Limited") -> ()  [unwired: 9 in, 1 out]
              }
            }
          }
          frame True {
            n587 = call-poly <vilib>:"NT Write Value.vi"("value"=TRUE, "name"="Shooter/Limited") -> ()  [unwired: 9 in, 1 out]
          }
        }
        n588 = call <vilib>:"Util_CalcDist.vi"("Y"=w799, "X"=w815) -> ("DIST"=w816:dbl)  [unwired: 9 in]
        n589 = Inverse Tangent (2 Input)(1:w799, 2:w815) -> (0:w825:dbl)
        n590 = Inverse Tangent (2 Input)(1:w801, 2:w815) -> (0:w821:dbl)
        n591 = Add(x=w825, y=3.141592653589793) -> (x+y=w826:dbl)
        n592 = Add(x=w821, y=3.141592653589793) -> (x+y=w823:dbl)
        n593 = Select(t=w825, s=w805, f=w826) -> (s? t:f=w824:dbl)
        n594 = Select(t=w821, s=w805, f=w823) -> (s? t:f=w820:dbl)
        n595 = call-poly <vilib>:"NT Write Value.vi"("value"=w867, "name"="Shooter/Limit Switches") -> ()  [unwired: 9 in, 1 out]
        n596 = call <vilib>:"MathUtil_AngleModulus.vi"("InputAngle"=w824) -> ("ModulsAngle"=w835:dbl)  [unwired: 10 in]
        n597 = call <vilib>:"MathUtil_AngleModulus.vi"("InputAngle"=w820) -> ("ModulsAngle"=w831:dbl)  [unwired: 10 in]
        n598 = call-poly <vilib>:"NT Write Value.vi"("value"=w816, "name"="Shooter/Distance_m") -> ()  [unwired: 9 in, 1 out]
        n599 = call-poly <vilib>:"NT Write Value.vi"("value"=w835, "name"="Shooter/Theta") -> ()  [unwired: 9 in, 1 out]
        n600 = call-poly <vilib>:"NT Write Value.vi"("value"=w831, "name"="Shooter/Corrected Theta") -> ()  [unwired: 9 in, 1 out]
        n601 = call <vilib>:"CTRE_Phoenix_MotorControl_RefNumRegistryGet.vi"("refnum name"="Intake L") -> ("error out"=w946:errorcluster, "PhoenixMotorControlDevRef"=w947:T27)  [unwired: 9 in]
        n602 = call <vilib>:"WPI_MotorControlRefNum Registry Get.vi"("refnum name"="Trigger") -> ("error out"=w785:errorcluster, "MotorControlDevRef"=w786:T27)  [unwired: 9 in]
        n603 = call-poly <vilib>:"NT Read Value.vi"("default value"="Stop", "name"="Robot State") -> ("value"=w838:string)  [unwired: 7 in, 2 out]
        n604 = call-poly <vilib>:"CTRE_Phoenix_MotorController_Get_TalonFX.vi"("PhoenixMotorControlDevRef"=w947, "error in"=w946) -> ("Temperature (C)"=w949:dbl)  [unwired: 11 in, 2 out]
        n605 = call-poly <vilib>:"CTRE_Phoenix_MotorController_Get_TalonFX.vi"("PhoenixMotorControlDevRef"=w947, "error in"=w946) -> ("Velocity (Raw Sensor Units per 100 ms)"=w968:i32)  [unwired: 10 in, 3 out]
        n606 = call-poly <vilib>:"SPARK Get Encoder Status.vi"("error in (no error)"=w785, "MotorControlDevRef in"=w786) -> ("Sensor Position"=w788:dbl)  [unwired: 6 in, 3 out]
        n607 = call-poly <vilib>:"SPARK Get Encoder Status.vi"("error in (no error)"=w785, "MotorControlDevRef in"=w786) -> ("Sensor Velocity"=w787:dbl)  [unwired: 6 in, 3 out]
        n608 = call <vilib>:"WPI_MotorControlRefNum Registry Get.vi"("refnum name"="Climb R") -> ("error out"=w789:errorcluster, "MotorControlDevRef"=w790:T27)  [unwired: 9 in]
        n609 = call <vilib>:"WPI_MotorControlRefNum Registry Get.vi"("refnum name"="Climb L") -> ("error out"=w793:errorcluster, "MotorControlDevRef"=w794:T27)  [unwired: 9 in]
        n610 = To Double Precision Float(number=w968) -> (double precision float=w964:dbl)
        n611 = case shown="\"Intake Mode\", \"Shoot Mode\"" w838 {
          frame "Intake Mode", "Shoot Mode" {
            n612 = call <vilib>:"CTRE_Phoenix_MotorControl_RefNumRegistryGet.vi"("refnum name"="Shooter Angle") -> ("error out"=w1008:errorcluster, "PhoenixMotorControlDevRef"=w1007:T27)  [unwired: 9 in]
            n613 = call <vilib>:"CTRE_Phoenix_MotorControl_SetNeutralMode.vi"("error in (no error)"=w1008, "Motor Control Neutral Mode"=CTRE_Phoenix_MotorControl_NeutralMode."Override to Coast", "PhoenixMotorControlDevRef"=w1007) -> ()  [unwired: 7 in, 2 out]
          }
          frame "Stop", Default {
            n614 = call <vilib>:"CTRE_Phoenix_MotorControl_RefNumRegistryGet.vi"("refnum name"="Shooter Angle") -> ("error out"=w1012:errorcluster, "PhoenixMotorControlDevRef"=w1011:T27)  [unwired: 9 in]
            n615 = call <vilib>:"CTRE_Phoenix_MotorControl_SetNeutralMode.vi"("error in (no error)"=w1012, "Motor Control Neutral Mode"=CTRE_Phoenix_MotorControl_NeutralMode."Override to Brake", "PhoenixMotorControlDevRef"=w1011) -> ()  [unwired: 7 in, 2 out]
          }
        }
        n616 = call-poly <vilib>:"SPARK Get Device Status.vi"("error in (no error)"=w793, "MotorControlDevRef in"=w794) -> ("Applied Output"=w792:dbl)  [unwired: 6 in, 3 out]
        n617 = call-poly <vilib>:"SPARK Get Device Status.vi"("error in (no error)"=w789, "MotorControlDevRef in"=w790) -> ("Applied Output"=w791:dbl)  [unwired: 6 in, 3 out]
        n618 = Multiply(x=w964, y=10.0) -> (x*y=w963:dbl)
        n619 = call-poly <vilib>:"NT Read Value.vi"("name"="Intake/Gear Ratio") -> ("value"=w944:dbl)  [unwired: 8 in, 2 out]
        n620 = call-poly <vilib>:"NT Read Value.vi"("name"="Intake/Gear Ratio/Trigger") -> ("value"=w941:dbl)  [unwired: 8 in, 2 out]
        n621 = Reciprocal(x=w972) -> (1/x=w973:dbl)
        n622 = Reciprocal(x=w944) -> (1/x=w971:dbl)
        n623 = Reciprocal(x=w941) -> (1/x=w873:dbl)
        n624 = Compound Arithmetic op=MULTIPLY(w963, w973, w971) -> (w974:dbl)
        n625 = Compound Arithmetic op=MULTIPLY(w787, w873) -> (w938:dbl)
        n626 = Compound Arithmetic op=MULTIPLY(w788, w873) -> (w872:dbl)
        n627 = call <vilib>:"Conv_Rotations_Radians.vi"("Rotations"=w974) -> ("Radians"=w967:dbl)  [unwired: 10 in]
        n628 = call-poly <vilib>:"NT Write Value.vi"("value"=w792, "name"="Climb/L Output") -> ()  [unwired: 9 in, 1 out]
        n629 = call-poly <vilib>:"NT Write Value.vi"("value"=w791, "name"="Climb/R Output") -> ()  [unwired: 9 in, 1 out]
        n630 = call <vilib>:"Units_RadiansPerSecondToRotationsPerMinute.vi"("RadiansPerSecond"=w967) -> ("RotationsPerMinute"=w966:dbl)  [unwired: 10 in]
        n631 = call-poly <vilib>:"NT Write Value.vi"("value"=w949, "name"="Intake/Intake L Temp_C") -> ()  [unwired: 9 in, 1 out]
        n632 = call-poly <vilib>:"NT Write Value.vi"("value"=w966, "name"="Intake/Intake L Speed_RPM Act") -> ()  [unwired: 9 in, 1 out]
        n633 = call-poly <vilib>:"NT Write Value.vi"("value"=w938, "name"="Intake/TriggerSpeed_RPM Act") -> ()  [unwired: 9 in, 1 out]
        n634 = call-poly <vilib>:"NT Write Value.vi"("value"=w872, "name"="Intake/TriggerPos_Rotation Act") -> ()  [unwired: 9 in, 1 out]
        n635 = call <vilib>:"WPI_MotorControlRefNum Registry Get.vi"("refnum name"="Climb L") -> ("error out"=w782:errorcluster, "MotorControlDevRef"=w784:T27)  [unwired: 9 in]
        n636 = call <vilib>:"WPI_MotorControlRefNum Registry Get.vi"("refnum name"="Climb R") -> ("error out"=w780:errorcluster, "MotorControlDevRef"=w781:T27)  [unwired: 9 in]
        n637 = call <vilib>:"CTRE_Phoenix_MotorControl_RefNumRegistryGet.vi"("refnum name"="Intake R") -> ("error out"=w858:errorcluster, "PhoenixMotorControlDevRef"=w857:T27)  [unwired: 9 in]
        n638 = call-poly <vilib>:"CTRE_Phoenix_MotorController_Get_TalonFX.vi"("PhoenixMotorControlDevRef"=w857, "error in"=w858) -> ("Temperature (C)"=w855:dbl)  [unwired: 11 in, 2 out]
        n639 = call-poly <vilib>:"CTRE_Phoenix_MotorController_Get_TalonFX.vi"("PhoenixMotorControlDevRef"=w857, "error in"=w858) -> ("Velocity (Raw Sensor Units per 100 ms)"=w849:i32)  [unwired: 10 in, 3 out]
        n640 = call-poly <vilib>:"SPARK Get Encoder Status.vi"("error in (no error)"=w782, "MotorControlDevRef in"=w784) -> ("Sensor Position"=w783:dbl)  [unwired: 6 in, 3 out]
        n641 = call-poly <vilib>:"SPARK Get Encoder Status.vi"("error in (no error)"=w780, "MotorControlDevRef in"=w781) -> ("Sensor Position"=w779:dbl)  [unwired: 6 in, 3 out]
        n642 = To Double Precision Float(number=w849) -> (double precision float=w853:dbl)
        n643 = Multiply(x=w853, y=10.0) -> (x*y=w854:dbl)
        n644 = call <vilib>:"Conv_Rotations_Radians.vi"("Rotations"=w783) -> ("Radians"=w919:dbl)  [unwired: 10 in]
        n645 = call <vilib>:"Conv_Rotations_Radians.vi"("Rotations"=w779) -> ("Radians"=w918:dbl)  [unwired: 10 in]
        n646 = call-poly <vilib>:"NT Read Value.vi"("name"="Climb/Gear Ratio/Climb L") -> ("value"=w929:dbl)  [unwired: 8 in, 2 out]
        n647 = call-poly <vilib>:"NT Read Value.vi"("name"="Climb/Gear Ratio/Climb R") -> ("value"=w936:dbl)  [unwired: 8 in, 2 out]
        n648 = call-poly <vilib>:"NT Read Value.vi"("name"="Intake/Gear Ratio") -> ("value"=w860:dbl)  [unwired: 8 in, 2 out]
        n649 = Divide(x=w921, y=2.0) -> (x/y=w920:dbl)
        n650 = Reciprocal(x=w929) -> (1/x=w926:dbl)
        n651 = Divide(x=w925, y=2.0) -> (x/y=w924:dbl)
        n652 = Reciprocal(x=w936) -> (1/x=w927:dbl)
        n653 = Reciprocal(x=w845) -> (1/x=w844:dbl)
        n654 = Reciprocal(x=w860) -> (1/x=w846:dbl)
        n655 = Compound Arithmetic op=MULTIPLY(w919, w920, w926) -> (w932:dbl)
        n656 = Compound Arithmetic op=MULTIPLY(w918, w924, w927) -> (w933:dbl)
        n657 = Compound Arithmetic op=MULTIPLY(w854, w844, w846) -> (w843:dbl)
        n658 = call <vilib>:"Conv_Rotations_Radians.vi"("Rotations"=w843) -> ("Radians"=w850:dbl)  [unwired: 10 in]
        n659 = call <vilib>:"Units_RadiansPerSecondToRotationsPerMinute.vi"("RadiansPerSecond"=w850) -> ("RotationsPerMinute"=w851:dbl)  [unwired: 10 in]
        n660 = call-poly <vilib>:"NT Write Value.vi"("value"=w932, "name"="Climb/Climb L Positon_mm") -> ()  [unwired: 9 in, 1 out]
        n661 = call-poly <vilib>:"NT Write Value.vi"("value"=w933, "name"="Climb/Climb R Positon_mm") -> ()  [unwired: 9 in, 1 out]
        n662 = call-poly <vilib>:"NT Write Value.vi"("value"=w855, "name"="Intake/Intake R Temp_C") -> ()  [unwired: 9 in, 1 out]
        n663 = call-poly <vilib>:"NT Write Value.vi"("value"=w851, "name"="Intake/Intake R Speed_RPM Act") -> ()  [unwired: 9 in, 1 out]
      }
    }
    frame Enabled {
    }
  }
  n664 = while {
    shift-right: [w1171] -> _
    shift-left: w1 -> [w1171]
    stop <- FALSE stop-if-true
    # "Wait for\nnext interval"
    # "Adjust\nwait time"
    # "Get Time\nUse a single\ntime for all control\nin this loop"
    n665 = call <vilib>:"Util_GetTime.vi"() -> ("FPGA_Time_Seconds"=w1166:dbl)  [unwired: 9 in, 2 out]
    n666 = call <vilib>:"Util_GetTime.vi"() -> ("error out"=w1160:errorcluster, "FPGA_Time_Seconds"=w1163:dbl)  [unwired: 9 in, 1 out]
    n667 = call <vilib>:"Time_WaitAdjust.vi"("PassthroughTime_SEC"=w1166, "MaxAdjustment_MS"=5.0 ("MaxDeviation_MS"), "DesiredLoopTime_MS"=20.0) -> ("AdjustedWaitTime_MS"=w1170:u32, "Offset_MS"=w1167:dbl)  [unwired: 7 in]
    n668 = call "SWERVE_DRIVE_ACT.vi"("Pass_Through_Time"=w1166, "error in"=w1160) -> ("error out"=w1165:errorcluster)  [unwired: 9 in]
    n669 = Wait (ms)(milliseconds to wait=w1170) -> ()  [unwired: 1 out]
    n670 = global write "Robot Global Data.vi" "Ctrl_Loop_Wait_Offset"(w1167) -> ()
    n671 = call <vilib>:"Util_GetTime.vi"("error in (no error)"=w1165) -> ("FPGA_Time_Seconds"=w1164:dbl)  [unwired: 8 in, 2 out]
    n672 = Subtract(x=w1164, y=w1163) -> (x-y=w1162:dbl)
    n673 = call-poly <vilib>:"NT Write Value.vi"("value"=w1162, "name"="Control/Drive Act Loop Elapsed Time") -> ()  [unwired: 9 in, 1 out]
  }
  n674 = while {
    shift-right: [w1181] -> _
    shift-left: w1 -> [w1181]
    stop <- FALSE stop-if-true
    n675 = call <vilib>:"Util_GetTime.vi"() -> ("FPGA_Time_Seconds"=w1180:dbl)  [unwired: 9 in, 2 out]
    n676 = call <vilib>:"Util_GetTime.vi"() -> ("error out"=w1179:errorcluster, "FPGA_Time_Seconds"=w1177:dbl)  [unwired: 9 in, 1 out]
    n677 = call "SWERVE_DRIVE_ACQUIRE.vi"("Pass_Through_Time"=w1180, "error in"=w1179) -> ("error out"=w1173:errorcluster)  [unwired: 9 in]
    n678 = Wait (ms)(milliseconds to wait=u32 20) -> ()  [unwired: 1 out]
    n679 = call <vilib>:"Util_GetTime.vi"("error in (no error)"=w1173) -> ("FPGA_Time_Seconds"=w1178:dbl)  [unwired: 8 in, 2 out]
    n680 = Subtract(x=w1178, y=w1177) -> (x-y=w1176:dbl)
    n681 = call-poly <vilib>:"NT Write Value.vi"("value"=w1176, "name"="Control/Drive Acquire Loop Elapsed Time") -> ()  [unwired: 9 in, 1 out]
  }
  n682 = while {
    shift-right: [w1217] -> _
    shift-left: w1 -> [w1217]
    stop <- FALSE stop-if-true
    w1212 = FALSE  # Write_Traj
    # "Limelight Vision Processing"
    # "Photonvision Vision Processing"
    # "When Write_Traj = False\nset INITIAL_POSE 'A' FGV\nfor smart auto location purpose"
    # "Put the 1st path segement for each Auto Selection"
    n683 = Wait (ms)(milliseconds to wait=u32 20) -> ()  [unwired: 1 out]
    n684 = call-poly <vilib>:"NT Read Value.vi"("name"="Auto Selector" ("Name")) -> ("value"=w1215:string)  [unwired: 8 in, 2 out]
    n685 = case shown="\"Path Demo\"" w1215 {
      tunnel: ["Route Empty.path" ("Trajectory File Name") "Path_Testing_1.path" ("Trajectory File Name") "Route A1 B Path 1.path" ("Trajectory File Name") "Route A1 B Path 1.path" ("Trajectory File Name") "Route A1 R Path 1.path" ("Trajectory File Name") "Route A1 R Path 1.path" ("Trajectory File Name") "Route B2 B Path 1.path" ("Trajectory File Name") "Route B2 B Path 1.path" ("Trajectory File Name") "Route B2 R Path 1.path" ("Trajectory File Name") "Route B2 R Path 1.path" ("Trajectory File Name") "Route C1 B Path 1.path" ("Trajectory File Name") "Route C1 B Path 1.path" ("Trajectory File Name") "Route C1 R Path 1.path" ("Trajectory File Name") "Route C1 R Path 1.path" ("Trajectory File Name") "Route C2 B Path 1.path" ("Trajectory File Name") "Route C2 R Path 1.path" ("Trajectory File Name") "Route A1 R Path 1.path" ("Trajectory File Name") "Route 1 R.path" ("Trajectory File Name") "Route 1 B.path" ("Trajectory File Name") "Route B1 R.path" ("Trajectory File Name") "Route B1 B.path" ("Trajectory File Name")] -> w1213
      frame Default {
      }
      frame "Path Demo" {
      }
      frame "Route A1 Blue" {
      }
      frame "Preload A Blue" {
      }
      frame "Route A1 Red" {
      }
      frame "Preload A Red" {
      }
      frame "Route B2 Blue" {
      }
      frame "Preload B Blue" {
      }
      frame "Route B2 Red" {
      }
      frame "Preload B Red" {
      }
      frame "Route C1 Blue" {
      }
      frame "Preload C Blue" {
      }
      frame "Route C1 Red" {
      }
      frame "Preload C Red" {
      }
      frame "Route C2 Blue" {
      }
      frame "Route C2 Red" {
      }
      frame "Route A1 Red Alter" {
      }
      frame "Route 1 R" {
      }
      frame "Route 1 B" {
      }
      frame "Route B1 Red" {
      }
      frame "Route B1 Blue" {
      }
    }
    n686 = call "SWERVE_TRAJECTORY_READFILE_BEGIN.vi"("Write_Traj"=w1212, "Trajectory File Name"=w1213) -> ()  [unwired: 6 in, 4 out]
    n687 = call-poly <vilib>:"NT Write Value.vi"("value"=w1213, "name"="Initial Path") -> ()  [unwired: 9 in, 1 out]
    n688 = call-poly <vilib>:"NT Read Value.vi"("name"="/limelight-shooter/botpose_wpiblue") -> ("value"=w1210:dbl[])  [unwired: 8 in, 2 out]
    n689 = call-poly <vilib>:"NT Read Value.vi"("name"="/limelight-shooter/targetpose_cameraspace") -> ("value"=w1204:dbl[])  [unwired: 8 in, 2 out]
    n690 = global read "Robot Global Data.vi" "Robot Mode"() -> (w1183:T2)
    n691 = for {
      tunnel: [w1237] -> w1208 mode=indexing if=w1224
      tunnel: [w1236] -> w1209 mode=indexing if=w1224
      tunnel: T39 [{"CameraName"="Camera_Trap", "TRANSLATION3D"={"X"=-0.31, "Y"=-0.276, "Z"=0.165}, "Roll, Pitch, Yaw"={"Roll  Degrees"=0.0, "Pitch  Degrees"=66.9, "Yaw  Degrees"=180.0}}, {"CameraName"="Camera_Left", "TRANSLATION3D"={"X"=-0.464, "Y"=0.273, "Z"=-0.208}, "Roll, Pitch, Yaw"={"Roll  Degrees"=0.0, "Pitch  Degrees"=31.5, "Yaw  Degrees"=-90.0}}] -> [w1235] mode=indexing
      w1224 = FALSE
      # "Don't accept values for now"
      n692 = Unbundle(w1235) -> ("CameraName"=w1243:string, "TRANSLATION3D"=w1242:T38, "Roll, Pitch, Yaw"=w1241:T40)
      n693 = call "PhotonVision_CameraProcess.vi"("Roll, Pitch, Yaw"=w1241, "TRANSLATION3D"=w1242, "CameraName"=w1243) -> ("out CameraToTarget_Pose3d"=w1240:T41, "out RobotPose"=w1237:T17, "Have Multi-tag"=w1226:bool, "CameraName"=w1236:string, "Pose Ambiguity"=w1229:dbl)  [unwired: 4 in]
      n694 = call <vilib>:"Pose3d_getTranslation3d.vi"("in Pose3d"=w1240) -> ("out Translation3d"=w1239:T38)  [unwired: 10 in]
      n695 = call <vilib>:"Translation3d_GetDistance.vi"("other Translation3d"=T38 {"X"=0.0, "Y"=0.0, "Z"=0.0}, "In Translation3d"=w1239) -> ("Distance"=w1234:dbl)  [unwired: 9 in]
      n696 = Less?(x=w1229, y=0.2) -> (x < y?=w1230:bool)
      n697 = Less Or Equal?(x=w1234, y=5.0) -> (x <= y?=w1228:bool)
      n698 = Not Equal To 0?(x=w1234) -> (x != 0?=w1232:bool)
      n699 = Or(x=w1230, y=w1226) -> (x .or. y?=w1225:bool)
      n700 = Or(x=w1226, y=w1228) -> (x .or. y?=w1227:bool)
      n701 = Compound Arithmetic op=AND(w1225, w1227, w1232) -> ()  [unwired: 1 out]
    }
    n702 = Index Array(array=w1204) -> (element #1=w1203:dbl, element #2=w1202:dbl, element #3=w1201:dbl)  [unwired: 4 in, 1 out]
    n703 = case shown="Default" w1183 {
      frame Default {
        n704 = call-poly <vilib>:"NT Write Value.vi"("value"=0.0, "name"="/limelight-shooter/pipeline") -> ()  [unwired: 9 in, 1 out]
      }
      frame "Autonomous Disabled", "Autonomous Enabled" {
        # "0 for Pose Estimation, 1 for Speaker Apriltag only"
        n705 = call-poly <vilib>:"NT Write Value.vi"("value"=1.0, "name"="/limelight-shooter/pipeline") -> ()  [unwired: 9 in, 1 out]
      }
    }
    n706 = Index Array(array=w1210, index #3=5 ("index")) -> (element #1=w1191:dbl, element #2=w1190:dbl, element #3=w1189:dbl)  [unwired: 2 in]
    n707 = call <vilib>:"Translation3d_Create.vi"("Z"=w1201, "Y"=w1202, "X"=w1203) -> ("TRANSLATION3D"=w1200:T38)  [unwired: 8 in]
    n708 = call <vilib>:"Translation3d_GetDistance.vi"("other Translation3d"=T38 {"X"=0.0, "Y"=0.0, "Z"=0.0}, "In Translation3d"=w1200) -> ("Distance"=w1194:dbl)  [unwired: 9 in]
    n709 = call <vilib>:"Pose2d_New.vi"("Heading"=w1189, "Y"=w1190, "X"=w1191) -> ("out POSe"=w1207:T17)  [unwired: 8 in]
    n710 = Less Or Equal?(x=w1194, y=5.0) -> (x <= y?=w1197:bool)
    n711 = Not Equal To 0?(x=w1194) -> (x != 0?=w1196:bool)
    n712 = And(x=w1197, y=w1196) -> (x .and. y?=w1187:bool)
    n713 = case shown="True" w1187 {
      tunnel: w1209 -> [w1276 w1282]
      tunnel: w1208 -> [w1275 w1281]
      tunnel: w1207 -> [_ w1280]
      tunnel: [w1276 w1278] -> w1206
      tunnel: [w1275 w1277] -> w1195
      frame False {
      }
      frame True {
        n714 = Insert Into Array(array=w1282, new element="Limelight" ("new element/subarray")) -> (w1278:string[])  [unwired: 1 in]
        n715 = Insert Into Array(array=w1281, new element=w1280) -> (w1277:T17[])  [unwired: 1 in]
      }
    }
    n716 = Array Size(array=w1195) -> (size(s)=w1186:i32)
    n717 = Not Equal To 0?(x=w1186) -> (x != 0?=w1184:bool)
    n718 = call "Is Value Changed.vim"("value"=w1184) -> ("changed or first call?"=w1185:bool)
    n719 = case shown="True" w1184 {
      tunnel: w1195 -> [_ w1266]
      tunnel: w1206 -> [_ w1261]
      tunnel: w1186 -> [_ w1251]
      tunnel: w1185 -> [_ w1250]
      tunnel: w1184 -> [_ w1249]
      frame False {
        n720 = call-poly <vilib>:"NT Write Value.vi"("value"=dbl[] [], "name"="Vision/Pose") -> ()  [unwired: 9 in, 1 out]
        n721 = call-poly <vilib>:"NT Write Value.vi"("value"=string[] [], "name"="Vision/Cams") -> ()  [unwired: 9 in, 1 out]
      }
      frame True {
        n722 = And(x=w1250, y=w1249) -> (x .and. y?=w1248:bool)
        n723 = for {
          tunnel: w1266 -> [w1274] mode=indexing
          tunnel: [w1268] -> w1254 mode=indexing
          tunnel: [w1269] -> w1253 mode=indexing
          tunnel: [w1270] -> w1252 mode=indexing
          tunnel: w1248 -> [w1267]
          n724 = call <vilib>:"Pose2d_getXYAngle.vi"("in POSE"=w1274) -> ("Angle"=w1271:dbl, "Y"=w1272:dbl, "X"=w1273:dbl)  [unwired: 8 in]
          n725 = call-poly <vilib>:"PID Control Input Filter.vi"("reinitialize? (F)"=w1267, "input"=w1273) -> ("output"=w1268:dbl)  [unwired: 3 in]
          n726 = call-poly <vilib>:"PID Control Input Filter.vi"("reinitialize? (F)"=w1267, "input"=w1272) -> ("output"=w1269:dbl)  [unwired: 3 in]
          n727 = call-poly <vilib>:"PID Control Input Filter.vi"("reinitialize? (F)"=w1267, "input"=w1271) -> ("output"=w1270:dbl)  [unwired: 3 in]
        }
        n728 = To Double Precision Float(number=w1251) -> (double precision float=w1255:dbl)
        n729 = Add Array Elements(numeric array=w1254) -> (sum=w1265:dbl)
        n730 = Add Array Elements(numeric array=w1253) -> (sum=w1264:dbl)
        n731 = Add Array Elements(numeric array=w1252) -> (sum=w1263:dbl)
        n732 = Divide(x=w1265, y=w1255) -> (x/y=w1259:dbl)
        n733 = Divide(x=w1264, y=w1255) -> (x/y=w1258:dbl)
        n734 = Divide(x=w1263, y=w1255) -> (x/y=w1257:dbl)
        n735 = Build Array(w1259, w1258, w1257) -> (w1256:dbl[])
        n736 = call-poly <vilib>:"NT Write Value.vi"("value"=w1261, "name"="Vision/Cams") -> ()  [unwired: 9 in, 1 out]
        n737 = call-poly <vilib>:"NT Write Value.vi"("value"=w1256, "name"="Vision/Pose") -> ()  [unwired: 9 in, 1 out]
      }
    }
    n738 = call-poly <vilib>:"NT Write Value.vi"("value"=w1184, "name"="Vision/HavePose") -> ()  [unwired: 9 in, 1 out]
  }
  n739 = while {
    shift-right: [w1324] -> _
    shift-left: w1 -> [w1324]
    stop <- FALSE stop-if-true
    w1345 = 45.0  # upper limit
    w1346 = -45.0  # lower limit
    w1357 = 1.05  # shotTime
    # "Calculate AIM using Pose Estimator"
    # "Testing Programs here"
    n740 = Wait (ms)(milliseconds to wait=u32 20) -> ()  [unwired: 1 out]
    n741 = call "SWERVE_ODOM_ABS_FGV.vi"() -> ("out SWERVE_DRIVE_POSE_EST2"=w1355:T19)  [unwired: 10 in, 1 out]
    n742 = disable-structure shown="Disabled" {
      frame Disabled {
        n743 = call <vilib>:"Rotation2d_CreateAngle.vi"("Angle"=3.141592653589793) -> ("ROTATION"=w1469:T15)  [unwired: 10 in]
        n744 = call <vilib>:"Rotation2d_RotateBy.vi"("other Rotation"=w1469) -> ("out ROTATION"=w1467:T15)  [unwired: 10 in]
        n745 = call <vilib>:"Pose2d_New_TRRO.vi"("ROTATION"=w1467) -> ()  [unwired: 10 in, 1 out]
      }
      frame Enabled {
      }
    }
    n746 = Unbundle By Name(w1355) -> ("Swerve_Drive_Odom.POSE"=w1326:T17)
    n747 = call-poly <vilib>:"NT Read Value.vi"("name"="Traj/ABS_Odometry") -> ("value"=w1368:dbl[])  [unwired: 8 in, 2 out]
    n748 = disable-structure shown="Disabled" {
      frame Disabled {
        w1443 = 2.0 ("y")
        n749 = global read "SWERVE_DRIVE_GLOBALS.vi" "Chassis vX Speed"() -> (w1450:dbl)
        n750 = global read "SWERVE_DRIVE_GLOBALS.vi" "Chassis vY Speed"() -> (w1449:dbl)
        n751 = call-poly <vilib>:"NT Read Value.vi"("name"="/limelight-shooter/botpose_targetspace") -> ("value"=w1464:dbl[])  [unwired: 8 in, 2 out]
        n752 = Index Array(array=w1464) -> (element #3=w1463:dbl)  [unwired: 3 in, 2 out]
        n753 = Build Array(w1450, w1449) -> (w1462:dbl[])
        n754 = call-poly <vilib>:"PID Control Input Filter.vi"("input"=w1463) -> ("output"=w1452:dbl)  [unwired: 4 in]
        n755 = Square(x=w1462) -> (x^2=w1461:dbl[])
        n756 = Add Array Elements(numeric array=w1461) -> (sum=w1460:dbl)
        n757 = Reciprocal(x=w1452) -> (1/x=w1451:dbl)
        n758 = Square Root(x=w1460) -> (sqrt(x)=w1459:dbl)
        n759 = Multiply(x=w1451, y=2.0) -> (x*y=w1442:dbl)
        n760 = Greater?(x=w1442, y=w1443) -> (0:w1444:bool)
        n761 = call <vilib>:"Util_ApproxEquals.vi"("Tolerance"=0.05, "Value 2"=w1459, "Value 1"=0.0) -> ("ApproxEquals"=w1457:bool)  [unwired: 8 in]
        n762 = Select(t=w1442, s=w1444, f=w1443) -> (s? t:f=w1441:dbl)
        n763 = case shown="True" w1457 {
          tunnel: w1441 -> [w1465 _]
          tunnel: [w1465 0.0] -> w1456
          frame False {
          }
          frame True {
          }
        }
        n764 = call <vilib>:"SlewRateLimiter_Execute.vi"("Enable"=TRUE, "PositiveRate"=2.5, "Input"=w1456) -> ("Output"=w1453:dbl)  [unwired: 7 in, 1 out]
        n765 = call-poly <vilib>:"NT Write Value.vi"("value"=w1453, "name"="OrientationFF") -> ()  [unwired: 9 in, 1 out]
      }
      frame Enabled {
      }
    }
    n766 = disable-structure shown="Disabled" {
      frame Disabled {
        w1429 = 0.02  # dT
        w1430 = 0.02  # dT
        w1435 = 0.02  # dT
        # "Shoot While Moving"
        n767 = global read "SWERVE_DRIVE_GLOBALS.vi" "Chassis vOmega Speed"() -> (w1438:dbl)
        n768 = global read "SWERVE_DRIVE_GLOBALS.vi" "Chassis vX Speed"() -> (w1440:dbl)
        n769 = global read "SWERVE_DRIVE_GLOBALS.vi" "Chassis vY Speed"() -> (w1439:dbl)
        n770 = call "SWERVE_DRIVE_GET_GYRO.vi"() -> ("Gyro Heading Radians"=w1417:dbl)  [unwired: 11 in]
        n771 = Negate(x=w1417) -> (-x=w1416:dbl)
        n772 = call <vilib>:"Rotation2d_CreateAngle.vi"("Angle"=w1416) -> ("ROTATION"=w1437:T15)  [unwired: 10 in]
        n773 = call <vilib>:"ChassisSpeeds_FromFieldRelativeSpeeds.vi"("RobotAngle"=w1437, "Omega"=w1438, "vY"=w1439, "vX"=w1440) -> ("CHASSIS"=w1436:T45)  [unwired: 7 in]
        n774 = call <vilib>:"ChassisSpeeds_GetXYOmega.vi"("CHASSIS"=w1436) -> ("vAngular"=w1419:dbl, "vY"=w1418:dbl, "vX"=w1420:dbl)  [unwired: 8 in]
        n775 = call "SWERVE_ODOM_ABS_FGV.vi"() -> ("out SWERVE_DRIVE_POSE_EST2"=w1428:T19)  [unwired: 10 in, 1 out]
        n776 = Unbundle By Name(w1428) -> ("Swerve_Drive_Odom.POSE"=w1427:T17)
        n777 = Multiply(x=w1420, y=w1429) -> (x*y=w1434:dbl)
        n778 = Multiply(x=w1418, y=w1430) -> (x*y=w1433:dbl)
        n779 = Multiply(x=w1419, y=w1435) -> (x*y=w1432:dbl)
        n780 = call <vilib>:"Twist2d_Create.vi"("dTHETA"=w1432, "dY"=w1433, "dX"=w1434) -> ("TWIST"=w1431:T46)  [unwired: 8 in]
        n781 = call <vilib>:"Pose2d_Exp.vi"("TWIST"=w1431, "POSE"=w1427) -> ("UpdatedPose"=w1426:T17)  [unwired: 9 in]
        n782 = call <vilib>:"Pose2d_getXYAngle.vi"("in POSE"=w1426) -> ("Angle"=w1422:dbl, "Y"=w1423:dbl, "X"=w1424:dbl)  [unwired: 8 in]
        n783 = Build Array(w1424, w1423, w1422) -> (w1421:dbl[])
        n784 = call-poly <vilib>:"NT Write Value.vi"("value"=w1421, "name"="Updated Pose") -> ()  [unwired: 9 in, 1 out]
      }
      frame Enabled {
      }
    }
    n785 = call <vilib>:"WPI_DriverStationGet Alliance Info.vi"() -> ("Alliance"=w1312:T24)  [unwired: 6 in, 5 out]
    n786 = Index Array(array=w1368) -> (element #1=w1367:dbl, element #2=w1366:dbl)  [unwired: 2 in]
    n787 = global read "SWERVE_DRIVE_GLOBALS.vi" "Chassis vOmega Speed"() -> (w1352:dbl)
    n788 = call "SWERVE_DRIVE_GET_GYRO.vi"() -> ("Gyro Heading Radians"=w1329:dbl)  [unwired: 11 in]
    n789 = global read "SWERVE_DRIVE_GLOBALS.vi" "Chassis vX Speed"() -> (w1354:dbl)
    n790 = global read "SWERVE_DRIVE_GLOBALS.vi" "Chassis vY Speed"() -> (w1353:dbl)
    n791 = case shown="\"Red\"" w1312 {
      tunnel: [w1414 w1415] -> w1315
      frame "Red" {
        w1414 = T7 {"X"=16.37, "Y"=5.55}  # Red Speaker
      }
      frame "Blue", Default {
        w1415 = T7 {"X"=0.175, "Y"=5.55}  # Blue Speaker
      }
    }
    n792 = call <vilib>:"Pose2d_getTranslation.vi"("in POSE"=w1326) -> ("outTRANSLATION"=w1342:T7)  [unwired: 10 in]
    n793 = call <vilib>:"Pose2d_getRotation.vi"("in POSE"=w1326) -> ("out ROTATION"=w1341:T15)  [unwired: 10 in]
    n794 = call <vilib>:"Translation2d_Create.vi"("Y"=w1366, "X"=w1367) -> ("TRANSLATION"=w1314:T7)  [unwired: 9 in]
    n795 = call <vilib>:"Transform2d_Create_TransRot.vi"("ROTATION"=w1341, "TRANSLATION"=w1342) -> ("TRANSFORM"=w1340:T47)  [unwired: 9 in]
    n796 = call <vilib>:"Conv_Radians_Deg.vi"("Radians"=w1329) -> ("Degrees"=w1356:dbl)  [unwired: 10 in]
    n797 = call <vilib>:"WPI_DriverStationGet Alliance Info.vi"() -> ("Alliance"=w1350:T24)  [unwired: 6 in, 5 out]
    n798 = Not Equal?(x=w1312, y=WPI_DriverStationAllianceInfo."Red") -> (x != y?=w1311:bool)
    n799 = call <vilib>:"Transform2d_Inverse.vi"("inTRANSFORM"=w1340) -> ("TRANSFORM"=w1339:T47)  [unwired: 10 in]
    n800 = call <vilib>:"Twist2d_Create.vi"("dTHETA"=w1352, "dY"=w1353, "dX"=w1354) -> ("TWIST"=w1325:T46)  [unwired: 8 in]
    n801 = case shown="\"Red\"" w1350 {
      tunnel: [w1470 w1471] -> w1349
      frame "Blue", Default {
        w1470 = T17 {"TRANSLATION"={"X"=0.175, "Y"=5.55}, "ROTATION"={"VALUE"=0.0, "COS"=1.0, "SIN"=0.0}}  # Blue Speaker
      }
      frame "Red" {
        w1471 = T17 {"TRANSLATION"={"X"=16.37, "Y"=5.55}, "ROTATION"={"VALUE"=3.14, "COS"=-1.0, "SIN"=0.0}}  # Red Speaker
      }
    }
    n802 = call <vilib>:"Transform2d_GetXYAngle.vi"("inTRANSFORM"=w1339) -> ("Angle"=w1336:dbl, "Y"=w1337:dbl, "X"=w1338:dbl)  [unwired: 8 in]
    n803 = call <vilib>:"Translation2d_Minus.vi"("other Translation"=w1314, "In Translation"=w1315) -> ("Out Translation"=w1313:T7)  [unwired: 9 in]
    n804 = Select(t=-0.215, s=w1311, f=0.215) -> (s? t:f=w1308:dbl)
    n805 = call <vilib>:"Pose2d_New.vi"("Heading"=w1336, "Y"=w1337, "X"=w1338) -> ("out POSe"=w1335:T17)  [unwired: 8 in]
    n806 = call <vilib>:"Translation2d_GetY.vi"("In Translation"=w1313) -> ("Y"=w1362:dbl)  [unwired: 10 in]
    n807 = call <vilib>:"Translation2d_GetX.vi"("In Translation"=w1313) -> ("X"=w1359:dbl)  [unwired: 10 in]
    n808 = call "getShootingParameters.vi"("shotTime"=w1357, "Turret_Angle_Deg"=w1356, "RobotPose"=w1326, "TurretToField"=w1335, "ShootingGoalPose"=w1349, "RobotVelocity"=w1325, "AllowShootOnMove"=FALSE) -> ("uncompensated_range_m"=w1323:dbl, "effective_yaw_angle_deg"=w1330:dbl, "effective_yaw_feedforward_velocity_deg_s"=w1344:dbl)  [unwired: 4 in, 6 out]
    n809 = In Range and Coerce(upper limit=w1345, x=w1344, lower limit=w1346) -> (coerced(x)=w1343:dbl)  [unwired: 1 out]
    n810 = call <vilib>:"Conv_Deg_Radians.vi"("Degress"=w1330) -> ("Radians"=w1328:dbl)  [unwired: 10 in]
    n811 = Add(x=w1359, y=w1308) -> (x+y=w1358:dbl)
    n812 = Inverse Tangent (2 Input)(1:w1359, 2:w1362) -> (0:w1305:dbl)
    n813 = global read "Robot Global Data.vi" "Robot Mode"() -> (w1322:T2)
    n814 = call <vilib>:"Util_CalcDist.vi"("Y"=w1358, "X"=w1362) -> ("DIST"=w1360:dbl)  [unwired: 9 in]
    n815 = Add(x=3.141592653589793, y=w1305) -> (x+y=w1307:dbl)
    n816 = call-poly <vilib>:"NT Read Value.vi"("default value"="Drive", "name"="Drive/Orient Ctrl Mode") -> ("value"=w1332:string)  [unwired: 7 in, 2 out]
    n817 = call <vilib>:"MathUtil_AngleModulus.vi"("InputAngle"=w1307) -> ("ModulsAngle"=w1364:dbl)  [unwired: 10 in]
    n818 = call <vilib>:"Conv_Deg_Radians.vi"("Degress"=w1343) -> ("Radians"=w1327:dbl)  [unwired: 10 in]
    n819 = Not Equal?(x=w1322, y=WPI_DriverStationRobotMode2."Autonomous Enabled") -> (x != y?=w1319:bool)
    n820 = Equal?(x=w1332, y="Apriltag") -> (x = y?=w1320:bool)
    n821 = call-poly <vilib>:"NT Write Value.vi"("value"=w1328, "name"="Shooter/Corrected Theta_B") -> ()  [unwired: 9 in, 1 out]
    n822 = And(x=w1320, y=w1319) -> (x .and. y?=w1318:bool)
    n823 = Select(t=w1327, s=w1318, f=0.0) -> (s? t:f=w1304:dbl)
    n824 = call-poly <vilib>:"NT Write Value.vi"("value"=w1364, "name"="Shooter/Corrected Theta_A") -> ()  [unwired: 9 in, 1 out]
    n825 = call-poly <vilib>:"NT Write Value.vi"("value"=w1360, "name"="Shooter/Distance_m_A") -> ()  [unwired: 9 in, 1 out]
    n826 = call-poly <vilib>:"NT Write Value.vi"("value"=w1323, "name"="Shooter/Distance_m_B") -> ()  [unwired: 9 in, 1 out]
    n827 = call-poly <vilib>:"NT Write Value.vi"("value"=w1304, "name"="Drive/Orientation FF") -> ()  [unwired: 9 in, 1 out]
    n828 = disable-structure shown="Default" {
      frame condition #0 {
        n829 = call-poly <vilib>:"NT Read Value.vi"("name"="Drive/P6 Str Config") -> ("Variant"=w1382:variant)  [unwired: 9 in, 1 out]
        n830 = call-poly <vilib>:"NT Read Value.vi"("name"="Drive/P6 Drv Config") -> ("Variant"=w1377:variant)  [unwired: 9 in, 1 out]
        n831 = Variant To Data(type=T44 [], Variant=w1382) -> (data=w1380:T44)  [unwired: 1 in, 1 out]
        n832 = Variant To Data(type=T44 [], Variant=w1377) -> (data=w1379:T44)  [unwired: 1 in, 1 out]
        n833 = for {
          tunnel: cluster{string}[] [{"LF Steering"}, {"RF Steering"}, {"LR Steering"}, {"RR Steering"}] ("Steering ref") -> [w1401] mode=indexing
          tunnel: [w1397] -> w1385 mode=indexing
          tunnel: w1380 -> [w1396] mode=indexing
          n834 = Unbundle(w1401) -> (w1400:string)
          n835 = Bundle By Name(cluster=w1396, "Slot0kP"=0.1) -> (w1397:T48)
          n836 = call <vilib>:"Phoenix6_Device_RefNumRegistryGet.vi"("refnum name"=w1400) -> ("error out"=w1398:errorcluster, "data"=w1399:T49)  [unwired: 9 in]
          n837 = call <vilib>:"TalonFXConfigurator.vi"("error in"=w1398, "DeviceConfiguration"=w1397, "DeviceReference"=w1399) -> ()  [unwired: 8 in, 1 out]
        }
        n838 = for {
          tunnel: cluster{string}[] [{"LF Drive"}, {"RF Drive"}, {"LR Drive"}, {"RR Drive"}] ("Steering ref") -> [w1394] mode=indexing
          tunnel: [w1390] -> w1374 mode=indexing
          tunnel: w1379 -> [w1389] mode=indexing
          n839 = Unbundle(w1394) -> (w1393:string)
          n840 = Bundle By Name(cluster=w1389, "Slot0kP"=0.0075) -> (w1390:T48)
          n841 = call <vilib>:"Phoenix6_Device_RefNumRegistryGet.vi"("refnum name"=w1393) -> ("error out"=w1391:errorcluster, "data"=w1392:T49)  [unwired: 9 in]
          n842 = call <vilib>:"TalonFXConfigurator.vi"("error in"=w1391, "DeviceConfiguration"=w1390, "DeviceReference"=w1392) -> ()  [unwired: 8 in, 1 out]
        }
        n843 = To Variant(anything=w1385) -> (Variant=w1384:variant)
        n844 = To Variant(anything=w1374) -> (Variant=w1375:variant)
        n845 = call-poly <vilib>:"NT Write Value.vi"("variant"=w1384, "name"="Drive/P6 Str Config") -> ()  [unwired: 9 in, 1 out]
        n846 = call-poly <vilib>:"NT Write Value.vi"("variant"=w1375, "name"="Drive/P6 Drv Config") -> ()  [unwired: 9 in, 1 out]
      }
      frame condition #1 (active) {
      }
    }
    n847 = disable-structure shown="Disabled" {
      frame Disabled {
        # "Speaker AIM offset"
        n848 = call-poly <vilib>:"NT Read Value.vi"("name"="PID Ctrl") -> ("value"=w1412:dbl[])  [unwired: 8 in, 2 out]
        n849 = Index Array(array=w1412) -> (element #1=w1411:dbl, element #2=w1403:dbl)  [unwired: 3 in, 1 out]
        n850 = In Range and Coerce(upper limit=5.0, x=w1403, lower limit=-5.0) -> (coerced(x)=w1402:dbl)  [unwired: 1 out]
        n851 = In Range and Coerce(upper limit=5.0, x=w1411, lower limit=-5.0) -> (coerced(x)=w1408:dbl)  [unwired: 1 out]
        n852 = call-poly <vilib>:"NT Write Value.vi"("value"=w1408, "name"="Shooter/Angle_Deg Corr") -> ()  [unwired: 9 in, 1 out]
        n853 = call-poly <vilib>:"NT Write Value.vi"("value"=w1402, "name"="Shooter/Fixed Angle_Deg Corr") -> ()  [unwired: 9 in, 1 out]
      }
      frame Enabled {
      }
    }
  }
